vi "ERT_ver2_9_7.vi"() -> ()   [LabVIEW 2023]
uses:
  <vilib>/Utility/error.llb/DialogType.ctl
  <vilib>/Utility/file.llb/Read Delimited Spreadsheet (string).vi
  <vilib>/Utility/file.llb/Read Delimited Spreadsheet (I64).vi
  <vilib>/Utility/config.llb/Read Key (Boolean).vi
  <vilib>/Utility/config.llb/Read Key (U32).vi
  <vilib>/Utility/config.llb/Read Key (Double).vi
  <vilib>/Utility/config.llb/Read Key (I32).vi
  <vilib>/Utility/config.llb/Read Key (String).vi
  <vilib>/Instr/_visa.llb/VISA Configure Serial Port (Instr).vi
  <vilib>/Utility/file.llb/Write Delimited Spreadsheet (I64).vi
  <vilib>/Utility/file.llb/Write Delimited Spreadsheet (string).vi
  <vilib>/Utility/file.llb/Write Delimited Spreadsheet (DBL).vi
  <vilib>/Utility/config.llb/Write Key (Boolean).vi
  <vilib>/Utility/config.llb/Write Key (U32).vi
  <vilib>/Utility/config.llb/Write Key (Double).vi
  <vilib>/Utility/config.llb/Write Key (I32).vi
  <vilib>/Utility/config.llb/Write Key (String).vi
  <vilib>/regexp/Match Regular Expression.xnode
  <instrlib>/Agilent 3446X Series/Agilent 3446X Series.lvlib
  <vilib>/Utility/config.llb/NI_LVConfig.lvlib
panel:
  out "State temp":string
  out "Period for one sample":i32
  out "ESP32 connect?":bool
  out "Current Sense \nResitance Array":dbl[](array[numeric])=[1.0032214, 1.00250644, 1.00234822, 1.0040944, 1.0017711, 1.00229431, 1.00344206, 1.00482066, 1.00381056, 1.00290978, 1.00333016, 1.00367587]
  out "channel count":i32
  out "State":string
  in  "Leave":bool
  in  "Tab Control":T1(tab)
  in  "Refresh":bool
  in  "DMM VISA":refnum<visa-resource-name> caption="DMM (34465A,34470A)"
  in  "ESP32 VISA":refnum<visa-resource-name> caption="ESP32"
  in  "Tab_Current Mode":T2(tab)
  in  "Current Set":u8[][](array[numeric])
  in  "Upload\nCurrent\nSet \nMode":bool
  in  "Current Set Mode":string[][](array[string])
  in  "Break Period Multipier":dbl=8.0
  in  "Insert\nBreak":bool
  in  "Inverse\nPolarity":bool=TRUE
  in  "Electrode number, N":u16=8
  in  "Array Mode":u16(ring) items=["None", "Gradient + Dipole dipole", "Gradient", "Dipole Dipole", "Schlumberger"]
  in  "Upload\nArray":bool
  in  "Only Use Last Value?":bool=TRUE
  in  "Current Channel":string
  in  "Current Mode":u8[][](array[numeric])=[[1, 2, 0, 0, 0, 0, 0, 0], [2, 1, 0, 0, 0, 0, 0, 0], [0, 0, 1, 2, 0, 0, 0, 0], [0, 0, 2, 1, 0, 0, 0, 0], [0, 0, 0, 0, 1, 2, 0, 0], [0, 0, 0, 0, 2, 1, 0, 0], [0, 0, 0, 0, 0, 0, 1, 2], [0, 0, 0, 0, 0, 0, 2, 1]]
  in  "Clear Current Mode":bool
  in  "Waiting\nTime":u32=100 caption="Waiting Time(mS)"
  in  "Sample Mode":u16(ring) items=["Normal", "Interlanced", "Serial", "Seperated Serial"]
  in  "Sample Number":i32=4
  in  "Switch On Time":u8=100 caption="Switch On Time(uS)"
  in  "Switch Off Time":u8=100 caption="Switch Off Time(uS)"
  in  "safe Mode?":bool=TRUE
  in  "PSU Buffer Time":u32=100 caption="PSU Buffer\nTime (ms)"
  in  "Save\nRaw Data":bool=TRUE
  in  "PSU Enable":bool
  in  "Output Max Current":dbl=0.1 caption="Max Current"
  in  "Output Max Voltage":dbl=100.0 caption="Max Voltage"
  in  "Measure\nMax Voltage":dbl=100.0
  in  "Current period":u32=2000
  in  "Scan Period":u32=100
  in  "Sample Measure\nTime(uS)":i32=100
  in  "Scan Number":u32=10
  in  "Constant Scan Number":bool=TRUE
  in  "Neglect\nTimeout Data":bool=TRUE
  in  "Enable Accurate \nMeasure":bool=TRUE
  in  "Enable DMM\n Relay":bool
  in  "Measure Current \nOnly":bool=TRUE
  in  "Record Accurate \nData Only":bool=TRUE
  in  "Remote\nPSU":bool
  in  "PSU(9184B)":refnum<visa-resource-name>="COM5" caption="PSU (9184B,9185B)"
  in  "Email Setting":T3={"server address"="smtp.gmail.com:587", "from"="ncuccc45002931@gmail.com", "username"="ncuccc45002931", "APP password"="aiwfjsidudnfefes\n", "Receiver Email"="yehtingo@gmail.com", "subject"="ERT_data_", "message"="it worked.", "Attach data?"=TRUE}
  in  "Send data\nAutomatically":bool=TRUE
  in  "Leave Timer":string
  in  "Scan Start Timer":string[](array[string])
  in  "Current min":dbl=0.1
  in  "Voltage min":dbl=0.1
  out "Current channel\nindex":string[](array[string])=["  ", "  "]
  in  "I":bool
  in  "V":bool
  in  "Scan Stop":bool
  in  "Scan start":bool
  out "XY Graph":cluster{dbl[], dbl[]}[](graph)
  in  "plot setting":T4(array[cluster])
  in  "Enable\nPlot":bool=TRUE
  in  "Auto Plot \nCurrent":bool
  in  "Current max":dbl=0.1
  in  "Voltage max":dbl=10.0
  out "Data Directory":path=path "C:/Users/User/Desktop/test.csv"
  out "Time out count:":i32
  in  "Data Directory":bool
  out "PSU V":string
  out "PSU I":string
  in  "Measured Current Sense Resistivity":i32[](listbox)
  in  "Update Resistivity":bool
  in  "Calibrate start":bool
  in  "Calibrate Stop":bool
  in  "Current Sense Resistivity List":i32[](listbox) caption="Current Sense Resistivity"
  out "Measured Current Sense \nResitance Array":dbl[](array[numeric])=[1.0032214, 1.00250644, 1.00234822, 1.0040944, 1.0017711, 1.00229431, 1.00344206, 1.00482066, 1.00381056, 1.00290978, 1.00333016, 1.00367587]
  in  "Wait Current Stable Period":i32=500
  in  "Resistance Test":i32[](listbox)
  in  "Resistance Test start":bool
  in  "Resistance Test Stop":bool
  in  "External\nPSU":bool
  in  "Tab Control 2":enum32{"R2 Format Covert"}(tab)
  in  "Conver Type:":T5(radio)
  in  "Original Data path":path
  in  "R2 format covert":bool
  in  "Modified Data path":path
  in  "R2 format_Scan number":i32=10 caption="Scan number"
  in  "Current set number in one current mode":i32=48 caption="Current Mode Number in One Current Set"
  out "concatenated string 3":string caption="concatenated string"
  # "W."
  # "No."
  # "Ch."
  # "No."
  # "Ch."
  # "No."
  # "Ch."
  # "min"
  # "min"
  # "+ channel:"
  # "¡V   channel:"
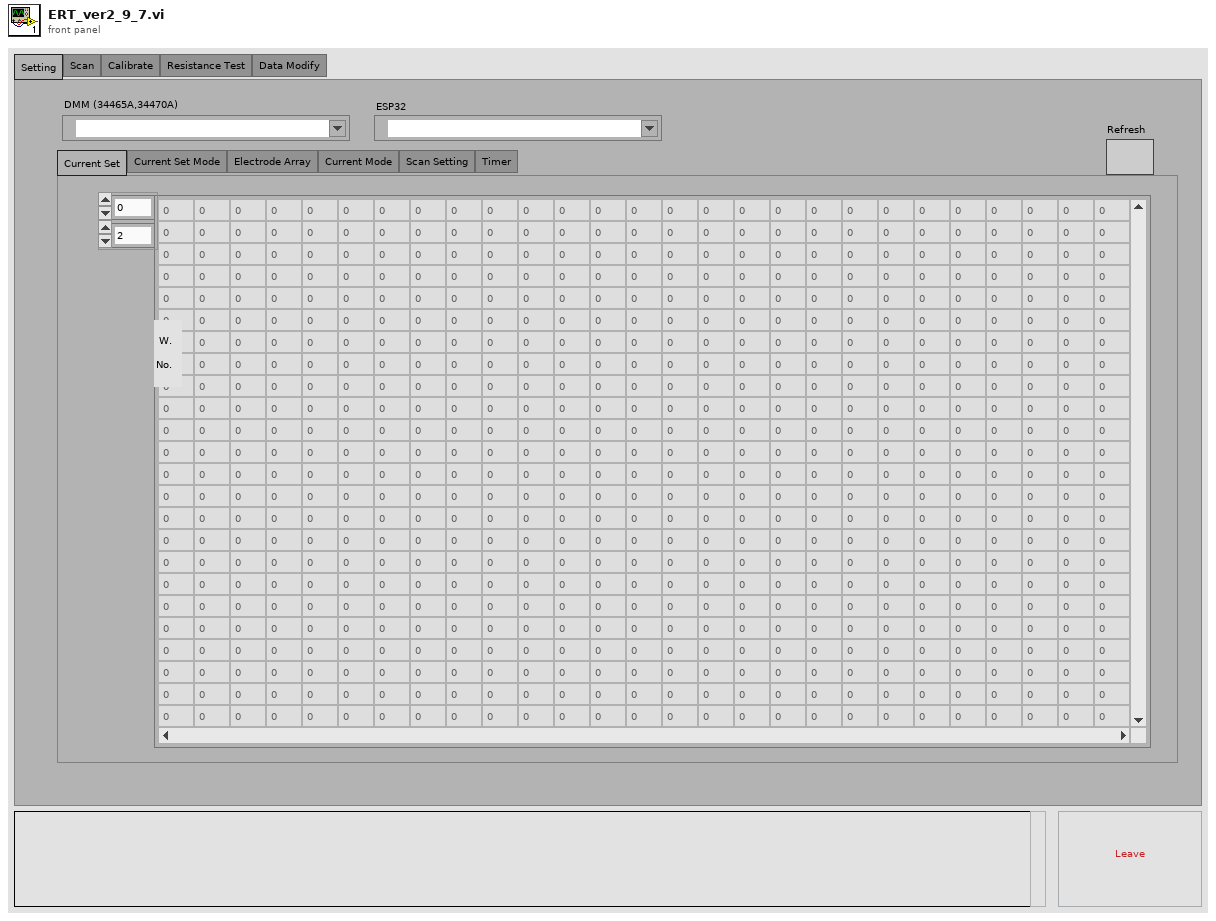
[diagram p1: front panel]
types:
  T1 = enum32{"Setting", "Scan", "Calibrate", "Resistance Test", "Data Modify"}
  T2 = enum32{"Current Set", "Current Set Mode", "Electrode Array", "Current Mode", "Scan Setting", "Timer"}
  T3 = cluster{"server address":string, "from":string, "username":string, "APP password":string, "Receiver Email":string, "subject":string, "message":string, "Attach data?":bool}
  T4 = cluster{"V plot":bool, "I plot":bool, "Plot colour":u32, "Channel name\n":string}[]
  T5 = enum32{"Filled", "Filled and splitted", "Regular"}
  T6 = typedef "DialogType.ctl" = u16
  T7 = enum8{"Enabled", "Disabled", "Disabled and Grayed Out"}
  T8 = typedef "NI_LVConfig.lvlib/Config Data RefNum.ctl" = refnum<k1>
  T9 = cluster{"Enable DMM\n Relay":bool, "Measure Current \nOnly":bool, dbl[], i32}
  T10 = cluster{"value":string, "value":string, "value":string, "value":string, "value":string, "value":string, "value":string, "value":bool}
  T11 = cluster{"DMM VISA":refnum<visa-resource-name>, "ESP32 VISA":refnum<visa-resource-name>, "Scan Period":u32, "Current period":u32, "Scan Measure\nTime(uS)":i32, "Measure\nMax Voltage":dbl, "Data Directory":path, "Voltage max":dbl, "Voltage min":dbl, "Current max":dbl, "Current min":dbl, "PSU(9184B)":refnum<visa-resource-name>}
  T12 = cluster{"Remote\nPSU":bool, "PSU(9184B)":refnum<visa-resource-name>, "Output Max Voltage":dbl, "Output Max Current":dbl, "PSU Buffer Time":u32}
  T13 = cluster{"DMM VISA":refnum<visa-resource-name>, "ESP32 VISA":refnum<visa-resource-name>, "Scan Period":u32, "Current period":u32, "Sample Measure\nTime(uS)":i32, "Measure\nMax Voltage":dbl, "Data Directory":path, "Voltage max":dbl, "Voltage min":dbl, "Current max":dbl, "Current min":dbl, "PSU(9184B)":refnum<visa-resource-name>}
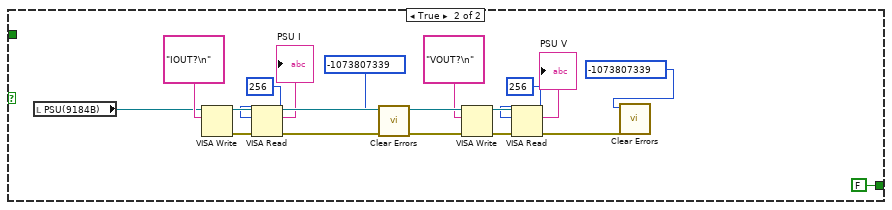
[diagram p3: hidden frame]
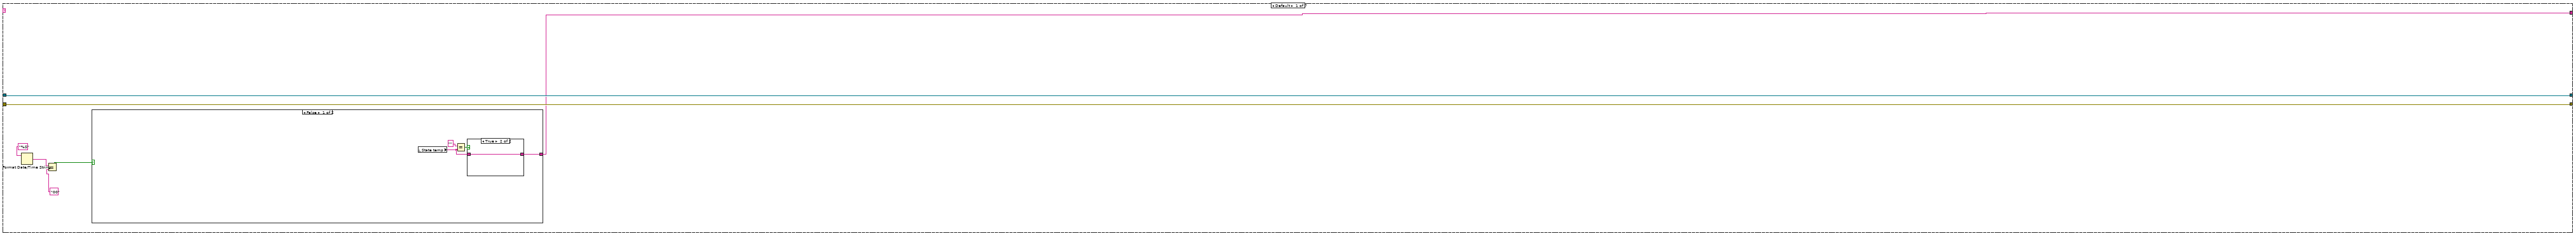
[diagram p4: hidden frame]
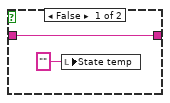
[diagram p5: hidden frame]
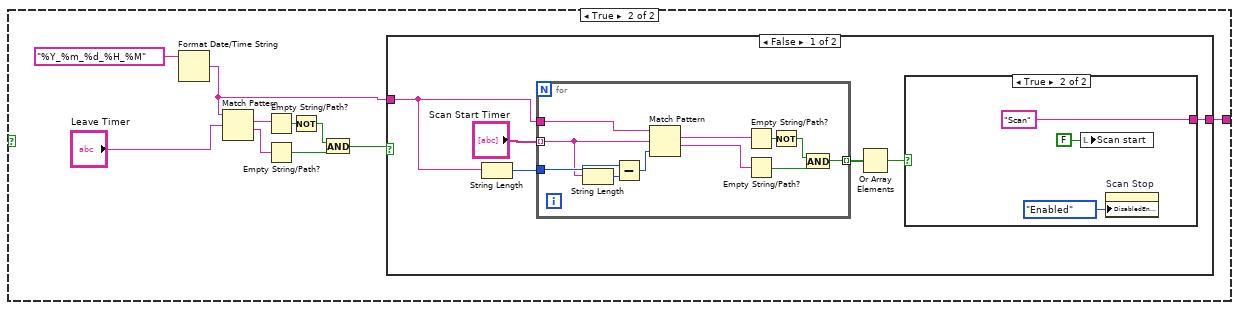
[diagram p6: hidden frame]
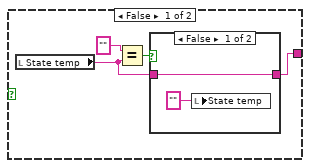
[diagram p7: hidden frame]
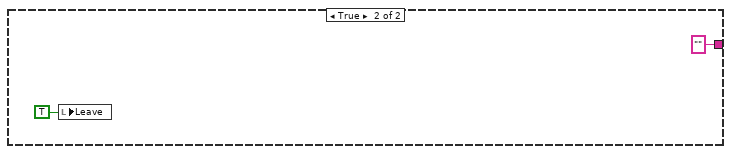
[diagram p9: hidden frame]
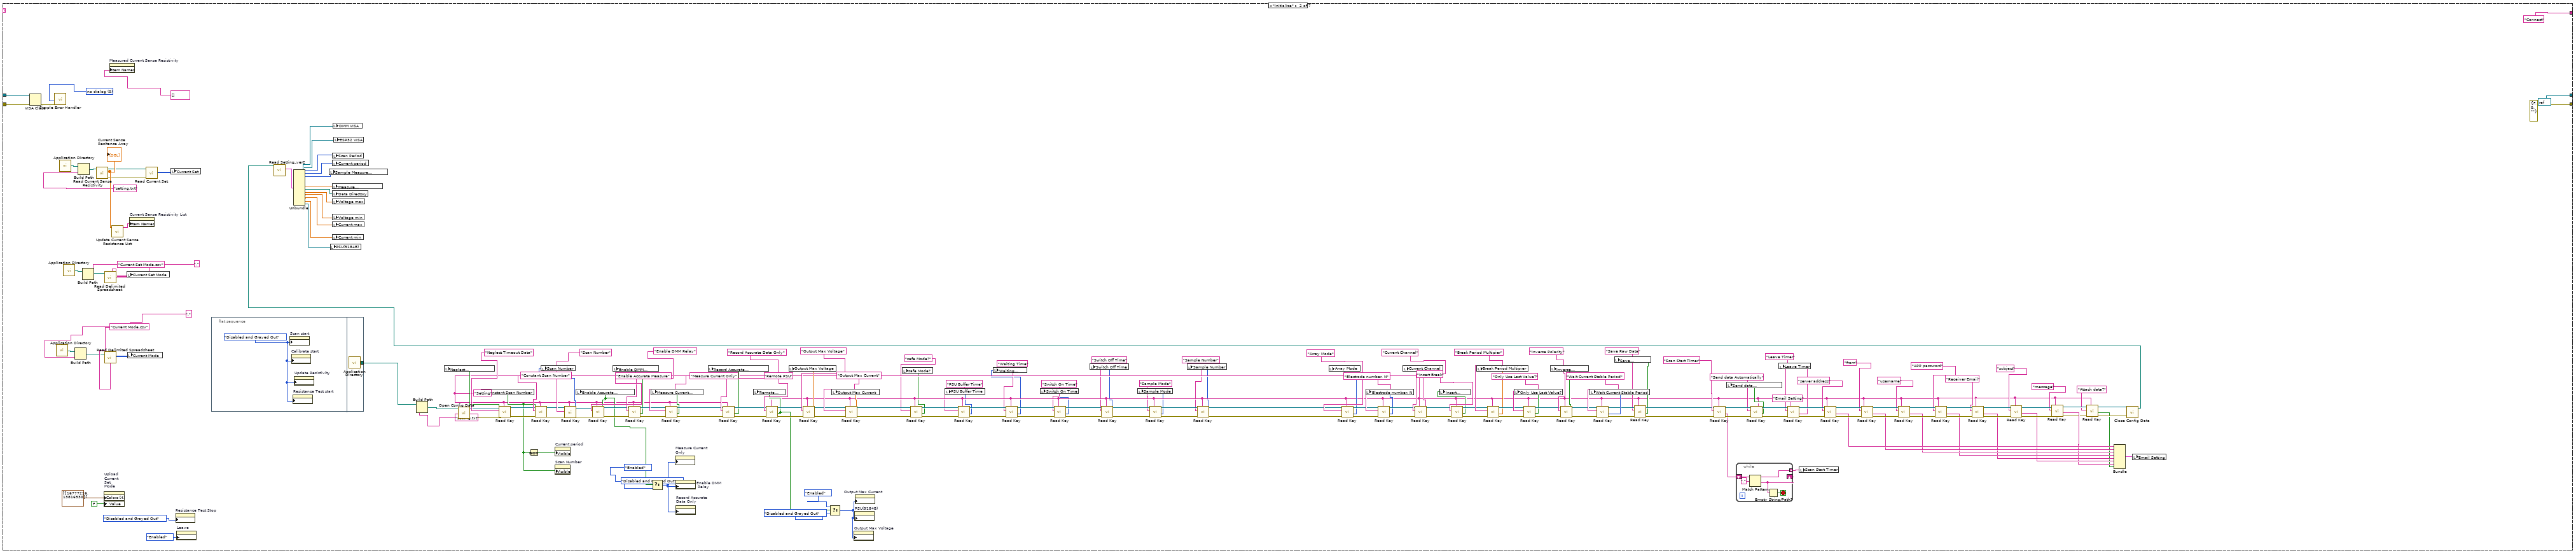
[diagram p10: hidden frame]
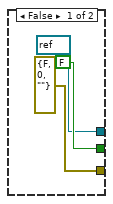
[diagram p11: hidden frame]
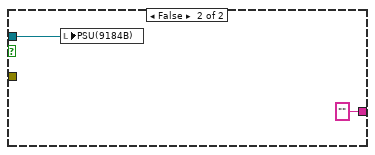
[diagram p12: hidden frame]
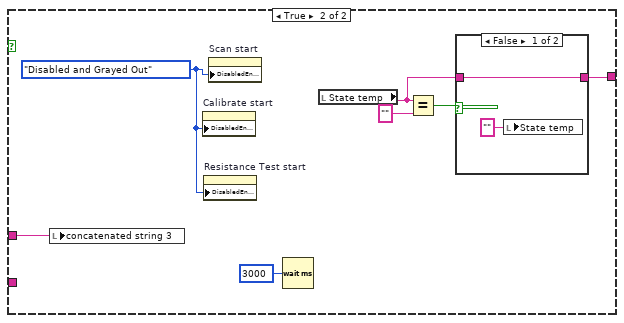
[diagram p13: hidden frame]
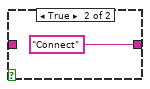
[diagram p14: hidden frame]
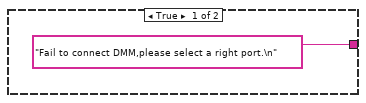
[diagram p15: hidden frame]
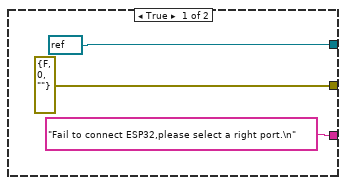
[diagram p16: hidden frame]
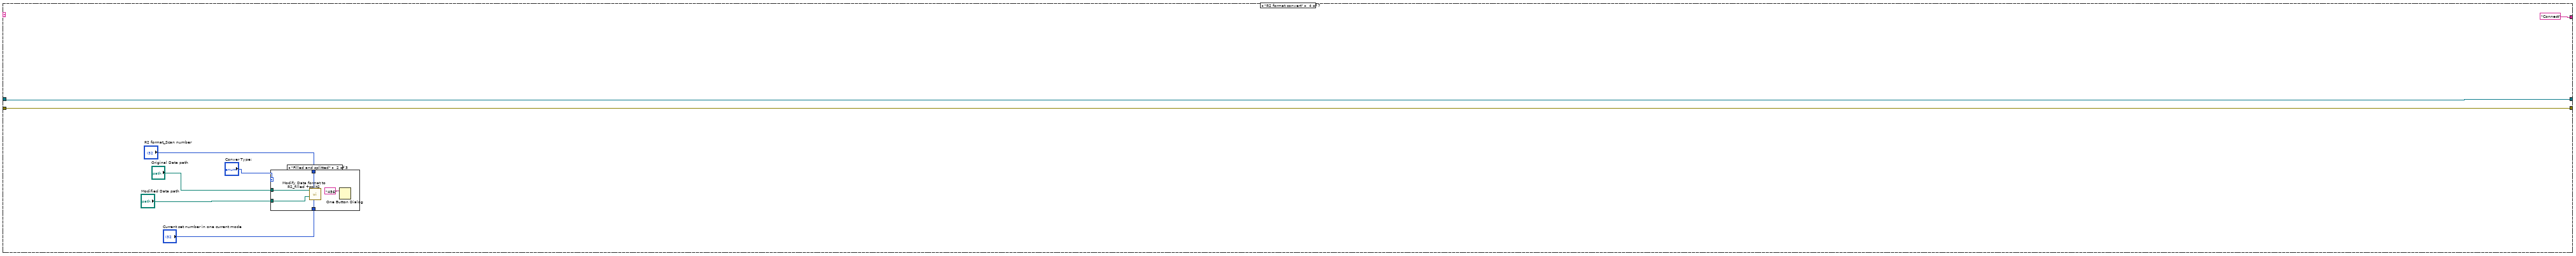
[diagram p17: hidden frame]
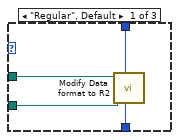
[diagram p18: hidden frame]
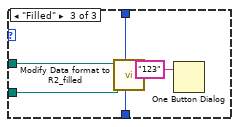
[diagram p19: hidden frame]
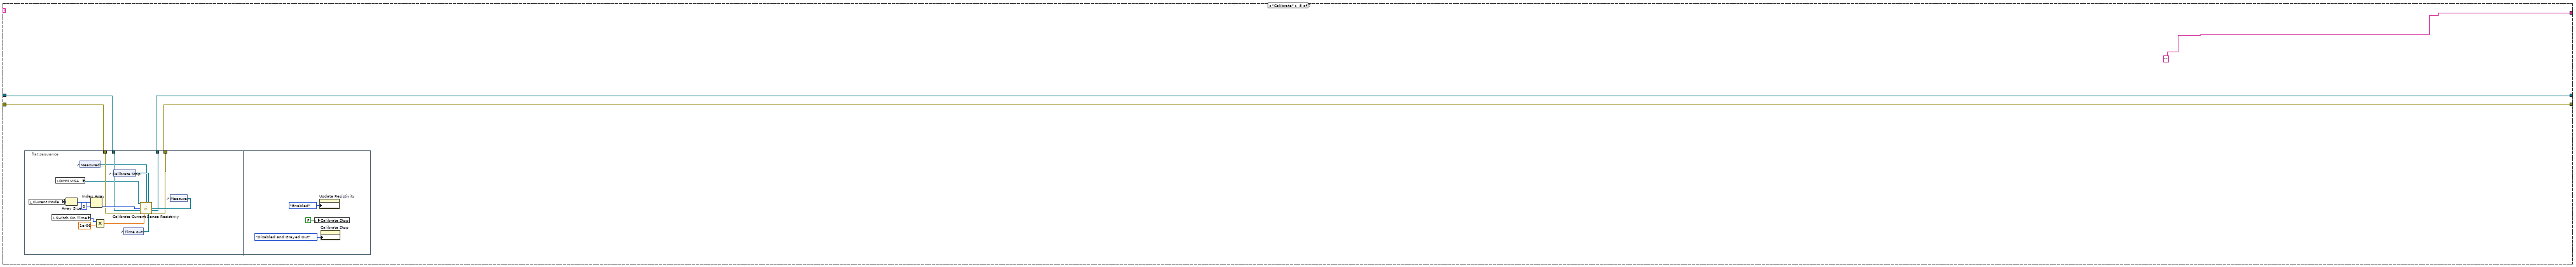
[diagram p20: hidden frame]
diagram:
  w2 = T6 0 items=["no dialog", "OK message", "continue or stop message", "OK message + warnings", "continue/stop + warnings"] ("type of dialog (OK msg:1)")
  # "Oscilloscope mode?"
  # "2_9 2024/1/18\n1. add Oscilloscope mode\n2. add command 'L' to turn\nESP32 into high Impedance\nso it can be parallel with other\ndevice."
  # "2_8 2024/1/9\n1. enable setting switch on \n,off time  and trigger time\n2.. add \"super sample\""
  # "2_7 2024/1/2\n1. add safe PSU mode\n(turn off output of PSU while switching \ncurrent mode)"
  # "ver2_6\n1. add email"
  # "ver2_5 2023/12/19\n1. add scan timer"
  # "ver2_4 2023/12/14\n1.add reconnect when timeout count\nreach 10000"
  # "ver2_3 2023/12/5\n1.updata modify after ver16\n2.add resistance test by DMM"
  # "Board ver2.\nconnect Vpsu from DMM+ to DMM-"
  # "Board ver1."
  # "ver16 2023/08/02\n1. PSU(9184B) connect (optionnal)"
  # "ver15 2023/07/31\n1. Connect COM before scan.\n2. add \"Test\" procedure"
  # "ver14 2023/06/28\n1. add scan mode \"constant scan number\"\n2. add option neglect timeout data\n3. option that modify to R2 format in the end\n4. add option to plot specific  min value"
  # "ver13 2023/06/17\n1.display current channel\nwhile scanning\n2. modify current mode in data when\nfinishing the scan"
  # "try timeout minimum\nwill the timeout in scan\nbe shorter?\nor just set this value to \nscan period minus 10?"
  # "ver12 2023/06/13\n1. main system\n2.edit current mode\n3. measure current with calbrated\ncurrent sense resistor\n4.  add command 's' before scan"
  # "ver11 2023/06/11\n1. record accurate measure only\n2. measure accurate current only"
  # "ver10 2023/06/06\n1.combine subVI and ploting\n2.set plot interpolation to 2 just like default,\nor it will causing more than 50mS when\nX scale change with 64 channels, rather than\n6mS, I think that is some kind of bug in\nlabview.\n3.because of previous changing, I need to \nrecord time \"after\" finising measure, so it can\nproperly display how long it take to finish\naccurate measure.\n4.save data when data index is between 2~3\nplot width"
  n1 = local read "Current Mode"() -> (w21:u8[][])
  n2 = local write "Leave"(FALSE ("Leave")) -> ()
  n3 = Array Size(array=w21) -> (size(s)=w20:i32[])
  n4 = Index Array(array=w20, index=0) -> (element=→"channel count":i32)
  n5 = local write "ESP32 connect?"(FALSE ("ESP32 connect?")) -> ()
  n6 = control-ref of="plot setting"() -> (w23:refnum<vi>)
  n7 = control-ref of="XY Graph"() -> (w22:refnum<vi>)
  n8 = while {
    tunnel: w23 -> [w26]
    tunnel: w22 -> [w25]
    stop <- w27 stop-if-true
    n9 = event shown="[1] \"Leave\": Value Change" {
      selector: _ -> [_ _ _ _ _ _ _ _ _ _ _ _ _ _ _ _ _ _ _ _ _ _ _ _ _ _ _ _ _ _ _ _ _ _ _ _ _ _ _ _ _]
      dyn-events: _ -> [_ _ _ _ _ _ _ _ _ _ _ _ _ _ _ _ _ _ _ _ _ _ _ _ _ _ _ _ _ _ _ _ _ _ _ _ _ _ _ _ _]
      timeout: 1000 -> [_ _ _ _ _ _ _ _ _ _ _ _ _ _ _ _ _ _ _ _ _ _ _ _ _ _ _ _ _ _ _ _ _ _ _ _ _ _ _ _ _]
      tunnel: [w28 w32 _ _ _ _ _ _ _ _ _ _ _ _ _ _ _ _ _ _ _ _ _ _ _ _ _ _ _ _ _ _ _ _ _ _ _ _ _ _ _] -> w27
      tunnel: w26 -> [_ _ _ _ _ _ _ _ _ _ _ _ _ _ _ _ _ w160 w166 w170 _ _ _ _ _ _ _ _ _ _ _ _ _ _ _ _ _ _ _ _ _]
      tunnel: w25 -> [_ _ _ _ _ _ _ _ _ _ _ _ _ _ _ _ _ w159 w165 w169 _ w179 w192 w205 w218 _ _ _ _ _ _ _ _ _ _ _ _ _ _ _ _]
      event Timeout {
        n10 = event-data() -> ()  [unwired: 1 in, 3 out]
        n11 = local read "Leave"() -> (w29:bool)
        n12 = local read "State"() -> (w30:string)
        n13 = Empty String/Path?(string/path=w30) -> (empty?=w31:bool)
        n14 = And(x=w31, y=w29) -> (x .and. y?=w28:bool)
      }
      event "Leave": Value Change {
        n15 = event-data() -> ("NewVal"=w32:bool)  [unwired: 1 in, 5 out]
      }
      event "Scan start": Value Change {
        n16 = event-data() -> ("NewVal"=w33:bool)  [unwired: 1 in, 5 out]
        n17 = case shown="True" w33 {
          frame False {
          }
          frame True {
            n18 = local write "Scan start"(FALSE ("Scan start")) -> ()
            n19 = local write "State temp"("Scan" ("State")) -> ()
            n20 = property on="Scan Stop" class="Bool (strict)"("DisabledEnum"=T7."Enabled" ("Disabled")) -> ()  [unwired: 2 in, 2 out]
          }
        }
      }
      event "Resistance Test start": Value Change {
        n21 = event-data() -> ("NewVal"=w37:bool)  [unwired: 1 in, 5 out]
        n22 = case shown="True" w37 {
          frame False {
          }
          frame True {
            n23 = local read "External\nPSU"() -> (w38:bool)
            n24 = case shown="True" w38 {
              tunnel: ["Resistance Test" ("State") w51] -> w39
              frame False {
              }
              frame True {
                n25 = local read "Remote\nPSU"() -> (w49:bool)
                n26 = Two Button Dialog(message="WARNING!!!!!\nMake sure  \"Measure max voltage\" in \"Scan Setting\"\nis higher than the voltage output from PSU,\nor you might damage your DMM.", 1:"Yes, I certainly have." ("T button name (\"OK\")"), 2:"Not Sure, check again" ("F button name (\"Cancel\")")) -> (T button?=w45:bool)
                n27 = Not(x=w45) -> (.not. x?=w44:bool)
                n28 = And(x=w49, y=w44) -> (x .and. y?=w46:bool)
                n29 = case shown="True" w46 {
                  tunnel: [FALSE ("T button?") w57] -> w47
                  frame False {
                  }
                  frame True {
                    n30 = local read "Output Max Voltage"() -> (w61:dbl)
                    n31 = Number To Decimal String(number=w61) -> (decimal integer string=w62:string)  [unwired: 1 in]
                    n32 = Concatenate Strings("WARNING!!!!!\nMake sure your loading can endure\n\"Max Voltage\" output( " ("message"), w62, " V)from PSU in \"Scan Setting " ("message")) -> (w58:string)
                    n33 = Two Button Dialog(message=w58, 1:"Yes, I certainly have." ("T button name (\"OK\")"), 2:"Not Sure, check again" ("F button name (\"Cancel\")")) -> (T button?=w57:bool)
                  }
                }
                n34 = Or(x=w45, y=w47) -> (x .or. y?=w48:bool)
                n35 = Select(t="" ("f"), s=w48, f="Resistance Test" ("State")) -> (s? t:f=w51:string)
              }
            }
            n36 = local write "Resistance Test Stop"(FALSE ("Resistance Test Stop")) -> ()
            n37 = property on="Resistance Test Stop" class="Bool (strict)"("DisabledEnum"=T7."Enabled" ("Disabled")) -> ()  [unwired: 2 in, 2 out]
            n38 = local write "Resistance Test start"(FALSE ("Scan start")) -> ()
            n39 = local write "State temp"(w39) -> ()
          }
        }
      }
      event "Remote\nPSU": Value Change {
        n40 = event-data() -> ("NewVal"=w68:bool)  [unwired: 1 in, 5 out]
        n41 = Select(t=T7."Enabled" ("Disabled"), s=w68, f=T7."Disabled and Grayed Out" ("Disabled")) -> (s? t:f=w66:T7)
        n42 = property on="Output Max Voltage" class="DigNum (strict)"("DisabledEnum"=w66) -> ()  [unwired: 2 in, 2 out]
        n43 = property on="PSU(9184B)" class="VISAName"("DisabledEnum"=w66) -> ()  [unwired: 2 in, 2 out]
        n44 = property on="Output Max Current" class="DigNum (strict)"("DisabledEnum"=w66) -> ()  [unwired: 2 in, 2 out]
        n45 = local write "State"("Connect" ("State")) -> ()
      }
      event "R2 format covert": Value Change {
        n46 = event-data() -> ("NewVal"=w70:bool)  [unwired: 1 in, 5 out]
        n47 = case shown="True" w70 {
          frame False {
          }
          frame True {
            n48 = flat-sequence {
              frame #0 {
                n49 = local read "Original Data path"() -> (w71:path)
                n50 = Empty String/Path?(string/path=w71) -> (empty?=w72:bool)
                n51 = case shown="True" w72 {
                  frame False {
                  }
                  frame True {
                    n52 = call "File Dialog2"() -> ("selected path"=w73:path)  [unwired: 12 in, 3 out]
                    n53 = Strip Path(path=w73) -> (stripped path=w78:path, name=w77:string)
                    n54 = local write "Original Data path"(w73) -> ()
                    n55 = Concatenate Strings("Modified_" ("string"), w77) -> (w76:string)
                    n56 = Build Path(base path=w78, name or relative path=w76) -> (appended path=w75:path)
                    n57 = local write "Modified Data path"(w75) -> ()
                  }
                }
              }
              frame #1 {
                n58 = local write "R2 format covert"(FALSE ("Scan start")) -> ()
                n59 = local write "State temp"("R2 format convert" ("State")) -> ()
              }
            }
          }
        }
      }
      event "Calibrate start": Value Change {
        n60 = event-data() -> ("NewVal"=w82:bool)  [unwired: 1 in, 5 out]
        n61 = case shown="True" w82 {
          frame False {
          }
          frame True {
            n62 = Two Button Dialog(message="WARNING!!!!!\nMake sure you have replace PSU+ pin to DMM I-\nor your machine might BLOW!!!!!\n", 1:"Yes, I certainly have." ("T button name (\"OK\")"), 2:"Not Sure, check again" ("F button name (\"Cancel\")")) -> (T button?=w89:bool)
            n63 = local write "Calibrate start"(FALSE ("Scan start")) -> ()
            n64 = Select(t="" ("f"), s=w89, f="Calibrate") -> (s? t:f=w90:string)
            n65 = local write "State temp"(w90) -> ()
          }
        }
        n66 = property on="Calibrate Stop" class="Bool (strict)"("DisabledEnum"=T7."Enabled" ("Disabled")) -> ()  [unwired: 2 in, 2 out]
      }
      event "Data Directory": Value Change {
        n67 = event-data() -> ("NewVal"=w91:bool)  [unwired: 1 in, 5 out]
        n68 = case shown="True" w91 {
          frame False {
          }
          frame True {
            n69 = call "File Dialog"() -> ("selected path"=→"Data Directory":path)  [unwired: 12 in, 3 out]
            n70 = local write "Data Directory"(FALSE ("Data Directory")) -> ()
          }
        }
      }
      event "Update Resistivity": Value Change {
        n71 = event-data() -> ("NewVal"=w97:bool)  [unwired: 1 in, 5 out]
        n72 = local read "State"() -> (w99:string)
        n73 = Equal?(x=w99, y="") -> (x = y?=w96:bool)
        n74 = And(x=w96, y=w97) -> (x .and. y?=w95:bool)
        n75 = case shown="True" w95 {
          tunnel: [FALSE ("Scan start") FALSE ("Scan start")] -> w94
          frame False {
          }
          frame True {
            n76 = local read "Measured Current Sense \nResitance Array"() -> (w107:dbl[])
            n77 = property on="Measured Current Sense Resistivity" class="LstBox (strict)"() -> ("Value"=w106:i32[])  [unwired: 2 in, 2 out]
            n78 = for {
              tunnel: w106 -> [w109] mode=indexing
              tunnel: w107 -> [w115]
              tunnel: [w113] -> w104
              n79 = local read "Current Sense \nResitance Array"() -> (w110:dbl[])
              n80 = Index Array(array=w115, index=w109) -> (element=w114:dbl)
              n81 = Array Size(array=w110) -> (size(s)=w111:i32)
              n82 = Less?(x=w109, y=w111) -> (x < y?=w112:bool)
              n83 = case shown="False" w112 {
                tunnel: w110 -> [w121 w127]
                tunnel: w114 -> [w118 w126]
                tunnel: w109 -> [w119 w125]
                tunnel: [w117 w124] -> w113
                frame False {
                  n84 = Increment(x=w119) -> (x+1=w116:i32)
                  n85 = Initialize Array(0.0 ("element"), w116) -> (w122:dbl[])
                  n86 = Replace Array Subset(array=w122, new element=w121) -> (w120:dbl[])  [unwired: 1 in]
                  n87 = Replace Array Subset(array=w120, new element=w118, index=w119) -> (w117:dbl[])
                }
                frame True {
                  n88 = Replace Array Subset(array=w127, new element=w126, index=w125) -> (w124:dbl[])
                }
              }
              n89 = local write "Current Sense \nResitance Array"(w113) -> ()
            }
            n90 = call <vilib>:"Application Directory.vi"() -> ("Application Directory"=w103:path)
            n91 = Build Path(base path=w103, name or relative path="setting.txt") -> (appended path=w101:path)
            n92 = call "Updata Current Sense Resistance List.vi"("Array in"=w104) -> ("Array out"=w105:string[])  [unwired: 10 in]
            n93 = property on="Current Sense Resistivity List" class="LstBox (strict)"("Item Names"=w105) -> ()  [unwired: 2 in, 2 out]
            n94 = call "Write Current Sense Resistivity.vi"("Array"=w104, "configuration file path"=w101) -> ()  [unwired: 8 in, 2 out]
          }
        }
        n95 = local write "Update Resistivity"(w94) -> ()
      }
      event "Current Set": Value Change {
        n96 = event-data() -> ()  [unwired: 1 in, 6 out]
        n97 = property on="Upload\nCurrent\nSet \nMode" class="Bool (strict)"("DisabledEnum"=T7."Enabled" ("Disabled")) -> ()  [unwired: 2 in, 2 out]
      }
      event "Upload\nCurrent\nSet \nMode": Value Change {
        n98 = event-data() -> ("NewVal"=w129:bool)  [unwired: 1 in, 5 out]
        n99 = case shown="True" w129 {
          frame False {
          }
          frame True {
            n100 = local read "Current Set Mode"() -> (w132:string[][])
            n101 = local read "Current Set"() -> (w133:u8[][])
            n102 = call "Updata Current Mode.vi"("Current Set Mode"=w132, "Current Set"=w133) -> ("Current Mode"=w131:u8[][])  [unwired: 9 in]
            n103 = property on="Upload\nCurrent\nSet \nMode" class="Bool (strict)"("Colors [4]"=cluster{u32, u32}[] [{16777216, 13816530}], "Value"=FALSE ("Upload\nCurrent\nSet \nMode")) -> ()  [unwired: 2 in, 2 out]
            n104 = local write "Current Mode"(w131) -> ()
          }
        }
      }
      event "Upload\nArray": Value Change {
        n105 = event-data() -> ("NewVal"=w135:bool)  [unwired: 1 in, 5 out]
        n106 = case shown="True" w135 {
          frame False {
          }
          frame True {
            n107 = One Button Dialog(message="Updata completed") -> ()  [unwired: 1 in, 1 out]
            n108 = call "Create Electrode Array_2.vi"("Current Channel"="Current Channel", "Insert\nBreak"="Insert\nBreak", "Inverse\nPolarity"="Inverse\nPolarity", "Electrode number, N"="Electrode number, N", "Array Mode"="Array Mode") -> ("Current Mode"=w138:u8[][])  [unwired: 6 in]
            n109 = local write "Current Mode"(w138) -> ()
            n110 = property on="Upload\nArray" class="Bool (strict)"("Colors [4]"=cluster{u32, u32}[] [{16777216, 13816530}]) -> ()  [unwired: 2 in, 2 out]
            n111 = local write "Upload\nArray"(FALSE ("Upload\nArray")) -> ()
          }
        }
      }
      event "Break Period Multipier": Value Change {
        n112 = event-data() -> ("NewVal"=w146:dbl)  [unwired: 1 in, 5 out]
        n113 = Absolute Value(x=w146) -> (abs(x)=w145:dbl)
        n114 = local write "Break Period Multipier"(w145) -> ()
      }
      event "Clear Current Mode": Value Change {
        n115 = event-data() -> ("NewVal"=w147:bool)  [unwired: 1 in, 5 out]
        n116 = case shown="True" w147 {
          frame False {
          }
          frame True {
            n117 = local write "Clear Current Mode"(FALSE ("Clear Current Mode")) -> ()
            n118 = local write "Current Mode"(i32[][] [] ("Current Mode")) -> ()
          }
        }
      }
      event "Refresh": Value Change {
        n119 = event-data() -> ("NewVal"=w150:bool)  [unwired: 1 in, 5 out]
        n120 = case shown="True" w150 {
          frame False {
          }
          frame True {
            n121 = local write "State temp"("Initialize" ("State")) -> ()
            n122 = local write "Refresh"(FALSE ("Refresh")) -> ()
          }
        }
      }
      event "Current Set Mode": Value Change {
        n123 = event-data() -> ()  [unwired: 1 in, 6 out]
        n124 = property on="Upload\nCurrent\nSet \nMode" class="Bool (strict)"("Colors [4]"=cluster{u32, u32}[] [{16711680, 13816530}]) -> ()  [unwired: 2 in, 2 out]
      }
      event "Enable Accurate \nMeasure": Value Change {
        n125 = event-data() -> ("NewVal"=w157:bool)  [unwired: 1 in, 5 out]
        n126 = Select(t=T7."Enabled" ("Disabled"), s=w157, f=T7."Disabled and Grayed Out" ("Disabled")) -> (s? t:f=w154:T7)
        n127 = property on="Measure Current \nOnly" class="Bool (strict)"("DisabledEnum"=w154) -> ()  [unwired: 2 in, 2 out]
        n128 = property on="Enable DMM\n Relay" class="Bool (strict)"("DisabledEnum"=w154) -> ()  [unwired: 2 in, 2 out]
        n129 = property on="Record Accurate \nData Only" class="Bool (strict)"("DisabledEnum"=w154) -> ()  [unwired: 2 in, 2 out]
      }
      event "plot setting": Value Change {
        n130 = event-data() -> ("OldVal"=w162:T4, "NewVal"=w161:T4)  [unwired: 1 in, 4 out]
        n131 = local read "channel count"() -> (w158:i32)
        n132 = call "Updata Monitor setting.vi"("Channel number"=w158, "XY Graph REF"=w159, "new plot setting"=w161, "old plot setting"=w162, "plot setting REF"=w160) -> ()  [unwired: 7 in]
      }
      event "V": Value Change {
        n133 = event-data() -> ("NewVal"=w164:bool)  [unwired: 1 in, 5 out]
        n134 = local read "channel count"() -> (w163:i32)
        n135 = call "Plot V.vi"("Channel number"=w163, "XY Graph REF"=w165, "V"=w164, "plot setting REF"=w166) -> ()  [unwired: 8 in]
      }
      event "I": Value Change {
        n136 = event-data() -> ("NewVal"=w168:bool)  [unwired: 1 in, 5 out]
        n137 = local read "channel count"() -> (w167:i32)
        n138 = call "Plot I.vi"("Channel number"=w167, "XY Graph REF"=w169, "V"=w168, "plot setting REF"=w170) -> ()  [unwired: 8 in]
      }
      event "Current Mode": Value Change {
        n139 = event-data() -> ("NewVal"=w172:u8[][])  [unwired: 1 in, 5 out]
        n140 = Array Size(array=w172) -> (size(s)=w174:i32[])
        n141 = Index Array(array=w174, index=0) -> (element=w173:i32)
        n142 = local write "channel count"(w173) -> ()
      }
      event "Current max": Value Change {
        n143 = event-data() -> ("OldVal"=w175:dbl, "NewVal"=w177:dbl)  [unwired: 1 in, 4 out]
        n144 = local read "Current min"() -> (w178:dbl)
        n145 = Less?(x=w178, y=w177) -> (x < y?=w176:bool)
        n146 = case shown="False" w176 {
          tunnel: w179 -> [_ w183]
          tunnel: w177 -> [_ w182]
          tunnel: w175 -> [w181 _]
          frame False {
            n147 = local write "Current max"(w181) -> ()
            n148 = One Button Dialog(message="max value need to be higher than min") -> ()  [unwired: 1 in, 1 out]
          }
          frame True {
            n149 = stacked-sequence {
              tunnel: w183 -> [w184 w187]
              tunnel: w182 -> [_ w186]
              frame #0 {
                n150 = property on="Property Node" class="XYGraph (strict)"(reference=w184, "ActYScl"=1 ("Active Y Scale")) -> ()  [unwired: 1 in, 2 out]
              }
              frame #1 {
                n151 = property on="Property Node" class="XYGraph (strict)"(reference=w187, "YScale.Maximum"=w186) -> ()  [unwired: 1 in, 2 out]
              }
            }
          }
        }
      }
      event "Current min": Value Change {
        n152 = event-data() -> ("OldVal"=w188:dbl, "NewVal"=w189:dbl)  [unwired: 1 in, 4 out]
        n153 = local read "Current max"() -> (w190:dbl)
        n154 = Greater?(x=w190, y=w189) -> (0:w191:bool)
        n155 = case shown="True" w191 {
          tunnel: w192 -> [_ w196]
          tunnel: w189 -> [_ w195]
          tunnel: w188 -> [w194 _]
          frame False {
            n156 = local write "Current min"(w194) -> ()
            n157 = One Button Dialog(message="min value need to be lower than max") -> ()  [unwired: 1 in, 1 out]
          }
          frame True {
            n158 = stacked-sequence {
              tunnel: w196 -> [w197 w200]
              tunnel: w195 -> [_ w199]
              frame #0 {
                n159 = property on="Property Node" class="XYGraph (strict)"(reference=w197, "ActYScl"=1 ("Active Y Scale")) -> ()  [unwired: 1 in, 2 out]
              }
              frame #1 {
                n160 = property on="Property Node" class="XYGraph (strict)"(reference=w200, "YScale.Minimum"=w199) -> ()  [unwired: 1 in, 2 out]
              }
            }
          }
        }
      }
      event "Voltage min": Value Change {
        n161 = event-data() -> ("OldVal"=w201:dbl, "NewVal"=w202:dbl)  [unwired: 1 in, 4 out]
        n162 = local read "Voltage max"() -> (w203:dbl)
        n163 = Greater?(x=w203, y=w202) -> (0:w204:bool)
        n164 = case shown="False" w204 {
          tunnel: w205 -> [_ w209]
          tunnel: w202 -> [_ w208]
          tunnel: w201 -> [w207 _]
          frame False {
            n165 = local write "Voltage min"(w207) -> ()
            n166 = One Button Dialog(message="min value need to be lower than max") -> ()  [unwired: 1 in, 1 out]
          }
          frame True {
            n167 = stacked-sequence {
              tunnel: w209 -> [w210 w213]
              tunnel: w208 -> [_ w212]
              frame #0 {
                n168 = property on="Property Node" class="XYGraph (strict)"(reference=w210, "ActYScl"=0 ("Active Y Scale")) -> ()  [unwired: 1 in, 2 out]
              }
              frame #1 {
                n169 = property on="Property Node" class="XYGraph (strict)"(reference=w213, "YScale.Minimum"=w212) -> ()  [unwired: 1 in, 2 out]
              }
            }
          }
        }
      }
      event "Voltage max": Value Change {
        n170 = event-data() -> ("OldVal"=w214:dbl, "NewVal"=w216:dbl)  [unwired: 1 in, 4 out]
        n171 = local read "Voltage min"() -> (w217:dbl)
        n172 = Less?(x=w217, y=w216) -> (x < y?=w215:bool)
        n173 = case shown="False" w215 {
          tunnel: w218 -> [_ w222]
          tunnel: w216 -> [_ w221]
          tunnel: w214 -> [w219 _]
          frame False {
            n174 = local write "Voltage max"(w219) -> ()
            n175 = One Button Dialog(message="max value need to be higher than min") -> ()  [unwired: 1 in, 1 out]
          }
          frame True {
            n176 = stacked-sequence {
              tunnel: w221 -> [_ w225]
              tunnel: w222 -> [w223 w226]
              frame #0 {
                n177 = property on="Property Node" class="XYGraph (strict)"(reference=w223, "ActYScl"=0 ("Active Y Scale")) -> ()  [unwired: 1 in, 2 out]
              }
              frame #1 {
                n178 = property on="Property Node" class="XYGraph (strict)"(reference=w226, "YScale.Maximum"=w225) -> ()  [unwired: 1 in, 2 out]
              }
            }
          }
        }
      }
      event "Original Data path": Value Change {
        n179 = event-data() -> ("NewVal"=w232:path)  [unwired: 1 in, 5 out]
        n180 = Strip Path(path=w232) -> (stripped path=w231:path, name=w230:string)
        n181 = Concatenate Strings("Modified_" ("string"), w230) -> (w229:string)
        n182 = Build Path(base path=w231, name or relative path=w229) -> (appended path=w227:path)
        n183 = local write "Modified Data path"(w227) -> ()
      }
      event "Constant Scan Number": Value Change {
        n184 = event-data() -> ("NewVal"=w234:bool)  [unwired: 1 in, 5 out]
        n185 = Not(x=w234) -> (.not. x?=w233:bool)
        n186 = property on="Current period" class="DigNum (strict)"("Visible"=w233) -> ()  [unwired: 2 in, 2 out]
        n187 = property on="Scan Number" class="DigNum (strict)"("Visible"=w234) -> ()  [unwired: 2 in, 2 out]
      }
      event "DMM VISA": Value Change {
        n188 = event-data() -> ()  [unwired: 1 in, 6 out]
        n189 = local write "State temp"("Connect" ("State")) -> ()
      }
      event "ESP32 VISA": Value Change {
        n190 = event-data() -> ()  [unwired: 1 in, 6 out]
        n191 = local write "State temp"("Connect" ("State")) -> ()
      }
      event "PSU(9184B)": Value Change {
        n192 = event-data() -> ()  [unwired: 1 in, 6 out]
        n193 = local write "State temp"("Connect" ("State")) -> ()
      }
      event "Array Mode": Value Change {
        n194 = event-data() -> ()  [unwired: 1 in, 6 out]
        n195 = property on="Upload\nArray" class="Bool (strict)"("Colors [4]"=cluster{u32, u32}[] [{16711680, 13816530}]) -> ()  [unwired: 2 in, 2 out]
      }
      event "Electrode number, N": Value Change {
        n196 = event-data() -> ()  [unwired: 1 in, 6 out]
        n197 = property on="Upload\nArray" class="Bool (strict)"("Colors [4]"=cluster{u32, u32}[] [{16711680, 13816530}]) -> ()  [unwired: 2 in, 2 out]
      }
      event "Current Channel": Value Change {
        n198 = event-data() -> ()  [unwired: 1 in, 6 out]
        n199 = property on="Upload\nArray" class="Bool (strict)"("Colors [4]"=cluster{u32, u32}[] [{16711680, 13816530}]) -> ()  [unwired: 2 in, 2 out]
      }
      event "Inverse\nPolarity": Value Change {
        n200 = event-data() -> ()  [unwired: 1 in, 6 out]
        n201 = property on="Upload\nArray" class="Bool (strict)"("Colors [4]"=cluster{u32, u32}[] [{16711680, 13816530}]) -> ()  [unwired: 2 in, 2 out]
      }
      event "Insert\nBreak": Value Change {
        n202 = event-data() -> ()  [unwired: 1 in, 6 out]
        n203 = property on="Upload\nArray" class="Bool (strict)"("Colors [4]"=cluster{u32, u32}[] [{16711680, 13816530}]) -> ()  [unwired: 2 in, 2 out]
      }
      event "Scan Number": Value Change {
        n204 = event-data() -> ("NewVal"=w245:u32)  [unwired: 1 in, 5 out]
        n205 = Less?(x=w245, y=u32 2) -> (x < y?=w243:bool)
        n206 = case shown="True" w243 {
          frame False {
          }
          frame True {
            n207 = local write "Scan Number"(u32 2 ("Scan Number")) -> ()
            n208 = One Button Dialog(message="Scan number need to be at least 2\nor you can use current period mode with 1mS") -> ()  [unwired: 1 in, 1 out]
          }
        }
      }
      event "Scan Start Timer": Value Change {
        n209 = event-data() -> ("NewVal"=w249:string[])  [unwired: 1 in, 5 out]
        n210 = for {
          tunnel: w249 -> [w265] mode=indexing
          shift-right: [w264] -> w248
          shift-left: string[] [] -> [w266]
          shift-right: [w262] -> w259
          shift-left: "" -> [w263]
          n211 = Empty String/Path?(string/path=w265) -> (empty?=w267:bool)
          n212 = case shown="False" w267 {
            tunnel: w266 -> [w273 w275]
            tunnel: w265 -> [w269 _]
            tunnel: [w272 w275] -> w264
            tunnel: w263 -> [w271 w274]
            tunnel: [w270 w274] -> w262
            frame False {
              n213 = Build Array (concatenate)(w273, w269) -> (w272:string[])
              n214 = Concatenate Strings(w271, w269, "," ("string")) -> (w270:string)
            }
            frame True {
            }
          }
        }
        n215 = call <vilib>:"Application Directory.vi"() -> ("Application Directory"=w255:path)
        n216 = Build Path(base path=w255, name or relative path="setting.txt") -> (appended path=w256:path)
        n217 = call <vilib>:"Open Config Data.vi"("configuration file path"=w256) -> ("error out"=w258:errorcluster, "refnum"=w257:T8)  [unwired: 8 in, 1 out]
        n218 = local write "Scan Start Timer"(w248) -> ()
        n219 = call-poly <vilib>:"Write Key.vi"("section"="Setting", "error in (no error)"=w258, "value"=w259, "key"="Scan Start Timer", "refnum"=w257) -> ("error out"=w261:errorcluster, "refnum out"=w260:T8)  [unwired: 4 in, 1 out]
        n220 = call <vilib>:"Close Config Data.vi"("error in (no error)"=w261, "refnum"=w260) -> ()  [unwired: 8 in, 2 out]
      }
      event "Leave Timer": Value Change {
        n221 = event-data() -> ("NewVal"=w276:string)  [unwired: 1 in, 5 out]
        n222 = call <vilib>:"Application Directory.vi"() -> ("Application Directory"=w277:path)
        n223 = Build Path(base path=w277, name or relative path="setting.txt") -> (appended path=w278:path)
        n224 = call <vilib>:"Open Config Data.vi"("configuration file path"=w278) -> ("error out"=w280:errorcluster, "refnum"=w279:T8)  [unwired: 8 in, 1 out]
        n225 = call-poly <vilib>:"Write Key.vi"("section"="Setting", "error in (no error)"=w280, "value"=w276, "key"="Leave Timer", "refnum"=w279) -> ("error out"=w285:errorcluster, "refnum out"=w284:T8)  [unwired: 4 in, 1 out]
        n226 = call <vilib>:"Close Config Data.vi"("error in (no error)"=w285, "refnum"=w284) -> ()  [unwired: 8 in, 2 out]
      }
      event "Send data\nAutomatically": Value Change {
        n227 = event-data() -> ("NewVal"=w286:bool)  [unwired: 1 in, 5 out]
        n228 = call <vilib>:"Application Directory.vi"() -> ("Application Directory"=w290:path)
        n229 = Build Path(base path=w290, name or relative path="setting.txt") -> (appended path=w291:path)
        n230 = call <vilib>:"Open Config Data.vi"("configuration file path"=w291) -> ("error out"=w293:errorcluster, "refnum"=w292:T8)  [unwired: 8 in, 1 out]
        n231 = call-poly <vilib>:"Write Key.vi"("section"="Setting", "error in (no error)"=w293, "value"=w286, "key"="Send data Automatically", "refnum"=w292) -> ("error out"=w295:errorcluster, "refnum out"=w294:T8)  [unwired: 4 in, 1 out]
        n232 = call <vilib>:"Close Config Data.vi"("error in (no error)"=w295, "refnum"=w294) -> ()  [unwired: 8 in, 2 out]
      }
      event "Email Setting": Value Change {
        w298 = "Email Setting" ("section")
        n233 = event-data() -> ("NewVal"=w334:T3)  [unwired: 1 in, 5 out]
        n234 = call <vilib>:"Application Directory.vi"() -> ("Application Directory"=w332:path)
        n235 = Unbundle By Name(w334) -> ("server address"=w309:string, "from"=w308:string, "username"=w307:string, "APP password"=w306:string, "Receiver Email"=w305:string, "subject"=w304:string, "message"=w303:string, "Attach data?"=w297:bool)
        n236 = Build Path(base path=w332, name or relative path="setting.txt") -> (appended path=w333:path)
        n237 = call <vilib>:"Open Config Data.vi"("configuration file path"=w333) -> ("error out"=w329:errorcluster, "refnum"=w330:T8)  [unwired: 8 in, 1 out]
        n238 = call-poly <vilib>:"Write Key.vi"("section"=w298, "error in (no error)"=w329, "value"=w309, "key"="server address", "refnum"=w330) -> ("error out"=w317:errorcluster, "refnum out"=w328:T8)  [unwired: 4 in, 1 out]
        n239 = call-poly <vilib>:"Write Key.vi"("section"=w298, "error in (no error)"=w317, "value"=w308, "key"="from", "refnum"=w328) -> ("error out"=w327:errorcluster, "refnum out"=w326:T8)  [unwired: 4 in, 1 out]
        n240 = call-poly <vilib>:"Write Key.vi"("section"=w298, "error in (no error)"=w327, "value"=w307, "key"="username", "refnum"=w326) -> ("error out"=w325:errorcluster, "refnum out"=w324:T8)  [unwired: 4 in, 1 out]
        n241 = call-poly <vilib>:"Write Key.vi"("section"=w298, "error in (no error)"=w325, "value"=w306, "key"="APP password", "refnum"=w324) -> ("error out"=w323:errorcluster, "refnum out"=w322:T8)  [unwired: 4 in, 1 out]
        n242 = call-poly <vilib>:"Write Key.vi"("section"=w298, "error in (no error)"=w323, "value"=w305, "key"="Receiver Email", "refnum"=w322) -> ("error out"=w321:errorcluster, "refnum out"=w320:T8)  [unwired: 4 in, 1 out]
        n243 = call-poly <vilib>:"Write Key.vi"("section"=w298, "error in (no error)"=w321, "value"=w304, "key"="subject", "refnum"=w320) -> ("error out"=w319:errorcluster, "refnum out"=w318:T8)  [unwired: 4 in, 1 out]
        n244 = call-poly <vilib>:"Write Key.vi"("section"=w298, "error in (no error)"=w319, "value"=w303, "key"="message", "refnum"=w318) -> ("error out"=w299:errorcluster, "refnum out"=w302:T8)  [unwired: 4 in, 1 out]
        n245 = call-poly <vilib>:"Write Key.vi"("section"=w298, "error in (no error)"=w299, "value"=w297, "key"="Attach data?", "refnum"=w302) -> ("error out"=w300:errorcluster, "refnum out"=w301:T8)  [unwired: 4 in, 1 out]
        n246 = call <vilib>:"Close Config Data.vi"("error in (no error)"=w300, "refnum"=w301) -> ()  [unwired: 8 in, 2 out]
      }
      event "Sample Number": Value Change {
        w336 = 50000 ("y")
        # "34465A maximun data number"
        n247 = event-data() -> ("NewVal"=w339:i32)  [unwired: 1 in, 5 out]
        n248 = local read "Current Mode"() -> (w340:u8[][])
        n249 = Array Size(array=w340) -> (size(s)=w341:i32[])
        n250 = Index Array(array=w341, index=0) -> (element=w335:i32)
        n251 = Multiply(x=w339, y=w335) -> (x*y=w338:i32)
        n252 = Greater?(x=w338, y=w336) -> (0:w337:bool)
        n253 = case shown="True" w337 {
          tunnel: w336 -> [_ w345]
          tunnel: w335 -> [_ w344]
          frame False {
          }
          frame True {
            n254 = Quotient & Remainder(x=w345, y=w344) -> (floor(x/y)=w343:i32)  [unwired: 1 out]
            n255 = local write "Sample Number"(w343) -> ()
            n256 = One Button Dialog(message="Data number can't be\nhigher than DMM available ") -> ()  [unwired: 1 in, 1 out]
          }
        }
      }
    }
  }
  n257 = while {
    shift-right: [w350] -> w15
    shift-left: errorcluster {"status"=FALSE, "code"=0, "source"=""} ("error out") -> [w356]
    shift-right: [w351] -> w6
    shift-left: refnum<visa-resource-name> refnum ("VISA Refnum out") -> [w355]
    tunnel: [TRUE] -> w14
    i -> [w347]
    stop <- w353 stop-if-true
    n258 = local read "State"() -> (w354:string)
    n259 = Wait (ms)(milliseconds to wait=u32 10) -> ()  [unwired: 1 out]
    n260 = case shown="\"Connect\"" w354 {
      tunnel: w356 -> [w362 w586 _ w881 w899 w923 w1085]
      tunnel: w355 -> [w363 w587 _ w882 w900 w924 w1086]
      tunnel: [w362 errorcluster {"status"=FALSE, "code"=0, "source"=""} ("error out") w689 w881 w897 w921 w1033] -> w350
      tunnel: [w363 refnum<visa-resource-name> refnum ("VISA Refnum out") w688 w882 w898 w922 w1034] -> w351
      tunnel: [w357 "Connect" ("State") w653 "Connect" ("State") "" ("State") "" ("State") "" ("State")] -> w349
      tunnel: w347 -> [_ _ w650 _ _ _ _]
      frame Default {
        n261 = Format Date/Time String(time format string (%c)="%S") -> (date/time string=w361:string)  [unwired: 2 in]
        n262 = Equal?(x=w361, y="00") -> (x = y?=w358:bool)
        n263 = case shown="False" w358 {
          tunnel: [w365 w380] -> w357
          frame False {
            n264 = local read "State temp"() -> (w364:string)
            n265 = Equal?(x="", y=w364) -> (x = y?=w366:bool)
            n266 = case shown="True" w366 {
              tunnel: [w369 w370] -> w365
              tunnel: w364 -> [w369 w370]
              frame False {
                n267 = local write "State temp"("" ("State temp")) -> ()
              }
              frame True {
              }
            }
          }
          frame True {
            n268 = Format Date/Time String(time format string (%c)="%Y_%m_%d_%H_%M") -> (date/time string=w372:string)  [unwired: 2 in]
            n269 = Match Pattern(string=w372, regular expression="Leave Timer") -> (match substring=w375:string, after substring=w376:string)  [unwired: 1 in, 2 out]
            n270 = Empty String/Path?(string/path=w375) -> (empty?=w377:bool)
            n271 = Empty String/Path?(string/path=w376) -> (empty?=w379:bool)
            n272 = Not(x=w377) -> (.not. x?=w378:bool)
            n273 = And(x=w378, y=w379) -> (x .and. y?=w371:bool)
            n274 = case shown="False" w371 {
              tunnel: [w384 "" ("State")] -> w380
              tunnel: w372 -> [w382 _]
              frame False {
                n275 = String Length(string=w382) -> (length=w381:i32)
                n276 = for {
                  tunnel: "Scan Start Timer" -> [w397] mode=indexing
                  tunnel: [w404] -> w386 mode=indexing
                  tunnel: w382 -> [w401]
                  tunnel: w381 -> [w399]
                  n277 = String Length(string=w397) -> (length=w400:i32)
                  n278 = Subtract(x=w399, y=w400) -> (x-y=w398:i32)
                  n279 = Match Pattern(string=w401, regular expression=w397, offset (0)=w398) -> (match substring=w407:string, after substring=w406:string)  [unwired: 2 out]
                  n280 = Empty String/Path?(string/path=w407) -> (empty?=w405:bool)
                  n281 = Empty String/Path?(string/path=w406) -> (empty?=w402:bool)
                  n282 = Not(x=w405) -> (.not. x?=w403:bool)
                  n283 = And(x=w403, y=w402) -> (x .and. y?=w404:bool)
                }
                n284 = Or Array Elements(Boolean array=w386) -> (logical OR=w385:bool)
                n285 = case shown="True" w385 {
                  tunnel: [w387 "Scan" ("State")] -> w384
                  frame False {
                    n286 = local read "State temp"() -> (w389:string)
                    n287 = Equal?(x="", y=w389) -> (x = y?=w390:bool)
                    n288 = case shown="False" w390 {
                      tunnel: [w392 w393] -> w387
                      tunnel: w389 -> [w392 w393]
                      frame False {
                        n289 = local write "State temp"("" ("State temp")) -> ()
                      }
                      frame True {
                      }
                    }
                  }
                  frame True {
                    n290 = local write "Scan start"(FALSE ("Scan start")) -> ()
                    n291 = property on="Scan Stop" class="Bool (strict)"("DisabledEnum"=T7."Enabled" ("Disabled")) -> ()  [unwired: 2 in, 2 out]
                  }
                }
              }
              frame True {
                n292 = local write "Leave"(TRUE ("Leave")) -> ()
              }
            }
          }
        }
      }
      frame "Initialize" {
        w442 = "Email Setting" ("section")
        w424 = "Setting" ("section")
        w585 = T6 0 items=["no dialog", "OK message", "continue or stop message", "OK message + warnings", "continue/stop + warnings"] ("type of dialog (OK msg:1)")
        n293 = VISA Close(VISA resource name=w587, error in (no error)=w586) -> (error out=w588:errorcluster)
        n294 = call <vilib>:"Simple Error Handler.vi"("type of dialog (OK msg:1)"=w585, "error in (no error)"=w588) -> ()  [unwired: 8 out]
        n295 = call <vilib>:"Application Directory.vi"() -> ("Application Directory"=w602:path)
        n296 = call <vilib>:"Application Directory.vi"() -> ("Application Directory"=w604:path)
        n297 = call <vilib>:"Application Directory.vi"() -> ("Application Directory"=w607:path)
        n298 = Build Path(base path=w602, name or relative path="Current Mode.csv") -> (appended path=w599:path)
        n299 = Build Path(base path=w604, name or relative path="setting.txt") -> (appended path=w600:path)
        n300 = Build Path(base path=w607, name or relative path="Current Set Mode.csv") -> (appended path=w605:path)
        n301 = call "Read Current Sense Resistivity.vi"("configuration file path"=w600) -> ("error out"=w613:errorcluster, "Array"=w617:dbl[], "file path"=w614:path)  [unwired: 8 in]
        "Current Sense \nResitance Array" <- w617
        n302 = property on="Upload\nCurrent\nSet \nMode" class="Bool (strict)"("Colors [4]"=cluster{u32, u32}[] [{16777216, 13816530}], "Value"=FALSE ("Upload\nCurrent\nMode")) -> ()  [unwired: 2 in, 2 out]
        n303 = call-poly <vilib>:"Read Delimited Spreadsheet.vi"("file path (dialog if empty)"=w605, "delimiter (\\t)"="," ("delimiter (\\t)")) -> ("all rows"=w610:string[][])  [unwired: 8 in, 5 out]
        n304 = call-poly <vilib>:"Read Delimited Spreadsheet.vi"("file path (dialog if empty)"=w599, "delimiter (\\t)"="," ("delimiter (\\t)")) -> ("all rows"=w609:i64[][])  [unwired: 8 in, 5 out]
        n305 = property on="Measured Current Sense Resistivity" class="LstBox (strict)"("Item Names"=string[] []) -> ()  [unwired: 2 in, 2 out]
        n306 = call "Updata Current Sense Resistance List.vi"("Array in"=w617) -> ("Array out"=w616:string[])  [unwired: 10 in]
        n307 = local write "Current Set Mode"(w610) -> ()
        n308 = local write "Current Mode"(w609) -> ()
        n309 = property on="Current Sense Resistivity List" class="LstBox (strict)"("Item Names"=w616) -> ()  [unwired: 2 in, 2 out]
        n310 = call "Read Current Set.vi"("configuration file path"=w614, "error in (no error)"=w613) -> ("Current Set"=w612:u8[][])  [unwired: 6 in, 2 out]
        n311 = local write "Current Set"(w612) -> ()
        n312 = property on="Resistance Test Stop" class="Bool (strict)"("DisabledEnum"=T7."Disabled and Grayed Out" ("Disabled")) -> ()  [unwired: 2 in, 2 out]
        n313 = property on="Leave" class="Bool (strict)"("DisabledEnum"=T7."Enabled" ("Disabled")) -> ()  [unwired: 2 in, 2 out]
        n314 = flat-sequence {
          tunnel: [w624] -> w507
          frame #0 {
            w623 = T7."Disabled and Grayed Out" ("Disabled")
            n315 = property on="Scan start" class="Bool (strict)"("DisabledEnum"=w623) -> ()  [unwired: 2 in, 2 out]
            n316 = property on="Calibrate start" class="Bool (strict)"("DisabledEnum"=w623) -> ()  [unwired: 2 in, 2 out]
            n317 = property on="Resistance Test start" class="Bool (strict)"("DisabledEnum"=w623) -> ()  [unwired: 2 in, 2 out]
            n318 = property on="Update Resistivity" class="Bool (strict)"("DisabledEnum"=w623) -> ()  [unwired: 2 in, 2 out]
          }
          frame #1 {
            n319 = call <vilib>:"Application Directory.vi"() -> ("Application Directory"=w624:path)
          }
        }
        n320 = Build Path(base path=w507, name or relative path="setting.txt") -> (appended path=w508:path)
        n321 = call <vilib>:"Open Config Data.vi"("configuration file path"=w508) -> ("error out"=w510:errorcluster, "refnum"=w511:T8)  [unwired: 8 in, 1 out]
        n322 = call-poly <vilib>:"Read Key.vi"("section"=w424, "error in (no error)"=w510, "key"="Neglect Timeout Data" ("Label.Text"), "refnum"=w511) -> ("error out"=w557:errorcluster, "value"=w530:bool, "refnum out"=w558:T8)  [unwired: 4 in, 1 out]
        n323 = local write "Neglect\nTimeout Data"(w530) -> ()
        n324 = call-poly <vilib>:"Read Key.vi"("section"=w424, "error in (no error)"=w557, "key"="Constant Scan Number" ("Label.Text"), "refnum"=w558) -> ("error out"=w515:errorcluster, "value"=w506:bool, "refnum out"=w516:T8)  [unwired: 4 in, 1 out]
        n325 = local write "Constant Scan Number"(w506) -> ()
        n326 = Not(x=w506) -> (.not. x?=w505:bool)
        n327 = property on="Current period" class="DigNum (strict)"("Visible"=w505) -> ()  [unwired: 2 in, 2 out]
        n328 = property on="Scan Number" class="DigNum (strict)"("Visible"=w506) -> ()  [unwired: 2 in, 2 out]
        n329 = call-poly <vilib>:"Read Key.vi"("section"=w424, "error in (no error)"=w515, "key"="Scan Number" ("Label.Text"), "refnum"=w516) -> ("error out"=w513:errorcluster, "value"=w512:u32, "refnum out"=w514:T8)  [unwired: 4 in, 1 out]
        n330 = local write "Scan Number"(w512) -> ()
        n331 = call-poly <vilib>:"Read Key.vi"("section"=w424, "error in (no error)"=w513, "key"="Enable Accurate Measure" ("Label.Text"), "refnum"=w514) -> ("error out"=w555:errorcluster, "value"=w504:bool, "refnum out"=w556:T8)  [unwired: 4 in, 1 out]
        n332 = local write "Enable Accurate \nMeasure"(w504) -> ()
        n333 = call-poly <vilib>:"Read Key.vi"("section"=w424, "error in (no error)"=w555, "key"="Enable DMM Relay" ("Label.Text"), "refnum"=w556) -> ("error out"=w553:errorcluster, "value"=w529:bool, "refnum out"=w554:T8)  [unwired: 4 in, 1 out]
        n334 = local write "Enable DMM\n Relay"(w529) -> ()
        n335 = Select(t=T7."Enabled" ("Disabled"), s=w504, f=T7."Disabled and Grayed Out" ("Disabled")) -> (s? t:f=w584:T7)
        n336 = call-poly <vilib>:"Read Key.vi"("section"=w424, "error in (no error)"=w553, "key"="Measure Current Only" ("Label.Text"), "refnum"=w554) -> ("error out"=w551:errorcluster, "value"=w528:bool, "refnum out"=w552:T8)  [unwired: 4 in, 1 out]
        n337 = local write "Measure Current \nOnly"(w528) -> ()
        n338 = property on="Measure Current \nOnly" class="Bool (strict)"("DisabledEnum"=w584) -> ()  [unwired: 2 in, 2 out]
        n339 = property on="Enable DMM\n Relay" class="Bool (strict)"("DisabledEnum"=w584) -> ()  [unwired: 2 in, 2 out]
        n340 = property on="Record Accurate \nData Only" class="Bool (strict)"("DisabledEnum"=w584) -> ()  [unwired: 2 in, 2 out]
        n341 = call-poly <vilib>:"Read Key.vi"("section"=w424, "error in (no error)"=w551, "key"="Record Accurate Data Only" ("Label.Text"), "refnum"=w552) -> ("error out"=w549:errorcluster, "value"=w527:bool, "refnum out"=w550:T8)  [unwired: 4 in, 1 out]
        n342 = local write "Record Accurate \nData Only"(w527) -> ()
        n343 = call-poly <vilib>:"Read Key.vi"("section"=w424, "error in (no error)"=w549, "key"="Remote PSU" ("Label.Text"), "refnum"=w550) -> ("error out"=w547:errorcluster, "value"=w503:bool, "refnum out"=w548:T8)  [unwired: 4 in, 1 out]
        n344 = local write "Remote\nPSU"(w503) -> ()
        n345 = call-poly <vilib>:"Read Key.vi"("section"=w424, "error in (no error)"=w547, "key"="Output Max Voltage" ("Label.Text"), "refnum"=w548) -> ("error out"=w545:errorcluster, "value"=w526:dbl, "refnum out"=w546:T8)  [unwired: 4 in, 1 out]
        n346 = local write "Output Max Voltage"(w526) -> ()
        n347 = Select(t=T7."Enabled" ("Disabled"), s=w503, f=T7."Disabled and Grayed Out" ("Disabled")) -> (s? t:f=w583:T7)
        n348 = call-poly <vilib>:"Read Key.vi"("section"=w424, "error in (no error)"=w545, "key"="Output Max Current" ("Label.Text"), "refnum"=w546) -> ("error out"=w439:errorcluster, "value"=w525:dbl, "refnum out"=w440:T8)  [unwired: 4 in, 1 out]
        n349 = local write "Output Max Current"(w525) -> ()
        n350 = property on="Output Max Voltage" class="DigNum (strict)"("DisabledEnum"=w583) -> ()  [unwired: 2 in, 2 out]
        n351 = property on="PSU(9184B)" class="VISAName"("DisabledEnum"=w583) -> ()  [unwired: 2 in, 2 out]
        n352 = property on="Output Max Current" class="DigNum (strict)"("DisabledEnum"=w583) -> ()  [unwired: 2 in, 2 out]
        n353 = call-poly <vilib>:"Read Key.vi"("section"=w424, "error in (no error)"=w439, "key"="safe Mode?" ("Label.Text"), "refnum"=w440) -> ("error out"=w437:errorcluster, "value"=w423:bool, "refnum out"=w438:T8)  [unwired: 4 in, 1 out]
        n354 = local write "safe Mode?"(w423) -> ()
        n355 = call-poly <vilib>:"Read Key.vi"("section"=w424, "error in (no error)"=w437, "key"="PSU Buffer Time" ("Label.Text"), "refnum"=w438) -> ("error out"=w435:errorcluster, "value"=w421:u32, "refnum out"=w436:T8)  [unwired: 4 in, 1 out]
        n356 = local write "PSU Buffer Time"(w421) -> ()
        n357 = call-poly <vilib>:"Read Key.vi"("section"=w424, "error in (no error)"=w435, "key"="Waiting Time" ("Label.Text"), "refnum"=w436) -> ("error out"=w433:errorcluster, "value"=w418:u32, "refnum out"=w434:T8)  [unwired: 4 in, 1 out]
        n358 = local write "Waiting\nTime"(w418) -> ()
        n359 = call-poly <vilib>:"Read Key.vi"("section"=w424, "error in (no error)"=w433, "key"="Switch On Time" ("Label.Text"), "refnum"=w434) -> ("error out"=w431:errorcluster, "value"=w416:u32, "refnum out"=w432:T8)  [unwired: 4 in, 1 out]
        n360 = local write "Switch On Time"(w416) -> ()
        n361 = call-poly <vilib>:"Read Key.vi"("section"=w424, "error in (no error)"=w431, "key"="Switch Off Time" ("Label.Text"), "refnum"=w432) -> ("error out"=w429:errorcluster, "value"=w415:u32, "refnum out"=w430:T8)  [unwired: 4 in, 1 out]
        n362 = local write "Switch Off Time"(w415) -> ()
        n363 = call-poly <vilib>:"Read Key.vi"("section"=w424, "error in (no error)"=w429, "key"="Sample Mode" ("Label.Text"), "refnum"=w430) -> ("error out"=w427:errorcluster, "value"=w413:u32, "refnum out"=w428:T8)  [unwired: 4 in, 1 out]
        n364 = local write "Sample Mode"(w413) -> ()
        n365 = call-poly <vilib>:"Read Key.vi"("section"=w424, "error in (no error)"=w427, "key"="Sample Number" ("Label.Text"), "refnum"=w428) -> ("error out"=w425:errorcluster, "value"=w411:i32, "refnum out"=w426:T8)  [unwired: 4 in, 1 out]
        n366 = local write "Sample Number"(w411) -> ()
        n367 = call-poly <vilib>:"Read Key.vi"("section"=w424, "error in (no error)"=w425, "key"="Array Mode" ("Label.Text"), "refnum"=w426) -> ("error out"=w543:errorcluster, "value"=w524:u32, "refnum out"=w544:T8)  [unwired: 4 in, 1 out]
        n368 = local write "Array Mode"(w524) -> ()
        n369 = call-poly <vilib>:"Read Key.vi"("section"=w424, "error in (no error)"=w543, "key"="Electrode number, N" ("Label.Text"), "refnum"=w544) -> ("error out"=w541:errorcluster, "value"=w523:u32, "refnum out"=w542:T8)  [unwired: 4 in, 1 out]
        n370 = local write "Electrode number, N"(w523) -> ()
        n371 = call-poly <vilib>:"Read Key.vi"("section"=w424, "error in (no error)"=w541, "key"="Current Channel" ("Label.Text"), "refnum"=w542) -> ("error out"=w539:errorcluster, "value"=w522:string, "refnum out"=w540:T8)  [unwired: 4 in, 1 out]
        n372 = local write "Current Channel"(w522) -> ()
        n373 = call-poly <vilib>:"Read Key.vi"("section"=w424, "error in (no error)"=w539, "key"="Insert Break" ("Label.Text"), "refnum"=w540) -> ("error out"=w537:errorcluster, "value"=w517:bool, "refnum out"=w538:T8)  [unwired: 4 in, 1 out]
        n374 = local write "Insert\nBreak"(w517) -> ()
        n375 = call-poly <vilib>:"Read Key.vi"("section"=w424, "error in (no error)"=w537, "key"="Break Period Multipier" ("Label.Text"), "refnum"=w538) -> ("error out"=w535:errorcluster, "value"=w521:dbl, "refnum out"=w536:T8)  [unwired: 4 in, 1 out]
        n376 = local write "Break Period Multipier"(w521) -> ()
        n377 = call-poly <vilib>:"Read Key.vi"("section"=w424, "error in (no error)"=w535, "key"="Only Use Last Value?" ("Label.Text"), "refnum"=w536) -> ("error out"=w533:errorcluster, "value"=w520:bool, "refnum out"=w534:T8)  [unwired: 4 in, 1 out]
        n378 = local write "Only Use Last Value?"(w520) -> ()
        n379 = call-poly <vilib>:"Read Key.vi"("section"=w424, "error in (no error)"=w533, "key"="Inverse Polarity" ("Label.Text"), "refnum"=w534) -> ("error out"=w531:errorcluster, "value"=w519:bool, "refnum out"=w532:T8)  [unwired: 4 in, 1 out]
        n380 = local write "Inverse\nPolarity"(w519) -> ()
        n381 = call-poly <vilib>:"Read Key.vi"("section"=w424, "error in (no error)"=w531, "key"="Wait Current Stable Period" ("Label.Text"), "refnum"=w532) -> ("error out"=w458:errorcluster, "value"=w518:u32, "refnum out"=w460:T8)  [unwired: 4 in, 1 out]
        n382 = local write "Wait Current Stable Period"(w518) -> ()
        n383 = call-poly <vilib>:"Read Key.vi"("section"=w424, "error in (no error)"=w458, "key"="Save Raw Data" ("Label.Text"), "refnum"=w460) -> ("error out"=w457:errorcluster, "value"=w455:bool, "refnum out"=w459:T8)  [unwired: 4 in, 1 out]
        n384 = local write "Save\nRaw Data"(w455) -> ()
        n385 = call-poly <vilib>:"Read Key.vi"("section"=w424, "error in (no error)"=w457, "key"="Scan Start Timer", "refnum"=w459) -> ("error out"=w499:errorcluster, "value"=w485:string, "refnum out"=w500:T8)  [unwired: 4 in, 1 out]
        n386 = while {
          shift-right: [w618] -> _
          shift-left: w485 -> [w622]
          tunnel: [w620] -> w484 mode=indexing
          stop <- w619 stop-if-true
          n387 = Match Pattern(string=w622, regular expression=",") -> (before substring=w620:string, after substring=w618:string)  [unwired: 1 in, 2 out]
          n388 = Empty String/Path?(string/path=w618) -> (empty?=w619:bool)
        }
        n389 = call-poly <vilib>:"Read Key.vi"("section"=w424, "error in (no error)"=w499, "key"="Send data Automatically", "refnum"=w500) -> ("error out"=w497:errorcluster, "value"=w482:bool, "refnum out"=w498:T8)  [unwired: 4 in, 1 out]
        n390 = local write "Send data\nAutomatically"(w482) -> ()
        n391 = call-poly <vilib>:"Read Key.vi"("section"=w424, "error in (no error)"=w497, "key"="Leave Timer", "refnum"=w498) -> ("error out"=w495:errorcluster, "value"=w480:string, "refnum out"=w496:T8)  [unwired: 4 in, 1 out]
        n392 = local write "Leave Timer"(w480) -> ()
        n393 = local write "Scan Start Timer"(w484) -> ()
        n394 = call-poly <vilib>:"Read Key.vi"("section"=w442, "error in (no error)"=w495, "key"="server address", "refnum"=w496) -> ("error out"=w493:errorcluster, "value"=w467:string, "refnum out"=w494:T8)  [unwired: 4 in, 1 out]
        n395 = call-poly <vilib>:"Read Key.vi"("section"=w442, "error in (no error)"=w493, "key"="from", "refnum"=w494) -> ("error out"=w491:errorcluster, "value"=w466:string, "refnum out"=w492:T8)  [unwired: 4 in, 1 out]
        n396 = call-poly <vilib>:"Read Key.vi"("section"=w442, "error in (no error)"=w491, "key"="username", "refnum"=w492) -> ("error out"=w489:errorcluster, "value"=w465:string, "refnum out"=w490:T8)  [unwired: 4 in, 1 out]
        n397 = call-poly <vilib>:"Read Key.vi"("section"=w442, "error in (no error)"=w489, "key"="APP password", "refnum"=w490) -> ("error out"=w487:errorcluster, "value"=w464:string, "refnum out"=w488:T8)  [unwired: 4 in, 1 out]
        n398 = call-poly <vilib>:"Read Key.vi"("section"=w442, "error in (no error)"=w487, "key"="Receiver Email", "refnum"=w488) -> ("error out"=w478:errorcluster, "value"=w463:string, "refnum out"=w479:T8)  [unwired: 4 in, 1 out]
        n399 = call-poly <vilib>:"Read Key.vi"("section"=w442, "error in (no error)"=w478, "key"="subject", "refnum"=w479) -> ("error out"=w476:errorcluster, "value"=w462:string, "refnum out"=w477:T8)  [unwired: 4 in, 1 out]
        n400 = call-poly <vilib>:"Read Key.vi"("section"=w442, "error in (no error)"=w476, "key"="message", "refnum"=w477) -> ("error out"=w446:errorcluster, "value"=w461:string, "refnum out"=w447:T8)  [unwired: 4 in, 1 out]
        n401 = call-poly <vilib>:"Read Key.vi"("section"=w442, "error in (no error)"=w446, "key"="Attach data?", "refnum"=w447) -> ("error out"=w444:errorcluster, "value"=w441:bool, "refnum out"=w445:T8)  [unwired: 4 in, 1 out]
        n402 = Bundle("value"=w467, "value"=w466, "value"=w465, "value"=w464, "value"=w463, "value"=w462, "value"=w461, "value"=w441) -> (w468:T10)  [unwired: 1 in]
        n403 = call <vilib>:"Close Config Data.vi"("error in (no error)"=w444, "refnum"=w445) -> ("file path"=w502:path)  [unwired: 8 in, 1 out]
        n404 = call "Read Setting_ver2.vi"("configuration file path"=w502) -> ("output cluster 2"=w598:T11)  [unwired: 6 in, 2 out]
        n405 = Unbundle(w598) -> ("DMM VISA"=w453:refnum<visa-resource-name>, "ESP32 VISA"=w451:refnum<visa-resource-name>, "Scan Period"=w597:u32, "Current period"=w596:u32, "Scan Measure\nTime(uS)"=w595:i32, "Measure\nMax Voltage"=w594:dbl, "Data Directory"=w593:path, "Voltage max"=w592:dbl, "Voltage min"=w591:dbl, "Current max"=w590:dbl, "Current min"=w589:dbl, "PSU(9184B)"=w454:refnum<visa-resource-name>)
        n406 = local write "Sample Measure\nTime(uS)"(w595) -> ()
        n407 = local write "PSU(9184B)"(w454) -> ()
        n408 = local write "Scan Period"(w597) -> ()
        n409 = local write "Current period"(w596) -> ()
        n410 = local write "Measure\nMax Voltage"(w594) -> ()
        n411 = local write "Data Directory"(w593) -> ()
        n412 = local write "Voltage max"(w592) -> ()
        n413 = local write "Voltage min"(w591) -> ()
        n414 = local write "Current max"(w590) -> ()
        n415 = local write "Current min"(w589) -> ()
        n416 = local write "DMM VISA"(w453) -> ()
        n417 = local write "ESP32 VISA"(w451) -> ()
        n418 = local write "Email Setting"(w468) -> ()
      }
      frame "Connect" {
        w637 = "^\\s*(Agilent|Keysight)\\s+Technologies\\s*\\,"  # Company Name Regular Expression
        w639 = "*IDN?"  # ID Query
        w667 = u32 100  # Bytes
        w628 = T6 0 items=["no dialog", "OK message", "continue or stop message", "OK message + warnings", "continue/stop + warnings"] ("type of dialog (OK msg:1)")
        # "clear input buffer"
        n419 = local read "ESP32 VISA"() -> (w687:refnum<visa-resource-name>)
        n420 = local read "DMM VISA"() -> (w627:refnum<visa-resource-name>)
        n421 = local read "Remote\nPSU"() -> (w679:bool)
        n422 = case shown="True" w679 {
          tunnel: [errorcluster {"status"=FALSE, "code"=0, "source"=""} ("error out") w837] -> w686
          tunnel: w628 -> [_ w835]
          tunnel: [refnum<visa-resource-name> refnum ("VISA resource name out") w825] -> w683
          tunnel: [FALSE w822] -> w680
          frame False {
          }
          frame True {
            w828 = u32 100  # Bytes
            n423 = local read "PSU(9184B)"() -> (w834:refnum<visa-resource-name>)
            n424 = call-poly "VISA Configure Serial Port"("VISA resource name"=w834, "timeout (10sec)"=u32 100, "baud rate (9600)"=u32 57600) -> ("VISA resource name out"=w830:refnum<visa-resource-name>, "error out"=w829:errorcluster)  [unwired: 11 in]
            n425 = Concatenate Strings("*IDN?" ("write buffer"), "\r\n") -> (w832:string)
            n426 = VISA Write(VISA resource name=w830, write buffer=w832, error in (no error)=w829) -> (VISA resource name out=w827:refnum<visa-resource-name>, error out=w826:errorcluster)  [unwired: 1 out]
            n427 = VISA Read(VISA resource name=w827, byte count=w828, error in (no error)=w826) -> (VISA resource name out=w825:refnum<visa-resource-name>, read buffer=w815:string, error out=w824:errorcluster)  [unwired: 1 out]
            n428 = Match Pattern(string=w815, regular expression="9185B") -> (offset past match=w817:i32)  [unwired: 1 in, 3 out]
            n429 = Match Pattern(string=w815, regular expression="9184B") -> (offset past match=w820:i32)  [unwired: 1 in, 3 out]
            n430 = Less?(x=w817, y=0) -> (x < y?=w813:bool)
            n431 = Less?(x=w820, y=0) -> (x < y?=w814:bool)
            n432 = call <vilib>:"Simple Error Handler.vi"("type of dialog (OK msg:1)"=w835, "error in (no error)"=w824) -> ("error?"=w823:bool, "error out"=w837:errorcluster)  [unwired: 3 in, 3 out]
            n433 = Compound Arithmetic op=AND(w814, w813) -> (w812:bool)
            n434 = Or(x=w823, y=w812) -> (x .or. y?=w822:bool)
          }
        }
        n435 = VISA Open(access mode=u32 0, VISA resource name=w627) -> (VISA resource name=w646:refnum<visa-resource-name>, error out=w645:errorcluster)  [unwired: 1 in, 2 out]
        n436 = call-poly "VISA Configure Serial Port"("VISA resource name"=w687, "timeout (10sec)"=u32 100, "Enable Termination\nChar (T)"=FALSE ("Enable Termination\nChar (T)"), "baud rate (9600)"=u32 115200) -> ("VISA resource name out"=w670:refnum<visa-resource-name>, "error out"=w668:errorcluster)  [unwired: 10 in]
        n437 = VISA Read(VISA resource name=w670, byte count=w667, error in (no error)=w668) -> (VISA resource name out=w669:refnum<visa-resource-name>, error out=w659:errorcluster)  [unwired: 2 out]
        n438 = VISA Clear(VISA resource name=w646, error in (no error)=w645) -> (VISA resource name out=w644:refnum<visa-resource-name>, error out=w643:errorcluster)
        n439 = property class="Instr"(reference=w644, error in=w643, "General Settings:Timeout Value"=u32 1000) -> (reference out=w633:refnum<visa-resource-name>, error out=w632:errorcluster)
        n440 = property class="Instr"(reference=w669, "TermChar En"=TRUE ("Message Based Settings:Termination Character Enable")) -> (reference out=w661:refnum<visa-resource-name>, error out=w658:errorcluster)  [unwired: 1 in]
        n441 = VISA Write(VISA resource name=w633, write buffer=w639, error in (no error)=w632) -> (VISA resource name out=w642:refnum<visa-resource-name>, error out=w641:errorcluster)  [unwired: 1 out]
        n442 = call <vilib>:"Simple Error Handler.vi"("type of dialog (OK msg:1)"=w628, "error in (no error)"=w659) -> ()  [unwired: 3 in, 5 out]
        n443 = VISA Read(VISA resource name=w642, byte count=u32 256, error in (no error)=w641) -> (VISA resource name out=w630:refnum<visa-resource-name>, read buffer=w636:string, error out=w631:errorcluster)  [unwired: 1 out]
        n444 = xnode "Match Regular Expression"("input string"=w636, "regular expression"=w637) -> ("after match"=w635:string)  [unwired: 4 in, 4 out]
        n445 = VISA Write(VISA resource name=w661, write buffer="*IDN?\n", error in (no error)=w658) -> (VISA resource name out=w677:refnum<visa-resource-name>, error out=w676:errorcluster)  [unwired: 1 out]
        n446 = call <instrlib>:"Close.vi"("error in (no error)"=w631, "VISA resource name"=w630) -> ("error out"=w629:errorcluster)  [unwired: 9 in]
        n447 = Match First String(2:string[] ["34465A", "34470A"] ("string array"), 3:w635) -> (0:w634:i32)  [unwired: 1 out]
        n448 = VISA Read(VISA resource name=w677, byte count=w667, error in (no error)=w676) -> (VISA resource name out=w675:refnum<visa-resource-name>, read buffer=w664:string, error out=w674:errorcluster)  [unwired: 1 out]
        n449 = Less Than 0?(x=w634) -> (x < 0?=w626:bool)
        n450 = Match Pattern(string=w664, regular expression="ESP32_") -> (after substring=w625:string, offset past match=w666:i32)  [unwired: 1 in, 2 out]
        n451 = Less?(x=w666, y=0) -> (x < y?=w662:bool)
        n452 = call <vilib>:"Simple Error Handler.vi"("type of dialog (OK msg:1)"=w628, "error in (no error)"=w629) -> ()  [unwired: 3 in, 5 out]
        n453 = call <vilib>:"Simple Error Handler.vi"("type of dialog (OK msg:1)"=w628, "error in (no error)"=w674) -> ("error?"=w682:bool, "error out"=w690:errorcluster)  [unwired: 3 in, 3 out]
        n454 = Or(x=w682, y=w662) -> (x .or. y?=w681:bool)
        n455 = case shown="False" w681 {
          tunnel: w675 -> [_ w869]
          tunnel: [refnum<visa-resource-name> refnum ("VISA resource name out") w867] -> w688
          tunnel: [errorcluster {"status"=FALSE, "code"=0, "source"=""} ("error out") w866] -> w689
          tunnel: w690 -> [_ w868]
          tunnel: ["Fail to connect ESP32,please select a right port.\n" ("message") "" ("message")] -> w656
          frame True {
          }
          frame False {
            n456 = local write "ESP32 VISA"(w869) -> ()
            n457 = local read "Sample Measure\nTime(uS)"() -> (w870:i32)
            n458 = local read "Enable Accurate \nMeasure"() -> (w874:bool)
            n459 = local read "Switch Off Time"() -> (w873:u8)
            n460 = local read "Switch On Time"() -> (w872:u8)
            n461 = local read "Measure Current \nOnly"() -> (w871:bool)
            n462 = call "ESP32_initialize_3.vi"("ESP32 IN"=w869, "Switch On Time"=w872, "Switch Off Time"=w873, "Enable Accurate \nMeasure"=w874, "error in (no error)"=w868, "Measure Current \nOnly"=w871, "Sample Measure\nTime(uS)"=w870) -> ("ESP32 out"=w867:refnum<visa-resource-name>, "error out"=w866:errorcluster)  [unwired: 7 in]
            "ESP32 connect?" <- TRUE
          }
        }
        n463 = case shown="True" w680 {
          tunnel: w683 -> [_ w841]
          tunnel: w686 -> [_ _]
          tunnel: ["Fail to connect PSU,please select a right port.\n" ("message") "" ("message")] -> w655
          frame True {
            n464 = local write "PSU(9184B)"(refnum<visa-resource-name> refnum ("VISA resource name out")) -> ()
          }
          frame False {
            n465 = local write "PSU(9184B)"(w841) -> ()
          }
        }
        n466 = Or(x=w626, y=w681) -> (x .or. y?=w685:bool)
        n467 = case shown="False" w626 {
          tunnel: w627 -> [_ w860]
          tunnel: ["Fail to connect DMM,please select a right port.\n" ("message") "" ("message")] -> w657
          frame True {
          }
          frame False {
            n468 = local write "DMM VISA"(w860) -> ()
          }
        }
        n469 = Or(x=w680, y=w685) -> (x .or. y?=w684:bool)
        n470 = Number To Decimal String(number=w650) -> (decimal integer string=w649:string)  [unwired: 1 in]
        n471 = Concatenate Strings("Connection #" ("string"), w649, "\n" ("string"), w657, w656, w655) -> (w654:string)
        n472 = case shown="False" w684 {
          tunnel: w654 -> [_ w853]
          tunnel: ["" ("State") w848] -> w653
          tunnel: w625 -> [w842 _]
          frame False {
            w847 = T7."Enabled" ("Disabled")
            n473 = property on="Calibrate start" class="Bool (strict)"("DisabledEnum"=w847) -> ()  [unwired: 2 in, 2 out]
            n474 = property on="Scan start" class="Bool (strict)"("DisabledEnum"=w847) -> ()  [unwired: 2 in, 2 out]
            n475 = property on="Resistance Test start" class="Bool (strict)"("DisabledEnum"=w847) -> ()  [unwired: 2 in, 2 out]
            n476 = Concatenate Strings("Successful connection." ("message"), "\nESP32 version:" ("string"), w842) -> (w845:string)
            n477 = local write "concatenated string 3"(w845) -> ()
          }
          frame True {
            w854 = T7."Disabled and Grayed Out" ("Disabled")
            n478 = local write "concatenated string 3"(w853) -> ()
            n479 = property on="Calibrate start" class="Bool (strict)"("DisabledEnum"=w854) -> ()  [unwired: 2 in, 2 out]
            n480 = property on="Resistance Test start" class="Bool (strict)"("DisabledEnum"=w854) -> ()  [unwired: 2 in, 2 out]
            n481 = property on="Scan start" class="Bool (strict)"("DisabledEnum"=w854) -> ()  [unwired: 2 in, 2 out]
            n482 = Wait (ms)(milliseconds to wait=u32 3000) -> ()  [unwired: 1 out]
            n483 = local read "State temp"() -> (w851:string)
            n484 = Equal?(x=w851, y="") -> (x = y?=w850:bool)
            n485 = case shown="False" w850 {
              tunnel: [w856 "Connect" ("State temp")] -> w848
              tunnel: w851 -> [w856 _]
              frame False {
                n486 = local write "State temp"("" ("State temp")) -> ()
              }
              frame True {
              }
            }
          }
        }
      }
      frame "R2 format convert" {
        n487 = case shown="\"Filled and splitted\"" "Conver Type:" {
          tunnel: "Modified Data path" -> [w886 w887 w896]
          tunnel: "Original Data path" -> [w885 w891 w895]
          tunnel: "R2 format_Scan number" -> [w884 w890 w894]
          tunnel: "Current set number in one current mode" -> [w883 w889 w893]
          frame "Regular", Default {
            n488 = call "Modify Data format to R2.vi"("Current set number in one current mode"=w883, "Scan number"=w884, "modified Data path"=w886, "original Data path"=w885) -> ()  [unwired: 8 in]
          }
          frame "Filled and splitted" {
            n489 = call "Modify Data format to R2_filled +split2.vi"("Current set number in one current mode"=w889, "Scan number"=w890, "modified Data path"=w887, "original Data path"=w891) -> ()  [unwired: 8 in]
            n490 = One Button Dialog(message="456") -> ()  [unwired: 1 in, 1 out]
          }
          frame "Filled" {
            n491 = call "Modify Data format to R2_filled.vi"("Current set number in one current mode"=w893, "Scan number"=w894, "modified Data path"=w896, "original Data path"=w895) -> ()  [unwired: 8 in]
            n492 = One Button Dialog(message="123") -> ()  [unwired: 1 in, 1 out]
          }
        }
      }
      frame "Calibrate" {
        n493 = flat-sequence {
          tunnel: w900 -> [w911]
          tunnel: w899 -> [w910]
          tunnel: [w909] -> w898
          tunnel: [w908] -> w897
          frame #0 {
            n494 = local read "Current Mode"() -> (w916:u8[][])
            n495 = local read "Switch On Time"() -> (w903:u8)
            n496 = local read "DMM VISA"() -> (w907:refnum<visa-resource-name>)
            n497 = Array Size(array=w916) -> (size(s)=w915:i32[])
            n498 = control-ref of="Measured Current Sense Resistivity"() -> (w905:refnum<vi>)
            n499 = Index Array(array=w915, index=0) -> (element=w917:i32)
            n500 = Multiply(x=w903, y=1e-06) -> (x*y=w902:dbl)
            n501 = control-ref of="Calibrate Stop"() -> (w906:refnum<vi>)
            n502 = control-ref of="Time out count:"() -> (w913:refnum<vi>)
            n503 = control-ref of="Measured Current Sense \nResitance Array"() -> (w914:refnum<vi>)
            n504 = call "Calibrate Current Sense Resistiviy.vi"("DMM ref in"=w907, "Measured Current Sense Resistivity REF"=w905, "Calibrate Stop REF"=w906, "Channel  Count"=w917, "Current Sense \nResitance Array\nREF"=w914, "ESP32 ref in"=w911, "ESP32 error in"=w910, "Manual Trigger Delay (1 s)"=w902, "Time out count REF"=w913) -> ("ESP32 ref out"=w909:refnum<visa-resource-name>, "ESP32 error out"=w908:errorcluster)  [unwired: 5 in]
          }
          frame #1 {
            n505 = local write "Calibrate Stop"(FALSE ("Calibrate Stop")) -> ()
            n506 = property on="Update Resistivity" class="Bool (strict)"("DisabledEnum"=T7."Enabled" ("Disabled")) -> ()  [unwired: 2 in, 2 out]
            n507 = property on="Calibrate Stop" class="Bool (strict)"("DisabledEnum"=T7."Disabled and Grayed Out" ("Disabled")) -> ()  [unwired: 2 in, 2 out]
          }
        }
      }
      frame "Resistance Test" {
        n508 = flat-sequence {
          tunnel: w924 -> [w944]
          tunnel: w923 -> [w943]
          tunnel: [w942] -> w922
          tunnel: [w941] -> w921
          frame #0 {
            n509 = local read "Current Mode"() -> (w947:u8[][])
            n510 = local read "Remote\nPSU"() -> (w927:bool)
            n511 = local read "PSU(9184B)"() -> (w928:refnum<visa-resource-name>)
            n512 = local read "Output Max Voltage"() -> (w929:dbl)
            n513 = local read "Output Max Current"() -> (w930:dbl)
            n514 = local read "PSU Buffer Time"() -> (w931:u32)
            n515 = local read "DMM VISA"() -> (w940:refnum<visa-resource-name>)
            n516 = local read "Current Sense \nResitance Array"() -> (w936:dbl[])
            n517 = local read "External\nPSU"() -> (w935:bool)
            n518 = local read "Switch On Time"() -> (w933:u8)
            n519 = control-ref of="Resistance Test"() -> (w938:refnum<vi>)
            n520 = Array Size(array=w947) -> (size(s)=w946:i32[])
            n521 = Index Array(array=w946, index=0) -> (element=w948:i32)
            n522 = Bundle("Remote\nPSU"=w927, "PSU(9184B)"=w928, "Output Max Voltage"=w929, "Output Max Current"=w930, "PSU Buffer Time"=w931) -> (w926:T12)  [unwired: 1 in]
            n523 = Multiply(x=w933, y=1e-06) -> (x*y=w932:dbl)
            n524 = control-ref of="Resistance Test Stop"() -> (w939:refnum<vi>)
            n525 = case shown="True" w935 {
              tunnel: w948 -> [w960 w968]
              tunnel: w944 -> [w959 w967]
              tunnel: w943 -> [w958 w966]
              tunnel: [w957 w965] -> w942
              tunnel: [w956 w964] -> w941
              tunnel: w940 -> [w955 w963]
              tunnel: w939 -> [w954 w962]
              tunnel: w938 -> [w953 w961]
              tunnel: "Wait Current Stable Period" -> [w952 _]
              tunnel: w936 -> [w951 _]
              tunnel: w932 -> [w950 _]
              tunnel: w926 -> [w949 _]
              frame True {
                n526 = call "Resistance Test_ver2_3.vi"("DMM ref in"=w955, "Resistance Test REF"=w953, "Resistance Test Stop REF"=w954, "PSU setting"=w949, "Channel  Count"=w960, "ESP32 ref in"=w959, "ESP32 error in"=w958, "Wait Current Stable Period"=w952, "Manual Trigger Delay (1 s)"=w950, "Current Sense \nResitance Array"=w951) -> ("ESP32 ref out"=w957:refnum<visa-resource-name>, "ESP32 error out"=w956:errorcluster)  [unwired: 4 in]
              }
              frame False {
                n527 = call "Resistance Test_byDMM_ver2.vi"("DMM ref in"=w963, "Resistance Test REF"=w961, "Resistance Test Stop REF"=w962, "Channel  Count"=w968, "ESP32 ref in"=w967, "ESP32 error in"=w966) -> ("ESP32 ref out"=w965:refnum<visa-resource-name>, "ESP32 error out"=w964:errorcluster)  [unwired: 8 in]
              }
            }
          }
          frame #1 {
            n528 = property on="Resistance Test Stop" class="Bool (strict)"("DisabledEnum"=T7."Disabled and Grayed Out" ("Disabled")) -> ()  [unwired: 2 in, 2 out]
            n529 = local write "Resistance Test Stop"(FALSE ("Calibrate Stop")) -> ()
          }
        }
      }
      frame "Scan" {
        w1037 = 0 ("f")
        w971 = "Setting" ("section")
        w1226 = 100 ("y")
        w1276 = 0 items=["Positive", "Negative"] ("Trigger Edge (1: Negative)")
        w1274 = 2 items=["Immediate", "Software (Bus)", "External"]  # Trigger Source
        w1275 = FALSE  # Auto Delay
        # "to milliseconds\nand *1.3 which is  empirical value"
        # "plot and save\nthe rest of the date"
        # "rough time for\nswitch REF"
        # "Reconnect DMM?"
        # "scan count"
        # "accurate data"
        # "It cost 50mS to turn on \"one\" current channel\n40mS to turn on \"one\" V channel"
        # ".set plot interpolation to 2 just like default,\nor it will causing more than 50mS when\nX scale change with 64 channels, rather than\n6mS, I think that is some kind of bug in\nlabview."
        # "Current mode"
        # "timeout count"
        # "N number"
        # "P number"
        # "accurate measure,Command'a' toggle"
        # "Current mode index"
        # "how many channel"
        # "how many state"
        # "Data matrix index"
        # "V for left Y axis\nI for right Y"
        # "Enable only plotting the number \nof data that fit plot width"
        # "Enanble dynamiclly scale?"
        # "this can be smaller\nto reduce the matrix size,\nas long as its value is bigger than 2"
        # "initilal time"
        n530 = local write "Time out count:"(0 ("Time out count")) -> ()
        n531 = call <vilib>:"Application Directory.vi"() -> ("Application Directory"=w1219:path)
        n532 = call <vilib>:"Application Directory.vi"() -> ("Application Directory"=w1216:path)
        n533 = Build Path(base path=w1219, name or relative path="Current Mode.csv") -> (appended path=w1217:path)
        n534 = call <vilib>:"Application Directory.vi"() -> ("Application Directory"=w1213:path)
        n535 = local read "Enable Accurate \nMeasure"() -> (w1082:bool)
        n536 = Build Path(base path=w1216, name or relative path="setting.txt") -> (appended path=w1214:path)
        n537 = Build Path(base path=w1213, name or relative path="Current Set Mode.csv") -> (appended path=w1211:path)
        n538 = local read "Data Directory"() -> (w1206:path)
        n539 = property on="Leave" class="Bool (strict)"("DisabledEnum"=T7."Disabled and Grayed Out" ("Disabled")) -> ()  [unwired: 2 in, 2 out]
        n540 = Array Size(array="Current Mode") -> (size(s)=w1281:i32[])
        n541 = local read "Current Set Mode"() -> (w1237:string[][])
        n542 = local read "Current Set"() -> (w1236:u8[][])
        n543 = local read "Insert\nBreak"() -> (w1184:bool)
        n544 = property on="XY Graph" class="XYGraph (strict)"() -> ("Width"=w1288:u32)  [unwired: 2 in, 2 out]
        n545 = Index Array(array=w1281, index=1) -> (element=w1251:i32)
        n546 = Index Array(array=w1281, index=0) -> (element=w1080:i32)
        n547 = Tick Count (ms)() -> (millisecond timer value=w1301:u32)
        n548 = stacked-sequence {
          tunnel: [_ "DMM VISA"] -> w1277
          tunnel: [w2684 _] -> w1091
          tunnel: [w2683 _] -> w1090
          tunnel: [w2681 _] -> w1088
          frame #0 {
            n549 = local read "Remote\nPSU"() -> (w2680:bool)
            n550 = case shown="True" w2680 {
              tunnel: [refnum<visa-resource-name> refnum ("VISA resource name out") w2689] -> w2684
              tunnel: [errorcluster {"status"=FALSE, "code"=0, "source"=""} ("error out") w2688] -> w2683
              tunnel: "safe Mode?" -> [_ w2687]
              frame False {
              }
              frame True {
                n551 = local read "Output Max Voltage"() -> (w2692:dbl)
                n552 = local read "Output Max Current"() -> (w2691:dbl)
                n553 = local read "PSU(9184B)"() -> (w2693:refnum<visa-resource-name>)
                n554 = local write "PSU Enable"(TRUE ("PSU Enable")) -> ()
                n555 = call "PSU_initialize_2.vi"("safe Mode?"=w2687, "Current"=w2691, "Voltage"=w2692, "VISA resource name"=w2693) -> ("error out"=w2688:errorcluster, "VISA resource name out"=w2689:refnum<visa-resource-name>)  [unwired: 6 in]
              }
            }
            n556 = And(x=w2680, y="safe Mode?") -> (x .and. y?=w2681:bool)
          }
          frame #1 {
          }
        }
        n557 = Compound Arithmetic op=ADD("Switch On Time", "Switch Off Time", "Sample Measure\nTime(uS)") -> (w1078:i32)
        n558 = Format Date/Time String(time format string (%c)="%Y_%m_%d_%H_%M") -> (date/time string=w1209:string)  [unwired: 2 in]
        n559 = local read "Sample Mode"() -> (w1018:u16)
        n560 = local read "Sample Number"() -> (w1015:i32)
        n561 = call "Write Current Set.vi"("configuration file path"=w1214, "Current Set"=w1236) -> ("file path"=w1197:path, "error out"=w1196:errorcluster)  [unwired: 7 in]
        n562 = call-poly <vilib>:"Write Delimited Spreadsheet.vi"("file path (dialog if empty)"=w1217, "2D data"="Current Mode", "delimiter (\\t)"="," ("delimiter (\\t)")) -> ()  [unwired: 11 in, 2 out]
        n563 = call-poly <vilib>:"Write Delimited Spreadsheet.vi"("file path (dialog if empty)"=w1211, "2D data"=w1237, "delimiter (\\t)"="," ("delimiter (\\t)")) -> ()  [unwired: 11 in, 2 out]
        n564 = Compound Arithmetic op=MULTIPLY(w1080, w1078) -> (w1230:i32)
        n565 = Add(x=w1230, y=500) -> (x+y=w1012:i32)
        "Period for one sample" <- w1012
        n566 = Concatenate Strings(w1209, ".csv" ("pattern (all files)")) -> (w1210:string)
        n567 = To Long Integer(number=w1288) -> (32bit integer=w1300:i32)
        n568 = local write "channel count"(w1080) -> ()
        n569 = local read "Sample Measure\nTime(uS)"() -> (w1200:i32)
        n570 = Multiply(x="Scan Number", y="Break Period Multipier") -> (x*y=w1181:dbl)
        n571 = Multiply(x="Current period", y="Break Period Multipier") -> (x*y=w1180:dbl)
        n572 = Multiply(x=w1012, y="Sample Number") -> (x*y=w1002:i32)
        n573 = Multiply(x=2, y=w1080) -> (x*y=w1252:i32)
        n574 = local read "Measure\nMax Voltage"() -> (w1199:dbl)
        n575 = Multiply(x=2, y=w1300) -> (x*y=w1298:i32)
        n576 = Equal To 0?(x=w1018) -> (x = 0?=w1016:bool)
        n577 = Round To Nearest(number=w1181) -> (nearest integer value=w1183:dbl)
        n578 = Round To Nearest(number=w1180) -> (nearest integer value=w1182:dbl)
        n579 = local read "Current period"() -> (w1201:u32)
        n580 = local read "Data Directory"() -> (w1198:path)
        n581 = To Unsigned Long Integer(number=w1183) -> (unsigned 32bit integer=w1175:u32)
        n582 = To Unsigned Long Integer(number=w1182) -> (unsigned 32bit integer=w1174:u32)
        n583 = local read "Voltage max"() -> (w1191:dbl)
        n584 = local read "PSU(9184B)"() -> (w1185:refnum<visa-resource-name>)
        n585 = local read "Voltage min"() -> (w1190:dbl)
        n586 = local read "Current max"() -> (w1189:dbl)
        n587 = stacked-sequence {
          tunnel: w1252 -> [w2695 _]
          tunnel: w1080 -> [_ w2709]
          frame #0 {
            n588 = for {
              N: w2695 -> [_]
              i -> [w2704]
              n589 = To Unsigned Long Integer(number=w2704) -> (unsigned 32bit integer=w2706:u32)
              n590 = Quotient & Remainder(x=w2706, y=u32 2) -> (x-y*floor(x/y)=w2698:u32, floor(x/y)=w2702:u32)
              n591 = To Long Integer(number=w2702) -> (32bit integer=w2701:i32)
              n592 = Index Array(array=u32[] [0, 3381759, 51218, 16711766, 10354830, 937121, 16770306, 24377, 65280, 9764922, 16749438, 10757120, 5444, 9556171, 6426112, 7039106, 255, 32181, 6980204, 44670, 12749983, 12491120, 36764, 6270286, 16711680, 16711926, 16712349, 6831419, 16741539, 9865960, 10026834, 10966848, 131070, 16772840, 16681216, 12437247, 119039, 12290048, 7685297, 10878930, 16754430, 7818496, 8013698, 2503680, 18260, 4390956, 11862271, 16757095, 16767846, 9501586, 8269266, 12440467, 15036414, 14614388, 65400, 39935, 25601, 30463, 8759552, 47383, 7897649, 65478, 16739905, 15228606] ("initial color"), index=w2701) -> (element=w2703:u32)
              n593 = To Unsigned Byte Integer(number=w2698) -> (unsigned 8bit integer=w2697:u8)
              n594 = Add(x=w2697, y=u8 1 ("Plot.Line Width")) -> (x+y=w2700:u8)
              n595 = property on="XY Graph" class="XYGraph (strict)"("Active Plot"=w2706, "Plot.YScaleIdx"=w2698, "Plot.Plot Color"=w2703, "Plot.Line Width"=w2700, "Plot.Plot Interpolation"=u8 2) -> ()  [unwired: 2 in, 2 out]
            }
          }
          frame #1 {
            n596 = control-ref of="XY Graph"() -> (w2708:refnum<vi>)
            n597 = control-ref of="plot setting"() -> (w2710:refnum<vi>)
            n598 = call "Initialize Monitor Setting.vi"("Channel number"=w2709, "XY Graph REF"=w2708, "plot setting"=w2710) -> ()  [unwired: 9 in]
          }
        }
        n599 = local read "Current min"() -> (w1188:dbl)
        n600 = local read "Scan Period"() -> (w1202:u32)
        n601 = Quotient & Remainder(x=w1002, y=770) -> (floor(x/y)=w1224:i32)  [unwired: 1 out]
        n602 = local read "DMM VISA"() -> (w1204:refnum<visa-resource-name>)
        n603 = local read "ESP32 VISA"() -> (w1203:refnum<visa-resource-name>)
        n604 = Build Path(base path=w1206, name or relative path=w1210) -> (appended path=w1205:path)
        n605 = Multiply(x=w1300, y=3) -> (x*y=w1019:i32)
        n606 = Build Path(base path=w1206, name or relative path="data_temp.csv" ("string")) -> (appended path=w1220:path)
        n607 = call <instrlib>:"Initialize.vi"("VISA resource name"=w1277) -> ("error out"=w1271:errorcluster, "VISA resource name out"=w1272:refnum<visa-resource-name>)  [unwired: 4 in, 5 out]
        n608 = Multiply(x="Switch On Time", y=1e-06) -> (x*y=w1074:dbl)
        n609 = local read "Sample Mode"() -> (w1071:u16)
        n610 = Add(x=w1224, y=25) -> (x+y=w1003:i32)
        n611 = Select(t=w1019, s=w1016, f=w1015) -> (s? t:f=w1017:i32)
        n612 = Multiply(x="Scan Period", y=w1288) -> (x*y=w1294:u32)
        n613 = To Double Precision Float(number=w1294) -> (double precision float=w1293:dbl)
        n614 = Greater?(x=w1003, y=w1226) -> (0:w1227:bool)
        n615 = VISA Write(VISA resource name=w1272, write buffer="DISP OFF", error in (no error)=w1271) -> (VISA resource name out=w1270:refnum<visa-resource-name>, error out=w1269:errorcluster)  [unwired: 1 out]
        n616 = Multiply(x=w1251, y=2) -> (x*y=w1248:i32)
        n617 = To Double Precision Float(number="Sample Measure\nTime(uS)") -> (double precision float=w1234:dbl)
        n618 = local read "Current Sense \nResitance Array"() -> (w1235:dbl[])
        n619 = Divide(x=w1293, y=1000.0) -> (x/y=w1285:dbl)
        n620 = Bundle("DMM VISA"=w1204, "ESP32 VISA"=w1203, "Scan Period"=w1202, "Current period"=w1201, "Sample Measure\nTime(uS)"=w1200, "Measure\nMax Voltage"=w1199, "Data Directory"=w1198, "Voltage max"=w1191, "Voltage min"=w1190, "Current max"=w1189, "Current min"=w1188, "PSU(9184B)"=w1185) -> (w1195:T13)  [unwired: 1 in]
        n621 = stacked-sequence {
          tunnel: "Current max" -> [_ _ _ w2716]
          tunnel: "Voltage max" -> [_ w2713 _ _]
          tunnel: "Voltage min" -> [_ w2712 _ _]
          tunnel: "Current min" -> [_ _ _ w2715]
          frame #0 {
            n622 = property on="XY Graph" class="XYGraph (strict)"("ActYScl"=0 ("Active Y Scale")) -> ()  [unwired: 2 in, 2 out]
          }
          frame #1 {
            n623 = property on="XY Graph" class="XYGraph (strict)"("YScale.Maximum"=w2713, "YScale.Minimum"=w2712) -> ()  [unwired: 2 in, 2 out]
          }
          frame #2 {
            n624 = property on="XY Graph" class="XYGraph (strict)"("ActYScl"=1 ("Active Y Scale")) -> ()  [unwired: 2 in, 2 out]
          }
          frame #3 {
            n625 = property on="XY Graph" class="XYGraph (strict)"("YScale.Maximum"=w2716, "YScale.Minimum"=w2715) -> ()  [unwired: 2 in, 2 out]
          }
        }
        n626 = Select(t=w1003, s=w1227, f=w1226) -> (s? t:f=w1225:i32)
        n627 = Select(t=w1248, s="Record Accurate \nData Only", f=0) -> (s? t:f=w1246:i32)
        n628 = call "Write Setting_ver2.vi"("configuration file path"=w1197, "output cluster"=w1195, "error in (no error)"=w1196) -> ("file path"=w1103:path, "error out"=w1104:errorcluster)  [unwired: 6 in]
        n629 = Decrement(x=w1175) -> (x-1=w1176:u32)
        n630 = call <instrlib>:"Configure Trigger.vi"("Manual Trigger Delay (1 s)"=w1074, "error in (no error)"=w1269, "Auto Delay (F:Disable)"=w1275, "Trigger Source (0: Immediate)"=w1274, "VISA resource name"=w1270) -> ("error out"=w1279:errorcluster, "VISA resource name out"=w1278:refnum<visa-resource-name>)  [unwired: 1 in, 4 out]
        n631 = property on="XY Graph" class="XYGraph (strict)"("XScale.Maximum"=w1285, "XScale.Minimum"=0.0 ("X Scale.Range:Minimum")) -> ()  [unwired: 2 in, 2 out]
        n632 = Decrement(x="Scan Number") -> (x-1=w1186:u32)
        n633 = call "ESP32_initialize_3.vi"("ESP32 IN"=w1086, "Switch On Time"="Switch On Time", "Switch Off Time"="Switch Off Time", "Enable Accurate \nMeasure"=w1082, "Sample Mode"=w1071, "error in (no error)"=w1085, "Measure Current \nOnly"="Measure Current \nOnly", "Sample Measure\nTime(uS)"="Sample Measure\nTime(uS)", "Sample number"="Sample Number") -> ("ESP32 out"=w1084:refnum<visa-resource-name>, "error out"=w1083:errorcluster)  [unwired: 5 in]
        n634 = Select(t=w1176, s="Constant Scan Number", f=w1174) -> (s? t:f=w1172:u32)
        n635 = call <instrlib>:"Configure Trigger Slope.vi"("error in (no error)"=w1279, "Trigger Edge (1: Negative)"=w1276, "VISA resource name"=w1278) -> ("error out"=w1267:errorcluster, "VISA resource name out"=w1268:refnum<visa-resource-name>)  [unwired: 7 in]
        n636 = call-poly <vilib>:"Write Delimited Spreadsheet.vi"("file path (dialog if empty)"=w1220, "append to file? (new file:F)"=FALSE) -> ("new file path (Not A Path if cancelled)"=w1223:path)  [unwired: 12 in, 1 out]
        n637 = Divide(x=w1234, y=1000000.0) -> (x/y=w1233:dbl)
        n638 = And(x="Enable\nPlot", y="Auto Plot \nCurrent") -> (x .and. y?=w1256:bool)
        n639 = Initialize Array(0.0 ("element"), w1252, w1017) -> (w1303:dbl[][])
        n640 = Initialize Array(0.0 ("element"), w1017) -> (w1302:dbl[])
        n641 = Initialize Array(u32 0 ("Current index"), w1017) -> (w1254:u32[])
        n642 = Initialize Array(0.0 ("element"), w1252, w1246) -> (w1243:dbl[][])
        n643 = Initialize Array(999999.0 ("element"), w1246) -> (w1242:dbl[])
        n644 = Initialize Array(u32 999999 ("Current index"), w1246) -> (w1241:u32[])
        n645 = Decrement(x=w1019) -> (x-1=w1297:i32)
        n646 = Greater?(x=w1071, y=u16 0) -> (0:w1073:bool)
        n647 = local read "Neglect\nTimeout Data"() -> (w1157:bool)
        n648 = case shown="False" w1073 {
          tunnel: w1303 -> [w1407 w1984]
          tunnel: w1302 -> [_ w1983]
          tunnel: w1301 -> [w1402 w1917]
          tunnel: w1300 -> [_ w1982]
          tunnel: w1298 -> [_ w1981]
          tunnel: w1297 -> [_ w1980]
          tunnel: "Scan Period" -> [_ w1979]
          tunnel: FALSE -> [_ w1978]
          tunnel: FALSE -> [_ w1977]
          tunnel: w1285 -> [_ w1976]
          tunnel: -1 -> [_ w1975]
          tunnel: w1268 -> [w1435 w1974]
          tunnel: w1267 -> [w1434 w1973]
          tunnel: TRUE -> [_ w1972]
          tunnel: u32 0 ("Current index") -> [_ w1971]
          tunnel: 0 -> [_ w1970]
          tunnel: 0 -> [_ w1969]
          tunnel: 0 ("Time out count") -> [_ w1968]
          tunnel: u8[] [] ("subarray") -> [_ w1967]
          tunnel: "Enable DMM\n Relay" -> [_ w1966]
          tunnel: "Enable\nPlot" -> [_ w1965]
          tunnel: w1256 -> [_ w1964]
          tunnel: w1254 -> [_ w1963]
          tunnel: w1252 -> [w1405 w1962]
          tunnel: w1251 -> [w1433 w1961]
          tunnel: "Record Accurate \nData Only" -> [_ w1960]
          tunnel: w1243 -> [_ w1959]
          tunnel: w1242 -> [_ w1958]
          tunnel: w1241 -> [_ w1957]
          tunnel: "Current Mode" -> [w1422 w1956]
          tunnel: w1235 -> [w1403 w1955]
          tunnel: w1233 -> [w1427 w1954]
          tunnel: "Measure\nMax Voltage" -> [w1428 w1953]
          tunnel: w1225 -> [w1393 w1952]
          tunnel: w1223 -> [w1411 w1951]
          tunnel: w1205 -> [w1412 w1950]
          tunnel: "Neglect\nTimeout Data" -> [_ w1949]
          tunnel: 0 -> [_ w1948]
          tunnel: w1186 -> [_ w1947]
          tunnel: w1184 -> [_ w1946]
          tunnel: "Current period" -> [_ w1945]
          tunnel: "Constant Scan Number" -> [_ w1944]
          tunnel: w1172 -> [_ w1943]
          tunnel: "Enable Accurate \nMeasure" -> [_ w1942]
          tunnel: FALSE ("Reconnect DMM?") -> [_ w1941]
          tunnel: w1091 -> [w1426 w1940]
          tunnel: w1090 -> [w1425 w1939]
          tunnel: "PSU Buffer Time" -> [w1421 w1938]
          tunnel: w1088 -> [w1420 w1937]
          tunnel: w1084 -> [w1424 w1936]
          tunnel: w1083 -> [w1423 w1935]
          tunnel: "Measure Current \nOnly" -> [_ w1934]
          tunnel: w1080 -> [w1404 w1933]
          tunnel: "Sample Number" -> [w1431 w1932]
          tunnel: [w1419 w1931] -> w1007
          tunnel: [w1418 w1930] -> w1006
          tunnel: [w1417 w1929] -> w1005
          tunnel: [w1416 w1928] -> w1035
          tunnel: [w1410 w1927] -> w1010
          tunnel: [w1409 w1926] -> w1032
          tunnel: [dbl[][] [] w1925] -> w1031
          tunnel: [dbl[] [] w1924] -> w1030
          tunnel: [u32[] [] w1923] -> w1029
          tunnel: [w1401 w1922] -> w1028
          tunnel: [w1399 w1921] -> w1027
          tunnel: [w1398 w1920] -> w1026
          tunnel: [w1400 w1919] -> w1025
          tunnel: [T7."Disabled and Grayed Out" ("Disabled") w1918] -> w1020
          tunnel: w1015 -> [w1406 _]
          tunnel: [w1397 w1915] -> w1011
          tunnel: [T7."Enabled" ("Disabled") T7."Enabled" ("Disabled")] -> w1008
          tunnel: [FALSE ("Scan Stop") FALSE ("Scan Stop")] -> w1004
          frame True {
            # "Initialize DMM?"
            n649 = local read "Sample Mode"() -> (w1391:u16)
            n650 = local read "Waiting\nTime"() -> (w1390:u32)
            n651 = case shown="1, Default" w1391 {
              tunnel: w1431 -> [w1438 w1452]
              tunnel: w1404 -> [w1441 w1445]
              tunnel: [w1440 w1445] -> w1430
              tunnel: [1 ("Sample Number") w1452] -> w1429
              tunnel: w1393 -> [w1437 _]
              tunnel: [w1437 w1442] -> w1392
              frame 1, Default {
                n652 = Multiply(x=w1438, y=w1441) -> (x*y=w1440:i32)
              }
              frame 2 {
                # "buffer"
                n653 = local read "Sample Measure\nTime(uS)"() -> (w1450:i32)
                n654 = local read "Sample Number"() -> (w1451:i32)
                n655 = local read "Switch Off Time"() -> (w1449:u8)
                n656 = local read "Switch On Time"() -> (w1448:u8)
                n657 = Multiply(x=w1451, y=w1450) -> (x*y=w1447:i32)
                n658 = Compound Arithmetic op=ADD(w1447, w1449, w1448) -> (w1446:i32)
                n659 = Multiply(x=w1446, y=w1445) -> (x*y=w1444:i32)
                n660 = Add(x=w1444, y=10) -> (x+y=w1442:i32)
              }
            }
            n661 = local read "Period for one sample"() -> (w1396:i32)
            n662 = while {
              tunnel: w1433 -> [w1472]
              tunnel: w1391 -> [w1456]
              shift-right: [w1482] -> _
              shift-left: 0 -> [w1471]
              tunnel: w1430 -> [w1496]
              tunnel: w1429 -> [w1497]
              tunnel: w1428 -> [w1514]
              tunnel: w1427 -> [w1453]
              shift-right: [w1490] -> w1419
              shift-left: w1435 -> [w1499]
              shift-right: [w1489] -> w1418
              shift-left: w1434 -> [w1498]
              shift-right: [w1493] -> _
              shift-left: w1426 -> [w1510]
              shift-right: [w1492] -> _
              shift-left: w1425 -> [w1509]
              shift-right: [w1488] -> w1417
              shift-left: w1424 -> [w1508]
              shift-right: [w1487] -> w1416
              shift-left: w1423 -> [w1507]
              tunnel: w1422 -> [w1511]
              tunnel: w1404 -> [w1506]
              tunnel: w1421 -> [w1505]
              tunnel: w1420 -> [w1504]
              tunnel: w1390 -> [w1502]
              tunnel: w1392 -> [w1491]
              tunnel: w1412 -> [w1485]
              tunnel: w1411 -> [w1484]
              tunnel: [w1485] -> w1410
              tunnel: [w1483] -> w1409
              shift-right: [w1470] -> w1401
              shift-left: w1407 -> [w1481]
              tunnel: w1406 -> [w1464]
              tunnel: w1405 -> [w1479]
              tunnel: w1404 -> [w1478]
              tunnel: w1403 -> [w1474]
              tunnel: w1402 -> [w1473]
              tunnel: [w1468] -> w1400
              tunnel: [w1466] -> w1399
              tunnel: [w1467] -> w1398
              tunnel: [w1464] -> w1397
              tunnel: w1396 -> [w1459]
              shift-right: [w1454] -> _
              shift-left: TRUE -> [w1455]
              stop <- w1458 stop-if-true
              # "how many V channel"
              n663 = case shown="True" w1455 {
                tunnel: w1514 -> [_ w1524]
                tunnel: w1453 -> [_ w1523]
                tunnel: [w1516 w1522] -> w1513
                tunnel: [w1515 w1521] -> w1512
                tunnel: w1499 -> [w1516 w1520]
                tunnel: w1498 -> [w1515 w1519]
                tunnel: w1497 -> [_ w1518]
                tunnel: w1496 -> [_ w1517]
                frame False {
                }
                frame True {
                  n664 = call "Osc_DMM_Initilize.vi"("Scan Measure\nTime"=w1523, "Measure Maximun Voltage"=w1524, "error in (no error)"=w1519, "Trigger Count (1)"=w1517, "Sample Count (1)"=w1518, "VISA Refnum in"=w1520) -> ("error out"=w1521:errorcluster, "VISA Refnum out"=w1522:refnum<visa-resource-name>)  [unwired: 4 in]
                }
              }
              n665 = call <instrlib>:"Initiate.vi"("error in (no error)"=w1512, "VISA resource name"=w1513) -> ("error out"=w1462:errorcluster, "VISA resource name out"=w1463:refnum<visa-resource-name>)  [unwired: 8 in]
              n666 = Index Array(array=w1511, index (col)=w1471) -> (element=w1475:u8[])  [unwired: 1 in]
              n667 = case shown="True" w1504 {
                tunnel: w1510 -> [w1843 w1907]
                tunnel: w1509 -> [w1842 w1906]
                tunnel: w1508 -> [w1841 w1912]
                tunnel: w1507 -> [w1840 w1911]
                tunnel: w1475 -> [w1839 w1910]
                tunnel: w1471 -> [w1838 w1909]
                tunnel: w1506 -> [w1837 w1908]
                tunnel: w1505 -> [w1836 _]
                tunnel: [w1835 w1907] -> w1493
                tunnel: [w1834 w1906] -> w1492
                tunnel: [w1832 w1905] -> w1501
                tunnel: [w1830 w1904] -> w1500
                tunnel: [w1829 w1903] -> w1503
                tunnel: w1463 -> [w1828 w1902]
                tunnel: w1462 -> [w1827 w1901]
                tunnel: [w1820 w1902] -> w1461
                tunnel: [w1819 w1901] -> w1460
                frame True {
                  n668 = flat-sequence {
                    tunnel: w1843 -> [w1869]
                    tunnel: w1842 -> [w1868]
                    tunnel: [w1867] -> w1858
                    tunnel: w1841 -> [w1867]
                    tunnel: [w1866] -> w1857
                    tunnel: w1840 -> [w1866]
                    tunnel: w1839 -> [w1865]
                    tunnel: [w1865] -> w1856
                    tunnel: w1838 -> [w1864]
                    tunnel: [w1864] -> w1855
                    tunnel: [w1863] -> w1854
                    tunnel: [w1862] -> w1853
                    tunnel: w1836 -> [w1861]
                    tunnel: [w1861] -> w1852
                    tunnel: w1828 -> [w1860]
                    tunnel: w1827 -> [w1859]
                    tunnel: [w1860] -> w1824
                    tunnel: [w1859] -> w1821
                    tunnel: w1858 -> [w1879]
                    tunnel: w1857 -> [w1878]
                    tunnel: [w1879] -> w1851
                    tunnel: [w1878] -> w1850
                    tunnel: w1856 -> [w1877]
                    tunnel: [w1877] -> w1849
                    tunnel: w1855 -> [w1876]
                    tunnel: [w1876] -> w1848
                    tunnel: [w1875] -> w1847
                    tunnel: w1854 -> [w1875]
                    tunnel: [w1874] -> w1846
                    tunnel: w1853 -> [w1874]
                    tunnel: w1852 -> [w1873]
                    tunnel: [w1872] -> w1825
                    tunnel: w1824 -> [w1872]
                    tunnel: [w1871] -> w1822
                    tunnel: w1821 -> [w1871]
                    tunnel: w1851 -> [w1890]
                    tunnel: w1850 -> [w1889]
                    tunnel: w1849 -> [w1888]
                    tunnel: w1848 -> [w1887]
                    tunnel: w1837 -> [w1886]
                    tunnel: [w1885] -> w1845
                    tunnel: w1847 -> [w1885]
                    tunnel: [w1884] -> w1844
                    tunnel: w1846 -> [w1884]
                    tunnel: [w1883] -> w1833
                    tunnel: [w1882] -> w1831
                    tunnel: [w1881] -> w1826
                    tunnel: w1825 -> [w1881]
                    tunnel: [w1880] -> w1823
                    tunnel: w1822 -> [w1880]
                    tunnel: w1845 -> [w1899]
                    tunnel: w1844 -> [w1898]
                    tunnel: [w1897] -> w1835
                    tunnel: [w1896] -> w1834
                    tunnel: [w1895] -> w1832
                    tunnel: w1833 -> [w1895]
                    tunnel: [w1894] -> w1830
                    tunnel: w1831 -> [w1894]
                    tunnel: [w1893] -> w1829
                    tunnel: [w1892] -> w1820
                    tunnel: w1826 -> [w1892]
                    tunnel: [w1891] -> w1819
                    tunnel: w1823 -> [w1891]
                    frame #0 {
                      n669 = VISA Write(VISA resource name=w1869, write buffer="OUT 1\nOUT OFF\n", error in (no error)=w1868) -> (VISA resource name out=w1863:refnum<visa-resource-name>, error out=w1862:errorcluster)  [unwired: 1 out]
                    }
                    frame #1 {
                      n670 = Wait (ms)(milliseconds to wait=w1873) -> ()  [unwired: 1 out]
                    }
                    frame #2 {
                      n671 = call "Arduino_a.vi"("Channel Number"=w1886, "error in (no error)"=w1889, "Current  Setting"=w1888, "Current Mode Count"=w1887, "VISA Refnum in"=w1890) -> ("error out"=w1882:errorcluster, "VISA Refnum out"=w1883:refnum<visa-resource-name>)  [unwired: 5 in]
                    }
                    frame #3 {
                      n672 = Tick Count (ms)() -> (millisecond timer value=w1893:u32)
                      n673 = VISA Write(VISA resource name=w1899, write buffer="OUT 1\nOUT ON\n", error in (no error)=w1898) -> (VISA resource name out=w1897:refnum<visa-resource-name>, error out=w1896:errorcluster)  [unwired: 1 out]
                    }
                  }
                }
                frame False {
                  n674 = call "Arduino_a.vi"("Channel Number"=w1908, "error in (no error)"=w1911, "Current  Setting"=w1910, "Current Mode Count"=w1909, "VISA Refnum in"=w1912) -> ("error out"=w1904:errorcluster, "VISA Refnum out"=w1905:refnum<visa-resource-name>)  [unwired: 5 in]
                  n675 = Tick Count (ms)() -> (millisecond timer value=w1903:u32)
                }
              }
              n676 = for {
                N: w1478 -> [w1525]
                tunnel: w1475 -> [w1528] mode=indexing
                shift-right: [w1526] -> w1476
                shift-left: 0 -> [w1527]
                tunnel: [w1525] -> w1465
                n677 = case shown="0" w1528 {
                  tunnel: w1527 -> [w1529 w1532 w1533]
                  tunnel: [w1529 w1531 w1533] -> w1526
                  frame Default {
                    n678 = One Button Dialog(message="Error\nCurrent\nMode" ("error source (\" \")")) -> ()  [unwired: 1 in, 1 out]
                  }
                  frame 0 {
                    n679 = Increment(x=w1532) -> (x+1=w1531:i32)
                  }
                  frame 1, 2 {
                  }
                }
              }
              n680 = while {
                tunnel: w1503 -> [w1817]
                tunnel: w1502 -> [w1815]
                tunnel: [w1813] -> w1495
                tunnel: w1501 -> [w1813]
                tunnel: [w1812] -> w1494
                tunnel: w1500 -> [w1812]
                stop <- w1814 stop-if-true
                n681 = Tick Count (ms)() -> (millisecond timer value=w1818:u32)
                n682 = Subtract(x=w1818, y=w1817) -> (x-y=w1816:u32)
                n683 = Greater Or Equal?(x=w1816, y=w1815) -> (x >= y?=w1814:bool)
              }
              n684 = case shown="1, 2" w1456 {
                selector: w1456 -> [w1774 _]
                tunnel: w1461 -> [w1777 w1801]
                tunnel: w1460 -> [w1776 w1800]
                tunnel: w1497 -> [_ w1799]
                tunnel: w1496 -> [_ w1798]
                tunnel: w1495 -> [w1771 w1797]
                tunnel: w1494 -> [w1770 w1796]
                tunnel: w1491 -> [_ w1778]
                tunnel: [w1777 w1787] -> w1490
                tunnel: [w1776 w1786] -> w1489
                tunnel: [w1771 w1784] -> w1488
                tunnel: [FALSE ("error?") w1782] -> w1486
                tunnel: [w1770 w1783] -> w1487
                tunnel: [dbl[] [] ("Measurements") w1781] -> w1480
                tunnel: [0 ("Time out count") w1780] -> w1469
                tunnel: [FALSE w1779] -> w1454
                frame 0, Default {
                  n685 = Number To Decimal String(number=w1774) -> (decimal integer string=w1772:string)  [unwired: 1 in]
                  n686 = Concatenate Strings(w1772, " is not a available Sample Mode" ("message")) -> (w1773:string)
                  n687 = One Button Dialog(message=w1773) -> ()  [unwired: 1 in, 1 out]
                }
                frame 1, 2 {
                  # "remember to add time out"
                  n688 = Multiply(x=w1799, y=w1798) -> (x*y=w1791:i32)
                  n689 = VISA Write(VISA resource name=w1797, write buffer="b", error in (no error)=w1796) -> (VISA resource name out=w1792:refnum<visa-resource-name>, error out=w1783:errorcluster)  [unwired: 1 out]
                  n690 = call <instrlib>:"Fetch Multiple Points.vi"("error in (no error)"=w1800, "Timeout (10000 ms)"=w1778, "VISA resource name"=w1801) -> ("error out"=w1793:errorcluster, "Measurements"=w1781:dbl[], "VISA resource name out"=w1794:refnum<visa-resource-name>)  [unwired: 6 in]
                  n691 = call "Clear Scan Time Out_5.vi"("Timeout"=w1778, "Channel number\nx Sample number"=w1791, "ESP32 ref"=w1792, "error in (no error)"=w1793, "VISA Refnum in"=w1794) -> ("error out"=w1785:errorcluster, "error?"=w1782:bool, "Time out count"=w1780:i32, "VISA Refnum out"=w1788:refnum<visa-resource-name>, "ESP32 ref out"=w1784:refnum<visa-resource-name>)  [unwired: 2 in]
                  n692 = Greater Or Equal?(x=w1780, y=10000) -> (x >= y?=w1790:bool)
                  n693 = case shown="True" w1790 {
                    selector: w1790 -> [w1802 _]
                    tunnel: w1788 -> [w1804 w1811]
                    tunnel: [w1804 w1810] -> w1787
                    tunnel: [w1803 w1809] -> w1786
                    tunnel: w1785 -> [w1803 _]
                    tunnel: [w1802 TRUE] -> w1779
                    frame False {
                    }
                    frame True {
                      n694 = local read "Switch On Time"() -> (w1807:u8)
                      n695 = Multiply(x=w1807, y=1e-06) -> (x*y=w1805:dbl)
                      n696 = call "DMM Scan Reset_4.vi"("Manual Trigger Delay (1 s)"=w1805, "VISA in resource name"=w1811) -> ("error out"=w1809:errorcluster, "VISA resource name out"=w1810:refnum<visa-resource-name>)  [unwired: 8 in]
                    }
                  }
                }
              }
              n697 = case shown="False" w1486 {
                tunnel: w1471 -> [w1542 w1763]
                tunnel: [w1547 w1763] -> w1482
                tunnel: w1484 -> [w1541 w1765]
                tunnel: [w1540 w1765] -> w1483
                tunnel: w1481 -> [w1558 w1756]
                tunnel: w1464 -> [w1559 _]
                tunnel: w1480 -> [w1557 _]
                tunnel: w1479 -> [w1556 _]
                tunnel: w1465 -> [w1555 _]
                tunnel: w1476 -> [w1554 _]
                tunnel: w1475 -> [w1553 _]
                tunnel: w1474 -> [w1552 _]
                tunnel: w1473 -> [w1550 _]
                tunnel: [w1539 w1756] -> w1470
                tunnel: [w1543 dbl[] []] -> w1466
                tunnel: w1472 -> [w1546 _]
                tunnel: [w1545 w1759] -> w1468
                tunnel: [w1538 u32[] []] -> w1467
                tunnel: w1469 -> [_ w1760]
                tunnel: w1459 -> [w1536 _]
                tunnel: w1456 -> [w1535 _]
                tunnel: w1453 -> [w1534 _]
                frame False {
                  n698 = Tick Count (ms)() -> (millisecond timer value=w1551:u32)
                  n699 = Subtract(x=w1551, y=w1550) -> (x-y=w1549:u32)
                  n700 = case shown="2" w1535 {
                    tunnel: w1559 -> [_ w1579 w1650]
                    tunnel: w1558 -> [_ w1578 w1656]
                    tunnel: w1557 -> [_ w1577 w1651]
                    tunnel: w1556 -> [_ w1576 _]
                    tunnel: w1555 -> [_ w1575 _]
                    tunnel: w1554 -> [_ w1574 w1652]
                    tunnel: w1553 -> [_ w1573 w1654]
                    tunnel: w1552 -> [_ w1572 w1653]
                    tunnel: w1549 -> [_ w1571 w1664]
                    tunnel: [0 w1570 w1663] -> w1548
                    tunnel: [dbl[][] [] w1569 w1655] -> w1544
                    tunnel: [dbl[] [] w1568 w1662] -> w1543
                    tunnel: w1542 -> [_ w1567 w1661]
                    tunnel: [u32[] [] w1566 w1660] -> w1538
                    tunnel: w1536 -> [_ w1565 w1659]
                    tunnel: w1534 -> [_ _ w1649]
                    frame 0, Default {
                      n701 = One Button Dialog(message="Error in sample mode 1 or 2") -> ()  [unwired: 1 in, 1 out]
                    }
                    frame 1 {
                      n702 = for {
                        N: w1579 -> [w1580]
                        shift-right: [w1592] -> w1569
                        shift-left: w1578 -> [w1606]
                        tunnel: w1577 -> [w1599]
                        tunnel: w1576 -> [w1601]
                        tunnel: w1575 -> [w1598]
                        tunnel: w1574 -> [w1600]
                        tunnel: w1573 -> [w1595]
                        tunnel: w1572 -> [w1594]
                        tunnel: w1571 -> [w1590]
                        tunnel: [w1584] -> w1568 mode=indexing
                        tunnel: [w1580] -> w1570
                        tunnel: w1567 -> [w1583]
                        tunnel: [w1582] -> w1566 mode=indexing
                        tunnel: w1565 -> [w1581]
                        i -> [w1591]
                        n703 = Multiply(x=w1590, y=u32 1000) -> (x*y=w1587:u32)
                        n704 = Multiply(x=w1598, y=w1591) -> (x*y=w1597:i32)
                        n705 = Array Subset(array=w1599, index=w1597, length=w1598) -> (w1596:dbl[])
                        n706 = Multiply(x=w1591, y=w1581) -> (x*y=w1588:i32)
                        n707 = Initialize Array(0.0 ("Measurement"), w1601) -> (w1602:dbl[])
                        n708 = Add(x=w1587, y=w1588) -> (x+y=w1586:u32)
                        n709 = for {
                          shift-right: [w1614] -> w1593
                          shift-left: w1602 -> [w1615]
                          tunnel: w1595 -> [w1618] mode=indexing
                          tunnel: w1600 -> [w1611]
                          shift-right: [w1616] -> _
                          shift-left: 0 ("index") -> [w1617]
                          shift-right: [w1612] -> _
                          shift-left: 0 ("index") -> [w1613]
                          tunnel: w1594 -> [w1610]
                          tunnel: w1596 -> [w1607]
                          i -> [w1609]
                          n710 = Index Array(array=w1610, index=w1609) -> (element=w1608:dbl)
                          n711 = case shown="1, 2" w1618 {
                            tunnel: w1617 -> [w1622 w1632 w1642]
                            tunnel: [w1622 w1631 w1642] -> w1616
                            tunnel: w1609 -> [_ w1629 w1647]
                            tunnel: w1615 -> [w1621 w1630 w1648]
                            tunnel: [w1621 w1627 w1644] -> w1614
                            tunnel: w1613 -> [w1620 w1626 w1639]
                            tunnel: [w1620 w1626 w1638] -> w1612
                            tunnel: w1611 -> [_ _ w1641]
                            tunnel: w1608 -> [_ _ w1636]
                            tunnel: w1607 -> [_ w1624 w1634]
                            frame Default {
                              n712 = One Button Dialog(message="Error in Scan") -> ()  [unwired: 1 in, 1 out]
                            }
                            frame 0 {
                              n713 = Multiply(x=w1629, y=2 ("x")) -> (x*y=w1625:i32)
                              n714 = Index Array(array=w1624, index=w1632) -> (element=w1623:dbl)
                              n715 = Increment(x=w1632) -> (x+1=w1631:i32)
                              n716 = Replace Array Subset(array=w1630, new element=w1623, index=w1625) -> (w1627:dbl[])
                            }
                            frame 1, 2 {
                              n717 = Add(x=w1639, y=w1641) -> (x+y=w1640:i32)
                              n718 = Index Array(array=w1634, index=w1640) -> (element=w1633:dbl)
                              n719 = Multiply(x=w1647, y=2 ("x")) -> (x*y=w1645:i32)
                              n720 = Negate(x=w1633) -> (-x=w1635:dbl)
                              n721 = Increment(x=w1645) -> (x+1=w1643:i32)
                              n722 = Divide(x=w1635, y=w1636) -> (x/y=w1637:dbl)
                              n723 = Increment(x=w1639) -> (x+1=w1638:i32)
                              n724 = Replace Array Subset(array=w1648, new element=w1637, index=w1643) -> (w1644:dbl[])
                            }
                          }
                        }
                        n725 = Divide(x=w1586, y=1000000.0) -> (x/y=w1584:dbl)
                        n726 = To Unsigned Long Integer(number=w1583) -> (unsigned 32bit integer=w1582:u32)
                        n727 = Replace Array Subset(array=w1606, new element=w1593, index (col)=w1591) -> (w1592:dbl[][])  [unwired: 1 in]
                      }
                    }
                    frame 2 {
                      n728 = for {
                        N: w1650 -> [w1717]
                        tunnel: w1664 -> [w1723]
                        tunnel: [w1715] -> w1662 mode=indexing
                        tunnel: [w1717] -> w1663
                        tunnel: w1661 -> [w1720]
                        tunnel: [w1719] -> w1660 mode=indexing
                        tunnel: w1659 -> [_]
                        tunnel: w1649 -> [w1712]
                        i -> [w1718]
                        n729 = Multiply(x=w1723, y=u32 1000) -> (x*y=w1716:u32)
                        n730 = Multiply(x=w1718, y=w1712) -> (x*y=w1713:dbl)
                        n731 = Divide(x=w1716, y=1000000.0) -> (x/y=w1714:dbl)
                        n732 = Add(x=w1714, y=w1713) -> (x+y=w1715:dbl)
                        n733 = To Unsigned Long Integer(number=w1720) -> (unsigned 32bit integer=w1719:u32)
                      }
                      n734 = for {
                        shift-right: [w1673] -> w1655
                        shift-left: w1656 -> [w1674]
                        tunnel: w1654 -> [w1677] mode=indexing
                        tunnel: [w1666] -> _ mode=indexing
                        shift-right: [w1675] -> _
                        shift-left: 0 ("index") -> [w1676]
                        shift-right: [w1671] -> _
                        shift-left: 0 ("index") -> [w1672]
                        tunnel: w1653 -> [w1670]
                        tunnel: w1651 -> [w1667]
                        tunnel: w1652 -> [w1666]
                        tunnel: w1650 -> [w1665]
                        i -> [w1669]
                        n735 = Index Array(array=w1670, index=w1669) -> (element=w1668:dbl)
                        n736 = case shown="0" w1677 {
                          tunnel: w1676 -> [w1681 w1693 w1705]
                          tunnel: [w1681 w1692 w1705] -> w1675
                          tunnel: w1669 -> [_ w1690 w1710]
                          tunnel: w1674 -> [w1680 w1691 w1711]
                          tunnel: [w1680 w1688 w1707] -> w1673
                          tunnel: w1672 -> [w1679 w1687 w1702]
                          tunnel: [w1679 w1687 w1701] -> w1671
                          tunnel: w1666 -> [_ _ w1704]
                          tunnel: w1668 -> [_ _ w1700]
                          tunnel: w1667 -> [_ w1685 w1698]
                          tunnel: w1665 -> [_ w1682 w1695]
                          frame Default {
                            n737 = One Button Dialog(message="Error in Scan") -> ()  [unwired: 1 in, 1 out]
                          }
                          frame 0 {
                            n738 = Multiply(x=w1693, y=w1682) -> (x*y=w1683:i32)
                            n739 = Multiply(x=w1690, y=2 ("x")) -> (x*y=w1686:i32)
                            n740 = Array Subset(array=w1685, index=w1683, length=w1682) -> (w1684:dbl[])
                            n741 = Increment(x=w1693) -> (x+1=w1692:i32)
                            n742 = Replace Array Subset(array=w1691, new element=w1684, index (row)=w1686) -> (w1688:dbl[][])  [unwired: 1 in]
                          }
                          frame 1, 2 {
                            n743 = Add(x=w1702, y=w1704) -> (x+y=w1703:i32)
                            n744 = Multiply(x=w1695, y=w1703) -> (x*y=w1696:i32)
                            n745 = Array Subset(array=w1698, index=w1696, length=w1695) -> (w1697:dbl[])
                            n746 = Multiply(x=w1710, y=2 ("x")) -> (x*y=w1708:i32)
                            n747 = Negate(x=w1697) -> (-x=w1699:dbl[])
                            n748 = Increment(x=w1708) -> (x+1=w1706:i32)
                            n749 = Divide(x=w1699, y=w1700) -> (x/y=w1694:dbl[])
                            n750 = Increment(x=w1702) -> (x+1=w1701:i32)
                            n751 = Replace Array Subset(array=w1711, new element=w1694, index (row)=w1706) -> (w1707:dbl[][])  [unwired: 1 in]
                          }
                        }
                      }
                    }
                  }
                  n752 = Increment(x=w1542) -> (x+1=w1547:i32)
                  n753 = Greater Or Equal?(x=w1547, y=w1546) -> (x >= y?=w1545:bool)
                  n754 = Decrement(x=w1548) -> (x-1=w1537:i32)
                  n755 = case shown="False" w1545 {
                    tunnel: w1544 -> [w1730 w1743]
                    tunnel: w1543 -> [w1728 _]
                    tunnel: w1538 -> [w1727 _]
                    tunnel: w1541 -> [w1726 w1744]
                    tunnel: [w1725 w1744] -> w1540
                    tunnel: [w1724 w1743] -> w1539
                    frame False {
                      n756 = in-place {
                        in-place-border: w1728 -> [w1737]
                        in-place-border: w1727 -> [w1736]
                        in-place-border: w1726 -> [w1735]
                        in-place-border: [w1734] -> w1725
                        n757 = in-place-split #1(w1730, 0) -> (w1733:dbl[][])  [unwired: 1 out]
                        n758 = To Double Precision Float(number=w1736) -> (double precision float=w1741:dbl[])
                        n759 = Build Array (concatenate)(w1737, w1741, w1733) -> (w1742:dbl[][])
                        n760 = call-poly <vilib>:"Write Delimited Spreadsheet.vi"("file path (dialog if empty)"=w1735, "format (%.3f)"="%.9f", "2D data"=w1742, "append to file? (new file:F)"=TRUE, "transpose? (no:F)"=TRUE, "delimiter (\\t)"="," ("delimiter (\\t)")) -> ("new file path (Not A Path if cancelled)"=w1734:path)  [unwired: 8 in, 1 out]
                        n761 = in-place-split #1(dbl[][] [] ("element"), w1733) -> (w1724:dbl[][])  [unwired: 1 out]
                      }
                    }
                    frame True {
                    }
                  }
                  n762 = stacked-sequence {
                    tunnel: w1544 -> [_ w1752]
                    tunnel: w1543 -> [w1749 w1751]
                    tunnel: w1537 -> [w1747 _]
                    frame #0 {
                      n763 = Index Array(array=w1749, index=0) -> (element=w1745:dbl)
                      n764 = Index Array(array=w1749, index=w1747) -> (element=w1746:dbl)
                      n765 = property on="XY Graph" class="XYGraph (strict)"("XScale.Maximum"=w1746, "XScale.Minimum"=w1745) -> ()  [unwired: 2 in, 2 out]
                    }
                    frame #1 {
                      n766 = for {
                        tunnel: w1752 -> [w1755] mode=indexing
                        tunnel: w1751 -> [w1754]
                        tunnel: [w1753] -> w1750 mode=indexing
                        n767 = Bundle(w1754, w1755) -> (w1753:cluster{dbl[], dbl[]})  [unwired: 1 in]
                      }
                      n768 = local write "XY Graph"(w1750) -> ()
                    }
                  }
                }
                frame True {
                  n769 = local read "Time out count:"() -> (w1761:i32)
                  n770 = Add(x=w1761, y=w1760) -> (x+y=w1758:i32)
                  n771 = local write "Time out count:"(w1758) -> ()
                  n772 = Greater?(x=w1758, y=100000 ("x")) -> (0:w1759:bool)
                }
              }
              n773 = local read "Scan Stop"() -> (w1457:bool)
              n774 = Or(x=w1457, y=w1468) -> (x .or. y?=w1458:bool)
            }
          }
          frame False {
            n775 = while {
              shift-right: [w2059] -> w1922
              shift-left: w1984 -> [w2057]
              shift-right: [w2060] -> w1921
              shift-left: w1983 -> [w2056]
              shift-right: [w2058] -> w1916
              shift-left: w1975 -> [w2051]
              tunnel: [w2100] -> _
              tunnel: w1962 -> [w2100]
              tunnel: w1982 -> [w2064]
              tunnel: w1981 -> [w2055]
              tunnel: w1980 -> [w2063]
              tunnel: w1979 -> [w2070]
              tunnel: w1976 -> [w2099]
              shift-right: [w2098] -> _
              shift-left: w1978 -> [w2097]
              tunnel: w1965 -> [w2096]
              tunnel: w1951 -> [w2027]
              tunnel: [w2026] -> w1926
              tunnel: [w2064] -> _
              shift-right: [w2094] -> _
              shift-left: w1977 -> [w2095]
              tunnel: w1956 -> [w2090]
              tunnel: w1945 -> [w2093]
              shift-right: [w2006] -> _
              shift-left: w1971 -> [w2048]
              tunnel: w1917 -> [w2065]
              shift-right: [w2007] -> _
              shift-left: w1972 -> [w2072]
              shift-right: [w2079] -> w1929
              shift-left: w1936 -> [w2092]
              shift-right: [w2080] -> w1928
              shift-left: w1935 -> [w2091]
              tunnel: w1933 -> [w2030]
              tunnel: w1961 -> [w2073]
              shift-right: [w2001] -> w1931
              shift-left: w1974 -> [w2089]
              shift-right: [w1999] -> w1930
              shift-left: w1973 -> [w2088]
              shift-right: [w2078] -> _
              shift-left: w1970 -> [w2087]
              shift-right: [w2077] -> _
              shift-left: w1969 -> [w2086]
              shift-right: [w2074] -> _
              shift-left: w1968 -> [w2085]
              shift-right: [w2075] -> _
              shift-left: w1967 -> [w2076]
              shift-right: [w2068] -> _
              shift-left: w1917 -> [w2071]
              tunnel: w1964 -> [w2067]
              tunnel: w1934 -> [w2054]
              tunnel: w1960 -> [w2044]
              tunnel: [w2044] -> _
              tunnel: [w2054] -> _
              shift-right: [w2053] -> w1920
              shift-left: w1963 -> [w2052]
              shift-right: [w2040] -> w1925
              shift-left: w1959 -> [w2043]
              shift-right: [w2039] -> w1924
              shift-left: w1958 -> [w2042]
              shift-right: [w2038] -> w1923
              shift-left: w1957 -> [w2041]
              tunnel: w1955 -> [w2033]
              tunnel: w1954 -> [w2032]
              tunnel: w1953 -> [w2031]
              tunnel: w1952 -> [w1987]
              tunnel: [T7."Disabled and Grayed Out" ("Disabled")] -> w1918
              tunnel: w1950 -> [w2025]
              tunnel: [w2025] -> w1927
              tunnel: w1949 -> [w2013]
              shift-right: [w2004] -> _
              shift-left: w1948 -> [w2017]
              tunnel: w1944 -> [w2019]
              tunnel: w1947 -> [w2018]
              tunnel: w1946 -> [w2014]
              tunnel: w1943 -> [w2015]
              shift-right: [w1996] -> _
              shift-left: w1941 -> [w1997]
              tunnel: w1942 -> [w1994]
              tunnel: w1966 -> [w1998]
              tunnel: [w1992] -> w1919
              tunnel: w1940 -> [w1989]
              tunnel: w1939 -> [w1988]
              tunnel: w1938 -> [w1990]
              tunnel: w1937 -> [w1991]
              tunnel: w1932 -> [w1986]
              i -> [w2066]
              stop <- w1993 stop-if-true
              # "last Scan time"
              # "if data number in one current mode is longer than\none plot width, might trigger this proceduce, or will\ntrigger next procedure when matrix index is between\n2~3 plot width"
              # "When there are 64 channels,\nthis will take 60mS"
              # "when DMM aperature is 100uS,\nit take 37mS for 64 channels,\n10mS for 4 Channels"
              # "I didn't use in line struture here,\nthat's beacause I want to run measure data\nwhile plotting, the smallest period can be smaller,\nrather than plot \"after\" measure data.\nHowever, it might require more memory, since\nit need to copy a big data array to the plotting\nprocedure."
              # "TRY THIS\nminumum value might be\nbetter with\n \"maximun - initial maximum\"\nor it will keep changing range\nwhen enable accurate measurement"
              # "when there are 64 channels of data\nits minimun period is 25mS without other procedure,\nsetting propety of plot  casuing too much time,\nFurthermore, It need more than 20mS when data matrix \nis rearrangeing."
              # "updata plot when\ngetting each three new data\nthen scan speed can increase\nto \"almost\" 10mS, 15mS at\nlease is a safer period\nUpdate: It take at least 16mS parallelly,\nso don't run the following code in 16mS, or it will get delay"
              # "silver version of XY graph\nis faster than normal one"
              # "make sure there are only\nnumber of data that fit the\nwidth of the plot to be plotted"
              # "if disable plot\nminimun speed \ncan be 2mS"
              # "it cost about 50mS to change DMM setting\nwithout reseting DMM relay,\nor it will take 240 with reseting DMM relay"
              # "about 13mS to send current mode for 64 channel\n7mS for8channel, because about 90uS to send one\nbit when baud rate is 115200, it also need about 10uS\nto send one  bit from labview to USB chip on ESP32"
              n776 = Increment(x=w2051) -> (x+1=w2050:i32)
              n777 = Replace Array Subset(array=w2052, new element=w2048, index=w2050) -> (w2049:u32[])
              n778 = flat-sequence {
                tunnel: w2066 -> [w2412]
                tunnel: w2067 -> [w2413]
                tunnel: [w2414] -> w1995
                tunnel: w1994 -> [w2415]
                tunnel: [w2416] -> w2069
                tunnel: w2071 -> [w2417]
                tunnel: w2065 -> [w2418]
                tunnel: w2072 -> [w2419]
                tunnel: w2073 -> [w2420]
                tunnel: w2048 -> [w2406]
                tunnel: [w2421] -> w2024
                tunnel: [w2422] -> w2023
                tunnel: [w2423] -> w2022
                tunnel: [w2425] -> w2075
                tunnel: w2076 -> [w2426]
                tunnel: w2030 -> [w2427]
                tunnel: [w2428] -> w2077
                tunnel: [w2429] -> w2078
                tunnel: [w2430] -> w2081
                tunnel: [w2431] -> w2082
                tunnel: [w2432] -> w2083
                tunnel: [w2433] -> w2084
                tunnel: w2086 -> [w2434]
                tunnel: w2087 -> [w2435]
                tunnel: w2088 -> [w2436]
                tunnel: w2089 -> [w2437]
                tunnel: w2090 -> [w2438]
                tunnel: w2091 -> [w2439]
                tunnel: w2092 -> [w2440]
                tunnel: w2093 -> [w2401]
                tunnel: w2048 -> [w2411]
                tunnel: w1998 -> [w2397]
                tunnel: w2032 -> [w2409]
                tunnel: w2031 -> [w2408]
                tunnel: w2019 -> [w2400]
                tunnel: w2017 -> [w2405]
                tunnel: w2018 -> [w2404]
                tunnel: [w2407] -> w2016
                tunnel: w2015 -> [w2399]
                tunnel: w2014 -> [w2403]
                tunnel: w1997 -> [w2396]
                tunnel: w1991 -> [w2395]
                tunnel: w1990 -> [w2394]
                tunnel: w1989 -> [w2393]
                tunnel: w1988 -> [w2392]
                tunnel: w1986 -> [w2391]
                frame #0 {
                  # "compare scan count with\nscan number for \"break mode\""
                  # "accurate meausre"
                  # "finish scan?"
                  n779 = Equal To 0?(x=w2411) -> (x = 0?=w2410:bool)
                  n780 = Tick Count (ms)() -> (millisecond timer value=w2424:u32)
                  n781 = Subtract(x=w2424, y=w2418) -> (x-y=w2402:u32)
                  n782 = case shown="True" w2403 {
                    tunnel: w2402 -> [w2448 w2482]
                    tunnel: w2401 -> [w2447 w2481]
                    tunnel: w2406 -> [w2446 w2480]
                    tunnel: [w2445 w2479] -> w2398
                    tunnel: w2400 -> [w2442 w2476]
                    tunnel: w2404 -> [w2444 w2478]
                    tunnel: w2405 -> [w2443 w2477]
                    tunnel: w2399 -> [w2441 _]
                    frame True {
                      n783 = case shown="True" w2442 {
                        tunnel: w2448 -> [_ w2475]
                        tunnel: w2447 -> [_ w2464]
                        tunnel: w2446 -> [w2459 w2473]
                        tunnel: [w2461 w2474] -> w2445
                        tunnel: w2443 -> [w2462 _]
                        tunnel: w2444 -> [w2455 _]
                        tunnel: w2441 -> [w2450 w2465]
                        frame True {
                          n784 = Quotient & Remainder(x=w2459, y=u32 2) -> (x-y*floor(x/y)=w2457:u32)  [unwired: 1 out]
                          n785 = Greater?(x=w2450, y=u32 0) -> (0:w2453:bool)
                          n786 = Equal To 0?(x=w2457) -> (x = 0?=w2456:bool)
                          n787 = Select(t=w2450, s=w2453, f=u32 1) -> (s? t:f=w2452:u32)
                          n788 = Select(t=w2455, s=w2456, f=w2452) -> (s? t:f=w2454:u32)
                          n789 = To Long Integer(number=w2454) -> (32bit integer=w2460:i32)
                          n790 = Equal?(x=w2462, y=w2460) -> (x = y?=w2461:bool)
                        }
                        frame False {
                          n791 = Quotient & Remainder(x=w2473, y=u32 2) -> (x-y*floor(x/y)=w2471:u32, floor(x/y)=w2468:u32)
                          n792 = Add(x=w2464, y=w2465) -> (x+y=w2463:u32)
                          n793 = Multiply(x=w2471, y=w2465) -> (x*y=w2469:u32)
                          n794 = Multiply(x=w2468, y=w2463) -> (x*y=w2470:u32)
                          n795 = Add(x=w2470, y=w2469) -> (x+y=w2467:u32)
                          n796 = Add(x=w2464, y=w2467) -> (x+y=w2466:u32)
                          n797 = Greater Or Equal?(x=w2475, y=w2466) -> (x >= y?=w2474:bool)
                        }
                      }
                    }
                    frame False {
                      n798 = case shown="True" w2476 {
                        tunnel: w2482 -> [_ w2491]
                        tunnel: w2481 -> [_ w2490]
                        tunnel: w2480 -> [_ w2488]
                        tunnel: [w2484 w2487] -> w2479
                        tunnel: w2477 -> [w2485 _]
                        tunnel: w2478 -> [w2486 _]
                        frame True {
                          n799 = To Long Integer(number=w2486) -> (32bit integer=w2483:i32)
                          n800 = Equal?(x=w2485, y=w2483) -> (x = y?=w2484:bool)
                        }
                        frame False {
                          n801 = Increment(x=w2488) -> (x+1=w2489:u32)
                          n802 = Multiply(x=w2489, y=w2490) -> (x*y=w2492:u32)
                          n803 = Greater Or Equal?(x=w2491, y=w2492) -> (x >= y?=w2487:bool)
                        }
                      }
                    }
                  }
                  n804 = case shown="True" w2419 {
                    tunnel: w2439 -> [w2513 w2544]
                    tunnel: [w2514 w2543] -> w2431
                    tunnel: [w2513 w2542] -> w2430
                    tunnel: w2440 -> [w2514 w2541]
                    tunnel: w2438 -> [_ w2540]
                    tunnel: w2406 -> [_ w2539]
                    tunnel: w2427 -> [_ w2534]
                    tunnel: w2437 -> [w2512 w2538]
                    tunnel: w2436 -> [w2511 w2537]
                    tunnel: [w2512 w2536] -> w2433
                    tunnel: [w2511 w2535] -> w2432
                    tunnel: [w2510 w2533] -> w2429
                    tunnel: [w2509 w2532] -> w2428
                    tunnel: w2435 -> [w2510 _]
                    tunnel: w2434 -> [w2509 _]
                    tunnel: w2426 -> [w2508 _]
                    tunnel: [w2508 w2531] -> w2425
                    tunnel: w2417 -> [w2507 _]
                    tunnel: [w2507 w2530] -> w2416
                    tunnel: w2415 -> [w2506 w2529]
                    tunnel: [w2506 w2528] -> w2414
                    tunnel: w2413 -> [_ w2527]
                    tunnel: w2412 -> [_ w2526]
                    tunnel: w2410 -> [_ w2525]
                    tunnel: w2397 -> [_ w2524]
                    tunnel: w2409 -> [_ w2523]
                    tunnel: w2408 -> [_ w2522]
                    tunnel: w2405 -> [w2505 _]
                    tunnel: [w2505 0] -> w2407
                    tunnel: w2396 -> [_ w2520]
                    tunnel: w2395 -> [_ w2519]
                    tunnel: w2394 -> [_ w2518]
                    tunnel: w2393 -> [_ w2517]
                    tunnel: w2392 -> [_ w2516]
                    tunnel: w2391 -> [_ w2515]
                    frame False {
                    }
                    frame True {
                      n805 = stacked-sequence {
                        tunnel: w2544 -> [_ w2590 _ _]
                        tunnel: [_ w2589 _ _] -> w2543
                        tunnel: [_ w2588 _ _] -> w2542
                        tunnel: w2541 -> [_ w2587 _ _]
                        tunnel: w2540 -> [_ w2586 _ _]
                        tunnel: w2539 -> [_ w2585 _ _]
                        tunnel: w2538 -> [_ w2583 _ _]
                        tunnel: w2537 -> [_ w2582 _ _]
                        tunnel: [_ w2581 _ _] -> w2536
                        tunnel: [_ w2580 _ _] -> w2535
                        tunnel: w2534 -> [_ w2579 _ _]
                        tunnel: [_ w2578 _ _] -> w2533
                        tunnel: [_ w2577 _ _] -> w2532
                        tunnel: [_ w2575 _ _] -> w2531
                        tunnel: [_ _ _ w2625] -> w2530
                        tunnel: w2529 -> [_ w2562 _ _]
                        tunnel: [_ w2576 _ _] -> w2528
                        tunnel: w2527 -> [_ w2570 _ _]
                        tunnel: w2526 -> [_ w2574 _ _]
                        tunnel: w2525 -> [_ w2564 _ _]
                        tunnel: w2524 -> [_ w2563 _ _]
                        tunnel: w2523 -> [_ w2568 _ _]
                        tunnel: w2522 -> [_ w2567 _ _]
                        tunnel: w2520 -> [_ w2559 _ _]
                        tunnel: w2519 -> [w2548 _ w2619 _]
                        tunnel: w2518 -> [w2545 _ _ _]
                        tunnel: w2517 -> [w2547 _ w2621 _]
                        tunnel: w2516 -> [w2546 _ w2620 _]
                        tunnel: w2515 -> [_ w2558 _ _]
                        frame #0 {
                          n806 = case shown="True" w2548 {
                            tunnel: w2547 -> [_ w2552]
                            tunnel: w2546 -> [_ w2551]
                            tunnel: w2545 -> [_ w2549]
                            frame False {
                            }
                            frame True {
                              n807 = flat-sequence {
                                tunnel: w2552 -> [w2555]
                                tunnel: w2551 -> [w2554]
                                tunnel: [w2553] -> w2550
                                tunnel: w2549 -> [w2553]
                                tunnel: w2550 -> [w2557]
                                frame #0 {
                                n808 = VISA Write(VISA resource name=w2555, write buffer="OUT 1\nOUT OFF\n", error in (no error)=w2554) -> ()  [unwired: 3 out]
                                }
                                frame #1 {
                                n809 = Wait (ms)(milliseconds to wait=w2557) -> ()  [unwired: 1 out]
                                }
                              }
                            }
                          }
                        }
                        frame #1 {
                          n810 = To Long Integer(number=w2585) -> (32bit integer=w2584:i32)
                          n811 = Greater?(x=w2574, y=0) -> (0:w2572:bool)
                          n812 = Or(x=w2564, y=w2563) -> (x .or. y?=w2569:bool)
                          n813 = Or(x=w2562, y=w2564) -> (x .or. y?=w2565:bool)
                          n814 = Index Array(array=w2586, index (col)=w2584) -> (element=w2575:u8[])  [unwired: 1 in]
                          n815 = And(x=w2570, y=w2572) -> (x .and. y?=w2571:bool)
                          n816 = Or(x=w2569, y=w2559) -> (x .or. y?=w2560:bool)
                          n817 = Or(x=w2559, y=w2565) -> (x .or. y?=w2561:bool)
                          n818 = case shown="True" w2571 {
                            tunnel: w2575 -> [_ w2593]
                            frame False {
                            }
                            frame True {
                              n819 = control-ref of="XY Graph"() -> (w2591:refnum<vi>)
                              n820 = control-ref of="plot setting"() -> (w2592:refnum<vi>)
                              n821 = call "Plot Current.vi"("Current Mode"=w2593, "XY Graph REF"=w2591, "plot setting"=w2592) -> ()  [unwired: 9 in]
                            }
                          }
                          n822 = call "Arduino_a.vi"("Channel Number"=w2579, "error in (no error)"=w2590, "Current  Setting"=w2575, "Current Mode Count"=w2584, "VISA Refnum in"=w2587) -> ("error out"=w2588:errorcluster, "VISA Refnum out"=w2589:refnum<visa-resource-name>)  [unwired: 5 in]
                          n823 = case shown="True" w2561 {
                            tunnel: w2583 -> [w2604 w2614]
                            tunnel: w2582 -> [w2601 w2612]
                            tunnel: [w2600 w2613] -> w2581
                            tunnel: [w2597 w2611] -> w2580
                            tunnel: w2579 -> [w2603 w2618]
                            tunnel: [w2599 w2617] -> w2578
                            tunnel: [w2598 w2616] -> w2577
                            tunnel: w2575 -> [w2602 w2615]
                            tunnel: [FALSE ("Enable Accurate \nMeasure") w2609] -> w2576
                            tunnel: w2560 -> [w2595 _]
                            tunnel: w2568 -> [w2606 _]
                            tunnel: w2567 -> [w2596 _]
                            tunnel: [w2605 w2610] -> w2566
                            tunnel: w2559 -> [_ w2609]
                            tunnel: w2558 -> [w2594 w2608]
                            frame True {
                              n824 = call "Scan Initilize_ver2_2.vi"("VISA Refnum in"=w2604, "Scan Measure\nTime"=w2606, "Channel Count"=w2603, "Current Setting"=w2602, "error in (no error)"=w2601, "Sample number"=w2594, "Measure Maximun Voltage"=w2596, "Enable DMM Relay"=w2595) -> ("Current Channel"=w2605:string[], "VISA Refnum out"=w2600:refnum<visa-resource-name>, "P channel number"=w2599:i32, "N channel number"=w2598:i32, "error out"=w2597:errorcluster)  [unwired: 3 in]
                            }
                            frame False {
                              n825 = call "Scan Initilize_without Accurate Measure_ver2_2.vi"("Sample number"=w2608, "error in (no error)"=w2612, "Current Setting"=w2615, "Channel Count"=w2618, "VISA Refnum in"=w2614) -> ("error out"=w2611:errorcluster, "N channel number"=w2616:i32, "P channel number"=w2617:i32, "VISA Refnum out"=w2613:refnum<visa-resource-name>, "Current Channel"=w2610:string[])  [unwired: 2 in]
                            }
                          }
                          "Current channel\nindex" <- w2566
                        }
                        frame #2 {
                          n826 = case shown="True" w2619 {
                            tunnel: w2621 -> [_ w2623]
                            tunnel: w2620 -> [_ w2622]
                            frame False {
                            }
                            frame True {
                              n827 = VISA Write(VISA resource name=w2623, write buffer="OUT 1\nOUT ON\n", error in (no error)=w2622) -> ()  [unwired: 3 out]
                            }
                          }
                        }
                        frame #3 {
                          # "set \"Last Scan Time\"\nto the moment right after\nsending command 'a'"
                          n828 = Tick Count (ms)() -> (millisecond timer value=w2625:u32)
                        }
                      }
                    }
                  }
                  n829 = case shown="False" w2398 {
                    tunnel: [FALSE w2500] -> w2423
                    tunnel: [FALSE TRUE] -> w2422
                    tunnel: [w2493 w2498] -> w2421
                    tunnel: w2406 -> [w2493 w2497]
                    tunnel: w2420 -> [_ w2496]
                    frame False {
                    }
                    frame True {
                      n830 = Increment(x=w2497) -> (x+1=w2498:u32)
                      n831 = To Unsigned Long Integer(number=w2496) -> (unsigned 32bit integer=w2502:u32)
                      n832 = Greater Or Equal?(x=w2498, y=w2502) -> (x >= y?=w2501:bool)
                      n833 = case shown="True" w2501 {
                        tunnel: [FALSE TRUE] -> w2500
                        frame False {
                        }
                        frame True {
                        }
                      }
                    }
                  }
                }
              }
              n834 = Increment(x=w2016) -> (x+1=w2011:i32)
              n835 = case shown="True" w2096 {
                tunnel: w2100 -> [_ w2647]
                tunnel: w2057 -> [_ w2644]
                tunnel: w2099 -> [_ w2628]
                tunnel: [FALSE w2643] -> w2098
                tunnel: w2097 -> [_ w2642]
                tunnel: w2056 -> [_ w2629]
                tunnel: w2064 -> [_ w2641]
                tunnel: w2051 -> [_ w2630]
                tunnel: w2070 -> [_ w2635]
                tunnel: w2095 -> [_ w2633]
                tunnel: [FALSE w2632] -> w2094
                frame False {
                }
                frame True {
                  n836 = case shown="True" w2633 {
                    tunnel: w2630 -> [w2665 w2672]
                    tunnel: w2641 -> [w2664 w2669]
                    tunnel: [0 w2670] -> w2646
                    tunnel: [w2666 w2669] -> w2645
                    tunnel: [w2663 TRUE] -> w2632
                    frame False {
                      n837 = Greater Or Equal?(x=w2665, y=w2664) -> (x >= y?=w2663:bool)
                      n838 = Increment(x=w2665) -> (x+1=w2666:i32)
                    }
                    frame True {
                      n839 = Subtract(x=w2672, y=w2669) -> (x-y=w2671:i32)
                      n840 = Increment(x=w2671) -> (x+1=w2670:i32)
                    }
                  }
                  n841 = for {
                    N: w2647 -> [_]
                    tunnel: w2644 -> [w2679] mode=indexing
                    tunnel: w2629 -> [w2676]
                    tunnel: w2646 -> [w2674]
                    tunnel: w2645 -> [w2673]
                    tunnel: [w2677] -> w2631 mode=indexing
                    n842 = Array Subset(array=w2676, index=w2674, length=w2673) -> (w2675:dbl[])
                    n843 = Array Subset(array=w2679, index=w2674, length=w2673) -> (w2678:dbl[])
                    n844 = Bundle(w2675, w2678) -> (w2677:cluster{dbl[], dbl[]})  [unwired: 1 in]
                  }
                  "XY Graph" <- w2631
                  n845 = Greater Or Equal?(x=w2635, y=u32 25) -> (x >= y?=w2639:bool)
                  n846 = case shown="False" w2642 {
                    tunnel: w2628 -> [_ w2661]
                    tunnel: [TRUE w2660] -> w2643
                    tunnel: w2630 -> [_ w2659]
                    tunnel: w2629 -> [_ w2658]
                    frame True {
                    }
                    frame False {
                      # "Enable dynamically plot"
                      n847 = Index Array(array=w2658, index=w2659) -> (element=w2662:dbl)
                      n848 = Greater Or Equal?(x=w2662, y=w2661) -> (x >= y?=w2660:bool)
                    }
                  }
                  n849 = Select(t=1, s=w2639, f=3) -> (s? t:f=w2636:i32)
                  n850 = Quotient & Remainder(x=w2630, y=w2636) -> (x-y*floor(x/y)=w2640:i32)  [unwired: 1 out]
                  n851 = case shown="0" w2640 {
                    tunnel: w2642 -> [_ w2651]
                    tunnel: w2629 -> [_ w2650]
                    tunnel: w2630 -> [_ w2649]
                    tunnel: w2628 -> [_ w2648]
                    frame Default {
                    }
                    frame 0 {
                      n852 = case shown="True" w2651 {
                        tunnel: w2650 -> [_ w2656]
                        tunnel: w2649 -> [_ w2655]
                        tunnel: w2648 -> [_ w2653]
                        frame False {
                        }
                        frame True {
                          n853 = Index Array(array=w2656, index=w2655) -> (element=w2654:dbl)
                          n854 = Subtract(x=w2654, y=w2653) -> (x-y=w2652:dbl)
                          n855 = property on="XY Graph" class="XYGraph (strict)"("XScale.Maximum"=w2654, "XScale.Minimum"=w2652) -> ()  [unwired: 2 in, 2 out]
                        }
                      }
                    }
                  }
                }
              }
              n856 = Increment(x=w2051) -> (x+1=w2010:i32)
              n857 = flat-sequence {
                tunnel: w2085 -> [w2139]
                tunnel: w2084 -> [w2138]
                tunnel: w2083 -> [w2137]
                tunnel: w2082 -> [w2136]
                tunnel: w2081 -> [w2135]
                tunnel: [w2134] -> w2080
                tunnel: [w2133] -> w2079
                tunnel: [w2132] -> w2000
                tunnel: [w2131] -> w2002
                tunnel: w2078 -> [w2130]
                tunnel: w2077 -> [w2129]
                tunnel: w2030 -> [w2109]
                tunnel: w2075 -> [w2128]
                tunnel: [w2104] -> w2074
                tunnel: w2010 -> [w2120]
                tunnel: w2057 -> [w2125]
                tunnel: [w2127] -> w2062
                tunnel: w1998 -> [w2124]
                tunnel: w2023 -> [w2106]
                tunnel: w1994 -> [w2126]
                tunnel: w2054 -> [w2123]
                tunnel: w2049 -> [w2121]
                tunnel: w2024 -> [w2118]
                tunnel: [w2117] -> w2009
                tunnel: [w2113] -> w2047
                tunnel: [w2112] -> w2046
                tunnel: [w2111] -> w2045
                tunnel: w2033 -> [w2110]
                tunnel: w2029 -> [w2108]
                tunnel: [w2107] -> w2012
                tunnel: [w2105] -> w2008
                tunnel: [w2105] -> w2020
                tunnel: [w2102] -> w1992
                tunnel: [w2101] -> w1985
                tunnel: w2065 -> [w2232]
                tunnel: w2010 -> [w2229]
                tunnel: w2056 -> [w2231]
                tunnel: [w2230] -> w2061
                tunnel: w2047 -> [w2228]
                tunnel: w2046 -> [w2227]
                tunnel: w2045 -> [w2224]
                tunnel: w2044 -> [w2225]
                tunnel: w2043 -> [w2223]
                tunnel: [w2222] -> w2040
                tunnel: w2009 -> [w2221]
                tunnel: w2042 -> [w2220]
                tunnel: [w2219] -> w2039
                tunnel: w2041 -> [w2218]
                tunnel: [w2217] -> w2038
                tunnel: w2013 -> [w2272]
                tunnel: w2012 -> [w2271]
                tunnel: w2011 -> [w2270]
                tunnel: w2010 -> [w2269]
                tunnel: w2009 -> [w2268]
                tunnel: w2008 -> [w2267]
                tunnel: [w2266] -> w2007
                tunnel: [w2265] -> w2006
                tunnel: [w2264] -> w2005
                tunnel: [w2263] -> w2004
                tunnel: w1985 -> [w2262]
                tunnel: [w2261] -> w2003
                tunnel: w2002 -> [w2260]
                tunnel: w2000 -> [w2259]
                tunnel: [w2258] -> w2001
                tunnel: [w2257] -> w1999
                tunnel: w1995 -> [w2256]
                tunnel: [w2255] -> w1996
                tunnel: w2064 -> [w2347]
                tunnel: w2063 -> [w2346]
                tunnel: w2062 -> [w2345]
                tunnel: w2061 -> [w2344]
                tunnel: [w2343] -> w2058
                tunnel: [w2342] -> w2059
                tunnel: [w2341] -> w2060
                tunnel: w2027 -> [w2340]
                tunnel: w2005 -> [w2330]
                tunnel: w2055 -> [w2338]
                tunnel: w2049 -> [w2334]
                tunnel: [w2333] -> w2053
                tunnel: [w2332] -> w2026
                tunnel: w2003 -> [w2331]
                tunnel: w2070 -> [w2385]
                tunnel: w2069 -> [w2384]
                tunnel: [w2383] -> w2068
                frame #0 {
                  n858 = And(x=w2126, y=w2106) -> (x .and. y?=w2114:bool)
                  n859 = case shown="True" w2114 {
                    tunnel: w2125 -> [_ w2157]
                    tunnel: w2124 -> [_ w2156]
                    tunnel: w2123 -> [_ w2144]
                    tunnel: [T9 {"Enable DMM\n Relay"=FALSE, "Measure Current \nOnly"=FALSE, [], 0} w2155] -> w2122
                    tunnel: w2121 -> [_ w2151]
                    tunnel: w2120 -> [_ w2147]
                    tunnel: [FALSE w2143] -> w2119
                    tunnel: [FALSE w2143] -> w2116
                    tunnel: w2109 -> [_ w2149]
                    frame False {
                      # "No meaning"
                      # "No meaning"
                    }
                    frame True {
                      # "Run command \"b\"\nto get V value first"
                      n860 = Decrement(x=w2147) -> (x-1=w2152:i32)
                      n861 = Index Array(array=w2151, index=w2147) -> (element=w2154:u32)
                      n862 = Index Array(array=w2151, index=w2152) -> (element=w2153:u32)
                      n863 = Equal To 0?(x=w2147) -> (x = 0?=w2146:bool)
                      n864 = Not Equal?(x=w2154, y=w2153) -> (x != y?=w2148:bool)
                      n865 = Or(x=w2148, y=w2146) -> (x .or. y?=w2145:bool)
                      n866 = Index Array(array=w2157, index (col)=w2152) -> (element=w2150:dbl[])  [unwired: 1 in]
                      n867 = And(x=w2145, y=w2144) -> (x .and. y?=w2143:bool)
                      n868 = Bundle("Enable DMM\n Relay"=w2156, "Measure Current \nOnly"=w2144, w2150, w2149) -> (w2155:T9)  [unwired: 1 in]
                    }
                  }
                  n869 = Not(x=w2116) -> (.not. x?=w2115:bool)
                  n870 = And(x=w2114, y=w2115) -> (x .and. y?=w2111:bool)
                  n871 = case shown="False" w2111 {
                    tunnel: w2139 -> [w2178 w2202]
                    tunnel: w2138 -> [w2188 w2213]
                    tunnel: w2137 -> [w2187 w2212]
                    tunnel: w2136 -> [w2186 w2211]
                    tunnel: w2135 -> [w2185 w2210]
                    tunnel: [w2184 w2209] -> w2131
                    tunnel: [w2183 w2208] -> w2132
                    tunnel: [w2182 w2207] -> w2133
                    tunnel: [w2166 w2206] -> w2134
                    tunnel: w2130 -> [w2181 w2205]
                    tunnel: w2129 -> [w2180 w2204]
                    tunnel: w2128 -> [w2179 w2203]
                    tunnel: [w2171 w2198] -> w2104
                    tunnel: w2125 -> [w2177 w2201]
                    tunnel: w2120 -> [w2176 w2200]
                    tunnel: [w2174 w2199] -> w2127
                    tunnel: w2122 -> [_ w2195]
                    tunnel: [w2170 w2197] -> w2112
                    tunnel: [w2170 w2196] -> w2113
                    tunnel: w2110 -> [w2169 w2194]
                    tunnel: w2108 -> [w2168 _]
                    tunnel: [w2167 w2190] -> w2107
                    tunnel: [w2163 w2190] -> w2101
                    frame False {
                      w2170 = dbl[] [] ("Accurate Data")
                      n872 = call "Scan_ver2_2.vi"("DMM ref"=w2188, "output cluster"=w2168, "P_current_count"=w2181, "N_current_count"=w2180, "DMM error"=w2187, "Current Sense \nResitance Array"=w2169, "ESP32 ref"=w2186, "ESP32 error"=w2185, "current_mode"=w2179) -> ("DMM ref"=w2184:refnum<visa-resource-name>, "DMM error"=w2183:errorcluster, "Measurements"=w2175:dbl[], "ESP32 ref"=w2182:refnum<visa-resource-name>, "Timout?"=w2167:bool, "Time out count"=w2165:i32, "ESP32 error"=w2166:errorcluster)
                      n873 = Greater?(x=w2165, y=0) -> (0:w2173:bool)
                      n874 = Greater?(x=w2165, y=10) -> (0:w2163:bool)
                      n875 = Replace Array Subset(array=w2177, new element=w2175, index (col)=w2176) -> (w2174:dbl[][])  [unwired: 1 in]
                      n876 = Add(x=w2165, y=w2178) -> (x+y=w2171:i32)
                      n877 = case shown="True" w2173 {
                        tunnel: w2171 -> [_ w2189]
                        frame False {
                        }
                        frame True {
                          "Time out count:" <- w2189
                        }
                      }
                    }
                    frame True {
                      n878 = call "Accurate Measure With Setting_ver2_2.vi"("DMM ref in"=w2213, "Accurate Measure Setting"=w2195, "P_current_count"=w2205, "N_current_count"=w2204, "DMM error in"=w2212, "Current Sense \nResitance Array"=w2194, "ESP32 ref in"=w2211, "ESP32 error in"=w2210, "current_mode"=w2203) -> ("DMM ref out"=w2209:refnum<visa-resource-name>, "DMM error out"=w2208:errorcluster, "Accurate Data"=w2197:dbl[], "ESP32 ref out"=w2207:refnum<visa-resource-name>, "time_out_count"=w2191:i32, "Standard Deviation of Data"=w2196:dbl[], "ESP32 error out"=w2206:errorcluster)
                      n879 = Greater Than 0?(x=w2191) -> (x > 0?=w2192:bool)
                      n880 = Replace Array Subset(array=w2201, new element=w2197, index (col)=w2200) -> (w2199:dbl[][])  [unwired: 1 in]
                      n881 = Add(x=w2191, y=w2202) -> (x+y=w2198:i32)
                      n882 = case shown="True" w2192 {
                        tunnel: w2198 -> [_ w2214]
                        frame False {
                        }
                        frame True {
                          n883 = local write "Time out count:"(w2214) -> ()
                        }
                      }
                      n884 = Greater?(x=w2191, y=10) -> (0:w2190:bool)
                    }
                  }
                  n885 = case shown="True" w2119 {
                    tunnel: w2118 -> [w2159 w2162]
                    tunnel: [w2159 w2161] -> w2117
                    tunnel: w2106 -> [w2158 _]
                    tunnel: [w2158 FALSE] -> w2105
                    frame False {
                    }
                    frame True {
                      # "run command \"b\" first\nthen accurate measure current\nin the next run"
                      n886 = Decrement(x=w2162) -> (x-1=w2161:u32)
                    }
                  }
                  n887 = Greater?(x=w2104, y=100000) -> (0:w2102:bool)
                }
                frame #1 {
                  n888 = Decrement(x=w2221) -> (x-1=w2215:u32)
                  n889 = And(x=w2225, y=w2224) -> (x .and. y?=w2226:bool)
                  n890 = Tick Count (ms)() -> (millisecond timer value=w2233:u32)
                  n891 = Subtract(x=w2233, y=w2232) -> (x-y=w2234:u32)
                  n892 = To Double Precision Float(number=w2234) -> (double precision float=w2236:dbl)
                  n893 = Divide(x=w2236, y=1000.0) -> (x/y=w2216:dbl)
                  n894 = case shown="True" w2226 {
                    tunnel: w2223 -> [w2239 w2254]
                    tunnel: w2215 -> [_ w2243]
                    tunnel: [w2239 w2250] -> w2222
                    tunnel: w2228 -> [_ w2249]
                    tunnel: w2227 -> [_ w2248]
                    tunnel: w2220 -> [w2238 w2247]
                    tunnel: [w2238 w2241] -> w2219
                    tunnel: w2218 -> [w2237 w2246]
                    tunnel: [w2237 w2240] -> w2217
                    tunnel: w2216 -> [_ w2242]
                    frame False {
                    }
                    frame True {
                      n895 = To Long Integer(number=w2243) -> (32bit integer=w2252:i32)
                      n896 = Multiply(x=w2252, y=2) -> (x*y=w2245:i32)
                      n897 = Increment(x=w2245) -> (x+1=w2244:i32)
                      n898 = Replace Array Subset(array=w2254, new element=w2248, index (col)=w2245) -> (w2251:dbl[][])  [unwired: 1 in]
                      n899 = Replace Array Subset(array=w2251, new element=w2249, index (col)=w2244) -> (w2250:dbl[][])  [unwired: 1 in]
                      n900 = Replace Array Subset(array=w2247, new element=w2242, index=w2245) -> (w2241:dbl[])
                      n901 = Replace Array Subset(array=w2246, new element=w2243, index=w2245) -> (w2240:u32[])
                    }
                  }
                  n902 = Replace Array Subset(array=w2231, new element=w2216, index=w2229) -> (w2230:dbl[])
                }
                frame #2 {
                  # "Serious time out\ncause by lost connetion"
                  n903 = And(x=w2272, y=w2271) -> (x .and. y?=w2273:bool)
                  n904 = case shown="True" w2273 {
                    tunnel: w2269 -> [w2278 w2296]
                    tunnel: [w2278 w2290] -> w2264
                    tunnel: w2270 -> [w2280 w2295]
                    tunnel: [w2280 w2289] -> w2263
                    tunnel: w2267 -> [w2277 w2293]
                    tunnel: [w2277 w2294] -> w2266
                    tunnel: w2268 -> [w2279 w2292]
                    tunnel: [w2279 w2291] -> w2265
                    tunnel: w2262 -> [_ w2288]
                    tunnel: [w2277 w2287] -> w2261
                    tunnel: w2260 -> [w2276 w2286]
                    tunnel: w2259 -> [w2275 w2285]
                    tunnel: [w2276 w2284] -> w2258
                    tunnel: [w2275 w2283] -> w2257
                    tunnel: w2256 -> [w2274 w2282]
                    tunnel: [w2274 w2281] -> w2255
                    frame False {
                    }
                    frame True {
                      n905 = case shown="True" w2288 {
                        tunnel: w2296 -> [w2306 w2326]
                        tunnel: w2295 -> [w2304 w2325]
                        tunnel: [TRUE w2319] -> w2294
                        tunnel: w2293 -> [w2311 w2324]
                        tunnel: w2292 -> [w2310 w2323]
                        tunnel: [w2309 w2322] -> w2291
                        tunnel: [w2305 w2321] -> w2290
                        tunnel: [0 w2320] -> w2289
                        tunnel: [FALSE w2319] -> w2287
                        tunnel: w2286 -> [w2303 w2318]
                        tunnel: w2285 -> [_ w2317]
                        tunnel: [w2302 w2318] -> w2284
                        tunnel: [w2301 w2317] -> w2283
                        tunnel: w2282 -> [_ w2316]
                        tunnel: [TRUE w2316] -> w2281
                        frame True {
                          n906 = local read "Switch On Time"() -> (w2298:u8)
                          n907 = Subtract(x=w2306, y=w2304) -> (x-y=w2305:i32)
                          n908 = case shown="True" w2311 {
                            tunnel: w2310 -> [w2313 w2315]
                            tunnel: [w2313 w2314] -> w2309
                            frame False {
                            }
                            frame True {
                              n909 = Decrement(x=w2315) -> (x-1=w2314:u32)
                            }
                          }
                          n910 = Multiply(x=w2298, y=1e-06) -> (x*y=w2297:dbl)
                          n911 = call "DMM Scan Reset_4.vi"("Manual Trigger Delay (1 s)"=w2297, "VISA in resource name"=w2303) -> ("error out"=w2301:errorcluster, "VISA resource name out"=w2302:refnum<visa-resource-name>)  [unwired: 8 in]
                        }
                        frame False {
                          w2319 = FALSE
                          n912 = case shown="True" w2324 {
                            tunnel: w2323 -> [w2327 w2329]
                            tunnel: [w2327 w2328] -> w2322
                            frame False {
                            }
                            frame True {
                              n913 = Decrement(x=w2329) -> (x-1=w2328:u32)
                            }
                          }
                          n914 = Decrement(x=w2325) -> (x-1=w2320:i32)
                          n915 = Decrement(x=w2326) -> (x-1=w2321:i32)
                        }
                      }
                    }
                  }
                }
                frame #3 {
                  n916 = Greater?(x=w2330, y=w2338) -> (0:w2339:bool)
                  n917 = And(x=w2331, y=w2339) -> (x .and. y?=w2335:bool)
                  n918 = Greater Or Equal?(x=w2330, y=w2346) -> (x >= y?=w2336:bool)
                  n919 = Or(x=w2336, y=w2335) -> (x .or. y?=w2337:bool)
                  n920 = case shown="True" w2337 {
                    tunnel: w2330 -> [w2352 w2372]
                    tunnel: [w2352 w2360] -> w2343
                    tunnel: w2347 -> [_ w2371]
                    tunnel: w2345 -> [w2351 w2373]
                    tunnel: [w2351 w2370] -> w2342
                    tunnel: w2344 -> [w2350 w2369]
                    tunnel: [w2350 w2368] -> w2341
                    tunnel: w2340 -> [w2348 w2361]
                    tunnel: w2334 -> [w2349 w2359]
                    tunnel: [w2349 w2356] -> w2333
                    tunnel: [w2348 w2353] -> w2332
                    frame False {
                    }
                    frame True {
                      n921 = Decrement(x=w2371) -> (x-1=w2360:i32)
                      n922 = Subtract(x=w2372, y=w2360) -> (x-y=w2358:i32)
                      n923 = in-place {
                        in-place-border: [w2380] -> w2367
                        n924 = in-place-split #2(w2373, w2358) -> (w2380:dbl[][], w2382:dbl[][])
                        n925 = in-place-split #2(w2382, dbl[][] [] ("element")) -> (w2370:dbl[][])  [unwired: 1 out]
                      }
                      n926 = in-place {
                        in-place-border: [w2374] -> w2357
                        n927 = in-place-split #3(w2359, w2358) -> (w2374:u32[], w2376:u32[])
                        n928 = in-place-split #3(w2376, dbl[] [] ("element")) -> (w2356:u32[])  [unwired: 1 out]
                      }
                      n929 = To Double Precision Float(number=w2357) -> (double precision float=w2354:dbl[])
                      n930 = in-place {
                        in-place-border: [w2377] -> w2355
                        n931 = in-place-split #4(w2369, w2358) -> (w2377:dbl[], w2379:dbl[])
                        n932 = in-place-split #4(w2379, dbl[] [] ("element")) -> (w2368:dbl[])  [unwired: 1 out]
                      }
                      n933 = Build Array (concatenate)(w2355, w2354, w2367) -> (w2362:dbl[][])
                      n934 = call-poly <vilib>:"Write Delimited Spreadsheet.vi"("file path (dialog if empty)"=w2361, "format (%.3f)"="%.9f", "2D data"=w2362, "append to file? (new file:F)"=TRUE, "transpose? (no:F)"=TRUE, "delimiter (\\t)"="," ("delimiter (\\t)")) -> ("new file path (Not A Path if cancelled)"=w2353:path)  [unwired: 8 in, 1 out]
                    }
                  }
                }
                frame #4 {
                  n935 = while {
                    tunnel: w2385 -> [w2388]
                    tunnel: w2384 -> [w2390]
                    tunnel: [w2387] -> w2383
                    tunnel: [w2386] -> _
                    stop <- w2389 stop-if-true
                    n936 = Tick Count (ms)() -> (millisecond timer value=w2387:u32)
                    n937 = Subtract(x=w2387, y=w2390) -> (x-y=w2386:u32)
                    n938 = Greater Or Equal?(x=w2386, y=w2388) -> (x >= y?=w2389:bool)
                  }
                }
              }
              n939 = Bundle("y"=w1987, w2030, "Sample Number"=w1986) -> (w2029:cluster{"y":i32, i32, "Sample Number":i32})  [unwired: 1 in]
              n940 = And(x=w2020, y=w2022) -> (x .and. y?=w2021:bool)
              n941 = local read "Leave"() -> (w2036:bool)
              n942 = Or(x="Scan Stop", y=w2021) -> (x .or. y?=w2035:bool)
              n943 = Or(x=w2036, y=w2035) -> (x .or. y?=w2034:bool)
              n944 = Or(x=w2034, y=w1992) -> (x .or. y?=w1993:bool)
            }
            n945 = Increment(x=w1916) -> (x+1=w1915:i32)
          }
        }
        n946 = call <vilib>:"Open Config Data.vi"("error in (no error)"=w1104, "configuration file path"=w1103) -> ("error out"=w1156:errorcluster, "refnum"=w1155:T8)  [unwired: 7 in, 1 out]
        n947 = local read "Constant Scan Number"() -> (w1158:bool)
        n948 = call-poly <vilib>:"Write Key.vi"("section"=w971, "error in (no error)"=w1156, "value"=w1157, "key"="Neglect Timeout Data" ("Label.Text"), "refnum"=w1155) -> ("error out"=w1124:errorcluster, "refnum out"=w1123:T8)  [unwired: 4 in, 1 out]
        n949 = call-poly <vilib>:"Write Key.vi"("section"=w971, "error in (no error)"=w1124, "value"=w1158, "key"="Constant Scan Number" ("Label.Text"), "refnum"=w1123) -> ("error out"=w1152:errorcluster, "refnum out"=w1151:T8)  [unwired: 4 in, 1 out]
        n950 = local read "Scan Number"() -> (w1159:u32)
        n951 = call-poly <vilib>:"Write Key.vi"("section"=w971, "error in (no error)"=w1152, "value"=w1159, "key"="Scan Number" ("Label.Text"), "refnum"=w1151) -> ("error out"=w1154:errorcluster, "refnum out"=w1153:T8)  [unwired: 4 in, 1 out]
        n952 = local read "Enable Accurate \nMeasure"() -> (w1160:bool)
        n953 = call-poly <vilib>:"Write Key.vi"("section"=w971, "error in (no error)"=w1154, "value"=w1160, "key"="Enable Accurate Measure" ("Label.Text"), "refnum"=w1153) -> ("error out"=w1126:errorcluster, "refnum out"=w1125:T8)  [unwired: 4 in, 1 out]
        n954 = local read "Enable DMM\n Relay"() -> (w1161:bool)
        n955 = call-poly <vilib>:"Write Key.vi"("section"=w971, "error in (no error)"=w1126, "value"=w1161, "key"="Enable DMM Relay" ("Label.Text"), "refnum"=w1125) -> ("error out"=w1128:errorcluster, "refnum out"=w1127:T8)  [unwired: 4 in, 1 out]
        n956 = local read "Measure Current \nOnly"() -> (w1162:bool)
        n957 = call-poly <vilib>:"Write Key.vi"("section"=w971, "error in (no error)"=w1128, "value"=w1162, "key"="Measure Current Only" ("Label.Text"), "refnum"=w1127) -> ("error out"=w1130:errorcluster, "refnum out"=w1129:T8)  [unwired: 4 in, 1 out]
        n958 = local read "Record Accurate \nData Only"() -> (w1100:bool)
        n959 = call-poly <vilib>:"Write Key.vi"("section"=w971, "error in (no error)"=w1130, "value"=w1100, "key"="Record Accurate Data Only" ("Label.Text"), "refnum"=w1129) -> ("error out"=w1132:errorcluster, "refnum out"=w1131:T8)  [unwired: 4 in, 1 out]
        n960 = local read "Remote\nPSU"() -> (w1163:bool)
        n961 = call-poly <vilib>:"Write Key.vi"("section"=w971, "error in (no error)"=w1132, "value"=w1163, "key"="Remote PSU" ("Label.Text"), "refnum"=w1131) -> ("error out"=w1134:errorcluster, "refnum out"=w1133:T8)  [unwired: 4 in, 1 out]
        n962 = local read "Output Max Voltage"() -> (w1101:dbl)
        n963 = call-poly <vilib>:"Write Key.vi"("section"=w971, "error in (no error)"=w1134, "value"=w1101, "key"="Output Max Voltage" ("Label.Text"), "refnum"=w1133) -> ("error out"=w1136:errorcluster, "refnum out"=w1135:T8)  [unwired: 4 in, 1 out]
        n964 = local read "Output Max Current"() -> (w1102:dbl)
        n965 = call-poly <vilib>:"Write Key.vi"("section"=w971, "error in (no error)"=w1136, "value"=w1102, "key"="Output Max Current" ("Label.Text"), "refnum"=w1135) -> ("error out"=w974:errorcluster, "refnum out"=w975:T8)  [unwired: 4 in, 1 out]
        n966 = local read "safe Mode?"() -> (w989:bool)
        n967 = call-poly <vilib>:"Write Key.vi"("section"=w971, "error in (no error)"=w974, "value"=w989, "key"="safe Mode?" ("Label.Text"), "refnum"=w975) -> ("error out"=w991:errorcluster, "refnum out"=w990:T8)  [unwired: 4 in, 1 out]
        n968 = local read "PSU Buffer Time"() -> (w988:u32)
        n969 = call-poly <vilib>:"Write Key.vi"("section"=w971, "error in (no error)"=w991, "value"=w988, "key"="PSU Buffer Time" ("Label.Text"), "refnum"=w990) -> ("error out"=w993:errorcluster, "refnum out"=w992:T8)  [unwired: 4 in, 1 out]
        n970 = local read "Waiting\nTime"() -> (w987:u32)
        n971 = call-poly <vilib>:"Write Key.vi"("section"=w971, "error in (no error)"=w993, "value"=w987, "key"="Waiting Time" ("Label.Text"), "refnum"=w992) -> ("error out"=w995:errorcluster, "refnum out"=w994:T8)  [unwired: 4 in, 1 out]
        n972 = local read "Switch On Time"() -> (w986:u8)
        n973 = call-poly <vilib>:"Write Key.vi"("section"=w971, "error in (no error)"=w995, "value"=w986, "key"="Switch On Time" ("Label.Text"), "refnum"=w994) -> ("error out"=w997:errorcluster, "refnum out"=w996:T8)  [unwired: 4 in, 1 out]
        n974 = local read "Switch Off Time"() -> (w985:u8)
        n975 = call-poly <vilib>:"Write Key.vi"("section"=w971, "error in (no error)"=w997, "value"=w985, "key"="Switch Off Time" ("Label.Text"), "refnum"=w996) -> ("error out"=w999:errorcluster, "refnum out"=w998:T8)  [unwired: 4 in, 1 out]
        n976 = local read "Sample Mode"() -> (w984:u16)
        n977 = call-poly <vilib>:"Write Key.vi"("section"=w971, "error in (no error)"=w999, "value"=w984, "key"="Sample Mode" ("Label.Text"), "refnum"=w998) -> ("error out"=w1001:errorcluster, "refnum out"=w1000:T8)  [unwired: 4 in, 1 out]
        n978 = local read "Sample Number"() -> (w983:i32)
        n979 = call-poly <vilib>:"Write Key.vi"("section"=w971, "error in (no error)"=w1001, "value"=w983, "key"="Sample Number" ("Label.Text"), "refnum"=w1000) -> ("error out"=w972:errorcluster, "refnum out"=w973:T8)  [unwired: 4 in, 1 out]
        n980 = local read "Array Mode"() -> (w1164:u16)
        n981 = call-poly <vilib>:"Write Key.vi"("section"=w971, "error in (no error)"=w972, "value"=w1164, "key"="Array Mode" ("Label.Text"), "refnum"=w973) -> ("error out"=w1138:errorcluster, "refnum out"=w1137:T8)  [unwired: 4 in, 1 out]
        n982 = local read "Electrode number, N"() -> (w1165:u16)
        n983 = call-poly <vilib>:"Write Key.vi"("section"=w971, "error in (no error)"=w1138, "value"=w1165, "key"="Electrode number, N" ("Label.Text"), "refnum"=w1137) -> ("error out"=w1140:errorcluster, "refnum out"=w1139:T8)  [unwired: 4 in, 1 out]
        n984 = local read "Current Channel"() -> (w1166:string)
        n985 = call-poly <vilib>:"Write Key.vi"("section"=w971, "error in (no error)"=w1140, "value"=w1166, "key"="Current Channel" ("Label.Text"), "refnum"=w1139) -> ("error out"=w1142:errorcluster, "refnum out"=w1141:T8)  [unwired: 4 in, 1 out]
        n986 = local read "Insert\nBreak"() -> (w1167:bool)
        n987 = call-poly <vilib>:"Write Key.vi"("section"=w971, "error in (no error)"=w1142, "value"=w1167, "key"="Insert Break" ("Label.Text"), "refnum"=w1141) -> ("error out"=w1144:errorcluster, "refnum out"=w1143:T8)  [unwired: 4 in, 1 out]
        n988 = local read "Break Period Multipier"() -> (w1168:dbl)
        n989 = call-poly <vilib>:"Write Key.vi"("section"=w971, "error in (no error)"=w1144, "value"=w1168, "key"="Break Period Multipier" ("Label.Text"), "refnum"=w1143) -> ("error out"=w1146:errorcluster, "refnum out"=w1145:T8)  [unwired: 4 in, 1 out]
        n990 = local read "Only Use Last Value?"() -> (w1169:bool)
        n991 = call-poly <vilib>:"Write Key.vi"("section"=w971, "error in (no error)"=w1146, "value"=w1169, "key"="Only Use Last Value?" ("Label.Text"), "refnum"=w1145) -> ("error out"=w1148:errorcluster, "refnum out"=w1147:T8)  [unwired: 4 in, 1 out]
        n992 = local read "Inverse\nPolarity"() -> (w1170:bool)
        n993 = call-poly <vilib>:"Write Key.vi"("section"=w971, "error in (no error)"=w1148, "value"=w1170, "key"="Inverse Polarity" ("Label.Text"), "refnum"=w1147) -> ("error out"=w1150:errorcluster, "refnum out"=w1149:T8)  [unwired: 4 in, 1 out]
        n994 = local read "Wait Current Stable Period"() -> (w1171:i32)
        n995 = call-poly <vilib>:"Write Key.vi"("section"=w971, "error in (no error)"=w1150, "value"=w1171, "key"="Wait Current Stable Period" ("Label.Text"), "refnum"=w1149) -> ("error out"=w1096:errorcluster, "refnum out"=w1097:T8)  [unwired: 4 in, 1 out]
        n996 = local read "Save\nRaw Data"() -> (w1092:bool)
        n997 = call-poly <vilib>:"Write Key.vi"("section"=w971, "error in (no error)"=w1096, "value"=w1092, "key"="Save Raw Data" ("Label.Text"), "refnum"=w1097) -> ("error out"=w1093:errorcluster, "refnum out"=w1094:T8)  [unwired: 4 in, 1 out]
        n998 = call <vilib>:"Close Config Data.vi"("error in (no error)"=w1093, "refnum"=w1094) -> ()  [unwired: 8 in, 2 out]
        n999 = local read "Enable Accurate \nMeasure"() -> (w1022:bool)
        n1000 = property on="Scan Stop" class="Bool (strict)"("DisabledEnum"=w1020) -> ()  [unwired: 2 in, 2 out]
        n1001 = local read "Sample Mode"() -> (w1024:u16)
        n1002 = local write "Scan Stop"(w1004) -> ()
        n1003 = property on="Leave" class="Bool (strict)"("DisabledEnum"=w1008) -> ()  [unwired: 2 in, 2 out]
        n1004 = Array Subset(array=w1028, index (col)=w1037, length (col)=w1011) -> (w1070:dbl[][])  [unwired: 2 in]
        n1005 = Array Subset(array=w1027, index=w1037, length=w1011) -> (w1062:dbl[])
        n1006 = Array Subset(array=w1026, index=w1037, length=w1011) -> (w1064:u32[])
        n1007 = To Double Precision Float(number=w1064) -> (double precision float=w1063:dbl[])
        n1008 = Equal To 0?(x=w1024) -> (x = 0?=w1023:bool)
        n1009 = Build Array (concatenate)(w1062, w1063, w1070) -> (w1060:dbl[][])
        n1010 = To Double Precision Float(number=w1029) -> (double precision float=w1061:dbl[])
        n1011 = local read "channel count"() -> (w1058:i32)
        n1012 = And(x=w1023, y=w1022) -> (x .and. y?=w1021:bool)
        n1013 = call-poly <vilib>:"Write Delimited Spreadsheet.vi"("file path (dialog if empty)"=w1032, "format (%.3f)"="%.9f", "2D data"=w1060, "append to file? (new file:F)"=TRUE, "transpose? (no:F)"=TRUE, "delimiter (\\t)"="," ("delimiter (\\t)")) -> ("new file path (Not A Path if cancelled)"=w1049:path, "error out"=w1051:errorcluster)  [unwired: 8 in]
        n1014 = VISA Write(VISA resource name=w1007, write buffer="DISP ON", error in (no error)=w1006) -> (VISA resource name out=w1066:refnum<visa-resource-name>, error out=w1065:errorcluster)  [unwired: 1 out]
        n1015 = call <instrlib>:"Error Query.vi"("error in (no error)"=w1065, "VISA resource name"=w1066) -> ("error out"=w1067:errorcluster, "VISA resource name out"=w1068:refnum<visa-resource-name>)  [unwired: 8 out]
        n1016 = Initialize Array(u8 0 ("Numeric"), w1058) -> (w1057:u8[])
        n1017 = call <instrlib>:"Close.vi"("error in (no error)"=w1067, "VISA resource name"=w1068) -> ("error out"=w1069:errorcluster)  [unwired: 9 out]
        n1018 = local read "Array Mode"() -> (w1053:u16)
        n1019 = call "Arduino_a.vi"("Channel Number"=w1058, "error in (no error)"=w1035, "Current  Setting"=w1057, "Current Mode Count"=65535, "VISA Refnum in"=w1005) -> ("error out"=w1033:errorcluster, "VISA Refnum out"=w1034:refnum<visa-resource-name>)  [unwired: 5 in]
        n1020 = local read "Current Mode"() -> (w1059:u8[][])
        n1021 = case shown="True" w1021 {
          tunnel: w1030 -> [_ w1389]
          tunnel: w1061 -> [_ w1388]
          tunnel: w1031 -> [_ w1387]
          tunnel: w1032 -> [_ w1385]
          tunnel: w1010 -> [_ w1373]
          tunnel: w1059 -> [_ w1372]
          tunnel: path[] [] ("Attachments path") -> [w1368 w1371]
          tunnel: [w1368 w1369] -> w1048
          frame False {
          }
          frame True {
            n1022 = Strip Path(path=w1385) -> (stripped path=w1382:path, name=w1384:string)
            n1023 = Build Array (concatenate)(w1389, w1388, w1387) -> (w1386:dbl[][])
            n1024 = Concatenate Strings("Accurate_" ("string"), w1384) -> (w1381:string)
            n1025 = Strip Path(path=w1373) -> (stripped path=w1375:path, name=w1377:string)
            n1026 = Build Path(base path=w1382, name or relative path=w1381) -> (appended path=w1380:path)
            n1027 = call "Save Accurate Data only.vi"("appended array"=w1386, "configuration file path"=w1380) -> ("error out 2"=w1378:errorcluster, "file path"=w1379:path)  [unwired: 8 in]
            n1028 = Concatenate Strings("Accurate_" ("string"), w1377) -> (w1374:string)
            n1029 = Build Path(base path=w1375, name or relative path=w1374) -> (appended path=w1370:path)
            n1030 = Build Array (concatenate)(w1371, w1370) -> (w1369:path[])
            n1031 = call "Modified Data File Current Mode.vi"("Current Mode"=w1372, "modified data"=w1370, "original error"=w1378, "original data"=w1379) -> ()  [unwired: 6 in, 2 out]
          }
        }
        n1032 = case shown="True" "Save\nRaw Data" {
          tunnel: w1059 -> [_ w1316]
          tunnel: [w1308 w1315] -> w1056
          tunnel: [w1307 w1314] -> w1055
          tunnel: w1051 -> [w1307 w1313]
          tunnel: w1049 -> [w1308 w1311]
          tunnel: w1048 -> [w1306 w1312]
          tunnel: [w1306 w1310] -> w1047
          tunnel: w1010 -> [_ w1309]
          frame False {
          }
          frame True {
            n1033 = Build Array (concatenate)(w1312, w1309) -> (w1310:path[])
            n1034 = call "Modified Data File Current Mode_2.vi"("Current Mode"=w1316, "modified data"=w1309, "original error"=w1313, "original data"=w1311) -> ("original error out"=w1314:errorcluster, "original data out"=w1315:path)  [unwired: 4 in, 2 out]
          }
        }
        n1035 = stacked-sequence {
          tunnel: w1069 -> [w1365 _ _]
          frame #0 {
            n1036 = call <vilib>:"Simple Error Handler.vi"("error in (no error)"=w1365) -> ()  [unwired: 1 in, 8 out]
          }
          frame #1 {
            n1037 = local read "Remote\nPSU"() -> (w1366:bool)
            n1038 = case shown="True" w1366 {
              frame False {
              }
              frame True {
                n1039 = local write "PSU Enable"(FALSE ("PSU Enable")) -> ()
              }
            }
          }
          frame #2 {
            # "Remove prompt\nhere, so timer won't\nget stucked by\n\"OK\" button\n2023/12/19"
          }
        }
        n1040 = Greater?(x=w1053, y=u16 0) -> (0:w1054:bool)
        n1041 = case shown="True" w1054 {
          tunnel: w1056 -> [_ w1364]
          tunnel: w1055 -> [_ w1363]
          tunnel: w1010 -> [_ w1354]
          tunnel: w1053 -> [_ w1351]
          tunnel: w1047 -> [w1347 w1350]
          tunnel: [w1347 w1348] -> w1046
          frame False {
          }
          frame True {
            n1042 = local read "Electrode number, N"() -> (w1361:u16)
            n1043 = local read "Only Use Last Value?"() -> (w1360:bool)
            n1044 = local read "Inverse\nPolarity"() -> (w1359:bool)
            n1045 = Strip Path(path=w1354) -> (stripped path=w1353:path, name=w1356:string)
            n1046 = property on="Array Mode" class="Ring (strict)"() -> ("RingText.Text"=w1352:string)  [unwired: 2 in, 2 out]
            n1047 = local read "Current Mode"() -> (w1362:u8[][])
            n1048 = local read "Insert\nBreak"() -> (w1358:bool)
            n1049 = Concatenate Strings(w1352, "_" ("string"), w1356) -> (w1355:string)
            n1050 = Build Path(base path=w1353, name or relative path=w1355) -> (appended path=w1349:path)
            n1051 = call "Translate to Array Data_3.vi"("original data"=w1364, "Only Use Last Value?"=w1360, "Electrode number, N"=w1361, "Current Mode"=w1362, "original error"=w1363, "Array Mode"=w1351, "modified data"=w1349, "Inverse\nPolarity"=w1359, "Insert\nBreak"=w1358) -> ()  [unwired: 5 in, 2 out]
            n1052 = Build Array (concatenate)(w1350, w1349) -> (w1348:path[])
          }
        }
        n1053 = case shown="True" "Send data\nAutomatically" {
          tunnel: w1025 -> [_ w1320]
          tunnel: w1010 -> [_ w1319]
          tunnel: w1051 -> [_ w1318]
          tunnel: w1046 -> [_ w1317]
          frame False {
          }
          frame True {
            n1054 = flat-sequence {
              tunnel: w1320 -> [w1338]
              tunnel: w1319 -> [w1337]
              tunnel: w1318 -> [w1336]
              tunnel: w1317 -> [w1335]
              frame #0 {
                n1055 = Wait (ms)(milliseconds to wait=u32 100) -> ()  [unwired: 1 out]
              }
              frame #1 {
                n1056 = Unbundle By Name("Email Setting") -> ("server address"=w1330:string, "from"=w1329:string, "username"=w1328:string, "APP password"=w1327:string, "Receiver Email"=w1326:string, "subject"=w1325:string, "message"=w1324:string, "Attach data?"=w1322:bool)
                n1057 = case shown="True" w1338 {
                  tunnel: [w1343 "Failed_to_Get_" ("subject")] -> w1340
                  tunnel: [w1342 "lost DMM connection" ("message")] -> w1323
                  tunnel: [w1341 FALSE ("Attachment?")] -> w1334
                  tunnel: w1325 -> [w1343 _]
                  tunnel: w1324 -> [w1342 _]
                  tunnel: w1322 -> [w1341 _]
                  frame False {
                  }
                  frame True {
                  }
                }
                n1058 = Strip Path(path=w1337) -> (name=w1339:string)  [unwired: 1 out]
                n1059 = Concatenate Strings(w1340, w1339) -> (w1332:string)
                n1060 = call "Send data by Email_3.vi"("server address"=w1330, "subject"=w1332, "plain text message"=w1323, "to"=w1326, "from"=w1329, "username"=w1328, "APP password"=w1327, "error in"=w1336, "Attachments path"=w1335, "Attachment?"=w1334) -> ("error out"=w1333:errorcluster)  [unwired: 5 in]
                n1061 = call <vilib>:"Simple Error Handler.vi"("error in (no error)"=w1333) -> ()  [unwired: 4 in, 5 out]
              }
            }
          }
        }
      }
    }
    n1062 = local read "Leave"() -> (w353:bool)
    n1063 = local write "State"(w349) -> ()
  }
  n1064 = while {
    tunnel: [FALSE] -> w8
    stop <- w2720 stop-if-true
    n1065 = local read "ESP32 VISA"() -> (w2719:refnum<visa-resource-name>)
    n1066 = local read "ESP32 connect?"() -> (w2718:bool)
    n1067 = case shown="True" w2718 {
      tunnel: w2719 -> [_ w2722]
      frame False {
      }
      frame True {
        n1068 = while {
          shift-right: [w2724] -> _
          shift-left: w2722 -> [w2730]
          stop <- w2727 stop-if-true
          n1069 = property class="Instr"(reference=w2730) -> (reference out=w2726:refnum<visa-resource-name>, error out=w2725:errorcluster, "Bytes at Port"=w2723:u32)  [unwired: 1 in]
          n1070 = Equal?(x=w2723, y=u32 0) -> (x = y?=w2728:bool)
          n1071 = case shown="False" w2728 {
            tunnel: [FALSE TRUE] -> w2727
            tunnel: w2726 -> [w2741 w2743]
            tunnel: w2725 -> [w2740 _]
            tunnel: [w2739 w2743] -> w2724
            tunnel: w2723 -> [w2733 _]
            frame False {
              n1072 = VISA Read(VISA resource name=w2741, byte count=w2733, error in (no error)=w2740) -> (VISA resource name out=w2739:refnum<visa-resource-name>, read buffer=w2734:string, error out=w2731:errorcluster)  [unwired: 1 out]
              n1073 = call <vilib>:"Clear Errors.vi"("error in (no error)"=w2731, "specific error code to clear (0: all)"=-1073807339 ("code out")) -> ()  [unwired: 4 in, 2 out]
              n1074 = feedback #5("") -> (w2737:string)
              n1075 = Concatenate Strings(w2737, w2734) -> (w2738:string)
              "concatenated string 3" <- w2738
              n1076 = feedback-in #5(w2738) -> ()
              n1077 = property on="concatenated string 3" class="Str"("Text.Scroll Position"=inf) -> ()  [unwired: 2 in, 2 out]
            }
            frame True {
            }
          }
        }
      }
    }
    n1078 = Wait (ms)(milliseconds to wait=u32 10) -> ()  [unwired: 1 out]
    n1079 = local read "Leave"() -> (w2720:bool)
  }
  n1080 = while {
    shift-right: [w2748] -> _
    shift-left: FALSE ("PSU Enable") -> [w2747]
    tunnel: [FALSE ("PSU Enable")] -> w9
    stop <- w2745 stop-if-true
    n1081 = local read "PSU Enable"() -> (w2748:bool)
    n1082 = case shown="False" w2748 {
      tunnel: w2747 -> [w2751 _]
      tunnel: [w2750 FALSE ("Leave")] -> w2745
      frame False {
        n1083 = case shown="True" w2751 {
          frame False {
          }
          frame True {
            n1084 = local read "PSU(9184B)"() -> (w2752:refnum<visa-resource-name>)
            n1085 = call "PSU_close.vi"("VISA resource name"=w2752) -> ()  [unwired: 11 in]
          }
        }
        n1086 = local read "Leave"() -> (w2750:bool)
      }
      frame True {
        n1087 = local read "PSU(9184B)"() -> (w2759:refnum<visa-resource-name>)
        n1088 = VISA Write(VISA resource name=w2759, write buffer="IOUT?\n") -> (VISA resource name out=w2765:refnum<visa-resource-name>, error out=w2766:errorcluster)  [unwired: 1 in, 1 out]
        n1089 = VISA Read(VISA resource name=w2765, byte count=u32 256, error in (no error)=w2766) -> (VISA resource name out=w2770:refnum<visa-resource-name>, read buffer=→"PSU I":string, error out=w2757:errorcluster)  [unwired: 1 out]
        n1090 = call <vilib>:"Clear Errors.vi"("error in (no error)"=w2757, "specific error code to clear (0: all)"=-1073807339 ("code out")) -> ("error out"=w2756:errorcluster)  [unwired: 4 in, 1 out]
        n1091 = VISA Write(VISA resource name=w2770, write buffer="VOUT?\n", error in (no error)=w2756) -> (VISA resource name out=w2768:refnum<visa-resource-name>, error out=w2769:errorcluster)  [unwired: 1 out]
        n1092 = VISA Read(VISA resource name=w2768, byte count=u32 256, error in (no error)=w2769) -> (read buffer=→"PSU V":string, error out=w2754:errorcluster)  [unwired: 2 out]
        n1093 = call <vilib>:"Clear Errors.vi"("error in (no error)"=w2754, "specific error code to clear (0: all)"=-1073807339 ("code out")) -> ()  [unwired: 4 in, 2 out]
      }
    }
    n1094 = Wait (ms)(milliseconds to wait=u32 100) -> ()  [unwired: 1 out]
  }
  n1095 = local write "PSU Enable"(w9) -> ()
  n1096 = local write "ESP32 connect?"(w8) -> ()
  n1097 = Quit LabVIEW(quit? (T)=w14) -> ()
  n1098 = VISA Write(VISA resource name=w6, write buffer="L", error in (no error)=w15) -> (VISA resource name out=w5:refnum<visa-resource-name>, error out=w7:errorcluster)  [unwired: 1 out]
  n1099 = VISA Close(VISA resource name=w5, error in (no error)=w7) -> (error out=w3:errorcluster)
  n1100 = call <vilib>:"Simple Error Handler.vi"("type of dialog (OK msg:1)"=w2, "error in (no error)"=w3) -> ()  [unwired: 3 in, 5 out]
  "State" <- "Initialize" ("State")
  "State temp" <- "" ("State temp")
